vi "Beampointing_BELLA_PICObooster.vi"() -> ()   [LabVIEW 2013]
uses:
  shared programs/GUI_Template/GUI_master/tcp new data cluster.ctl
  <userlib>/_OpenG.lib/array/array.llb/Filter 1D Array with Scalar (String)__ogtk.vi
  <vilib>/Utility/file.llb/Write To Spreadsheet File (string).vi
  <vilib>/Utility/file.llb/Read From Spreadsheet File (string).vi
  <vilib>/Analysis/NI_AALBase.lvlib
  GUI_Beampointing_single_TRA/Ctrs/move.ctl
  Ctrs/beam detection.ctl
  <vilib>/vision/NI_Vision_Development_Module.lvlib
  shared programs/GUI_Template/GUI_master/tcp_new_data_event.ctl
panel:
  out "Array 3":sgl[](array[numeric])=[35.01637, 16.987305, 27.281555, 56.5656, 0.0, 12.310791, 0.0, 0.0, 0.0, 0.0, 0.0, 0.0]
  in  "save path":path=path "W:/BP_DATA"
  out "size(s) 6":i32=12
  out "config path":string="H:\\Software\\control-all-loasis\\Developers Version\\Interface\\builds\\GUIs\\GUI_Beampointing_PicoBooster\\20160427BELLA.cfg"
  out "motor refs 7":refnum<vi>[](array[refnum])
  out "Moving Y":string
  out "Moving X":string
  out "particles":T1(array[cluster])=[{"Area"=13625.0, "Number of Holes"=0.0, "Bounding Rect"={"Left"=100.0, "Top"=93.0, "Right"=241.0, "Bottom"=225.0}, "Center of Mass"={"X"=171.3850275229358, "Y"=158.37277064220183}, "Orientation"=31.450434142859965, "Dimensions"={"Width"=141.0, "Height"=132.0}}]
  out "motor refs 6":refnum<vi>[](array[refnum])
  out "millisecond timer value":u32=150056294
  out "motor refs 5":refnum<vi>[](array[refnum])
  out "appended path":path=path "C:/Users/loasis.BELLANET/Documents/000 Labview/Developers Version/Interface/GUI_Beampointing_multi/defaultDevices_PICObooster.txt"
  out "motor refs 4":refnum<vi>[](array[refnum])
  in  "active Axis ref 3":cluster{"Ref X":refnum<vi>, "Ref Y":refnum<vi>}
  out "motor refs 3":refnum<vi>[](array[refnum])
  in  "active man refs":cluster{"Ref X":refnum<vi>, "Ref Y":refnum<vi>}
  out "motor refs 2":refnum<vi>[](array[refnum])
  in  "Numeric":dbl=2.0
  out "Current State":string="Exit"
  in  "output cluster 2":T5 {"detection para"."smal para"."Measurement Parameter" items=["Center of Mass X", "Center of Mass Y", "First Pixel X", "First Pixel Y", "Bounding Rect Left", "Bounding Rect Top", "Bounding Rect Right", "Bounding Rect Bottom", "Max Feret Diameter Start X", "Max Feret Diameter Start Y", "Max Feret Diameter End X", "Max Feret Diameter End Y", "Max Horiz. Segment Length Left", "Max Horiz. Segment Length Right", "Max Horiz. Segment Length Row", "-", "Bounding Rect Width", "Bounding Rect Height", "Bounding Rect Diagonal", "Perimeter", "Convex Hull Perimeter", "Holes' Perimeter", "Max Feret Diameter", "Equivalent Ellipse Major Axis", "Equivalent Ellipse Minor Axis", "Equivalent Ellipse Minor Axis (Feret)", "Equivalent Rect Long Side", "Equivalent Rect Short Side", "Equivalent Rect Diagonal", "Equivalent Rect Short Side (Feret)", "Average Horiz. Segment Length", "Average Vert. Segment Length", "Hydraulic Radius", "Waddel Disk Diameter", "-", "Area", "Holes' Area", "Particle & Holes' Area", "Convex Hull Area", "Image Area", "-", "Number of Holes", "Number of Horiz. Segments", "Number of Vert. Segments", "-", "Orientation", "Max Feret Diameter Orientation", "-", "% Area/Image Area", "% Area/(Particle & Holes' Area)", "Ratio of Equivalent Ellipse Axes", "Ratio of Equivalent Rect Sides", "-", "Elongation Factor", "Compactness Factor", "Heywood Circularity Factor", "Type Factor", "-", "Sum X", "Sum Y", "Sum XX", "Sum XY", "Sum YY", "Sum XXX", "Sum XXY", "Sum XYY", "Sum YYY", "-", "Moment of Inertia XX", "Moment of Inertia XY", "Moment of Inertia YY", "Moment of Inertia XXX", "Moment of Inertia XXY", "Moment of Inertia XYY", "Moment of Inertia YYY", "Norm. Moment of Inertia XX", "Norm. Moment of Inertia XY", "Norm. Moment of Inertia YY", "Norm. Moment of Inertia XXX", "Norm. Moment of Inertia XXY", "Norm. Moment of Inertia XYY", "Norm. Moment of Inertia YYY", "Hu Moment 1", "Hu Moment 2", "Hu Moment 3", "Hu Moment 4", "Hu Moment 5", "Hu Moment 6", "Hu Moment 7"]; "detection para"."smal para"."Range Lower Value" format="%.2f"; "detection para"."smal para"."Range Upper Value" format="%.2f"; "detection para"."detection method" items=["clustering", "entropy", "metric", "moments", "inter-class variance"]; "detection para"."Filter" items=["No Filter", "Median Filter", "Low Pass Filter"]}
  out "CCDs":string[](array[string])=["RegenCam", "BoosterCam", "PreampCam", "Amp1Cam", "Amp2Cam", "Amp3Cam", "", "", "", "", "", ""]
  in  "GUIdevice 12":string
  in  "GUIdevice 11":string
  in  "GUIdevice 10":string
  in  "GUIdevice 9":string
  out "error out 2":errorcluster
  in  "active cams":string[](array[string])
  in  "Motor Y":dbl[][](array[numeric])
  in  "Motor X":dbl[][](array[numeric])
  out "Names":string[](array[string])=["device12", "device45", "", ""]
  in  "Offset X stats":dbl[][](array[numeric])
  in  "Offset Y stats":dbl[][](array[numeric])
  out "Box":T6(array[cluster])=[{"Left"=100.0, "Top"=93.0, "Right"=241.0, "Bottom"=225.0}, {"Left"=87.0, "Top"=22.0, "Right"=220.0, "Bottom"=185.0}, {"Left"=80.0, "Top"=37.0, "Right"=220.0, "Bottom"=176.0}, {"Left"=78.0, "Top"=52.0, "Right"=221.0, "Bottom"=209.0}, {"Left"=0.0, "Top"=0.0, "Right"=0.0, "Bottom"=0.0}]
  in  "Tab Control 2":enum32{"Config ", "Main", "History"}(tab)=enum."Main"
  in  "associated motors":T7={"Motor CCD 1"=0, "Motor CCD 2"=0, "Motor CCD 3"=1, "Motor CCD 4"=0, "Motor CCD 5"=0, "Motor CCD 6"=0, "Motor CCD 7"=0, "Motor CCD 8"=0, "Motor CCD 9"=0, "Motor CCD 10"=0, "Motor CCD 11"=0, "Motor CCD 12"=0} {"Motor CCD 12" items=["device12", "device45", "", ""]; "Motor CCD 11" items=["device12", "device45", "", ""]; "Motor CCD 10" items=["device12", "device45", "", ""]; "Motor CCD 9" items=["device12", "device45", "", ""]; "Motor CCD 8" items=["device12", "device45", "", ""]; "Motor CCD 7" items=["device12", "device45", "", ""]; "Motor CCD 6" items=["device12", "device45", "", ""]; "Motor CCD 5" items=["device12", "device45", "", ""]; "Motor CCD 4" items=["device12", "device45", "", ""]; "Motor CCD 3" items=["device12", "device45", "", ""]; "Motor CCD 2" items=["device12", "device45", "", ""]; "Motor CCD 1" items=["device12", "device45", "", ""]}
  out "Cameras":T8={"[0]"="RegenCam", "[1]"="BoosterCam", "[2]"="PreampCam", "[3]"="Amp1Cam", "[4]"="Amp2Cam", "[5]"="Amp3Cam", "[6]"="", "[7]"="", "[8]"="", "[8] 2"="", "[8] 3"="", "[8] 4"=""}
  out "Status":cluster{i32, i32, "Centroid X":dbl[][]}(graph)={0, 1, "Centroid X"=[[171.87383691112902, 0.0, 0.0], [153.80799798158193, 0.0, 0.0], [147.97157969527117, 0.0, 0.0], [147.97285865350722, 0.0, 0.0], [0.0, 0.0, 0.0], [0.0, 0.0, 0.0], [0.0, 0.0, 0.0], [0.0, 0.0, 0.0], [0.0, 0.0, 0.0], [0.0, 0.0, 0.0], [0.0, 0.0, 0.0], [0.0, 0.0, 0.0]]}
  in  "Exposure:12":dbl=0.095 min=0.0001 max=1.0 format="%#_6f"
  in  "Triggerdelay::12":dbl=0.003 min=0.0 max=0.09 format="%#_6f"
  in  "Exposure::11":dbl=0.095 min=0.0001 max=1.0 format="%#_6f"
  in  "Triggerdelay::11":dbl=0.003 min=0.0 max=0.09 format="%#_6f"
  in  "Exposure::10":dbl=0.095 min=0.0001 max=1.0 format="%#_6f"
  in  "Triggerdelay::10":dbl=0.003 min=0.0 max=0.09 format="%#_6f"
  in  "Exposure::9":dbl=0.095 min=0.0001 max=1.0 format="%#_6f"
  in  "Triggerdelay::9":dbl=0.003 min=0.0 max=0.09 format="%#_6f"
  in  "Trigger::9":bool
  in  "Trigger::10":bool caption="Trigger:10"
  in  "Trigger::11":bool
  in  "Trigger::12":bool
  in  "Target.Y::9":dbl=45.0 caption="T9y" min=0.0 max=2000.0 format="%#_6f"
  in  "Target.X::9":dbl=47.0 caption="Tx9" min=0.0 max=2000.0 format="%#_6f"
  in  "Target.Y::10":dbl=45.0 caption="T10y" min=0.0 max=2000.0 format="%#_6f"
  in  "Target.X::10":dbl=47.0 caption="T10x" min=0.0 max=2000.0 format="%#_6f"
  in  "Target.Y::11":dbl=45.0 caption="T11y" min=0.0 max=2000.0 format="%#_6f"
  in  "Target.X::11":dbl=47.0 caption="T11x" min=0.0 max=2000.0 format="%#_6f"
  in  "Target.Y::12":dbl=45.0 caption="T12y" min=0.0 max=2000.0 format="%#_6f"
  in  "Target.X::12":dbl=47.0 caption="T12x" min=0.0 max=2000.0 format="%#_6f"
  in  "Exposure::8":dbl=0.095 min=0.0001 max=1.0 format="%#_6f"
  in  "Triggerdelay::8":dbl=0.003 min=0.0 max=0.09 format="%#_6f"
  in  "Trigger::8":bool
  in  "Target.Y::8":dbl=45.0 caption="T8y" min=0.0 max=2000.0 format="%#_6f"
  in  "Target.X::8":dbl=47.0 caption="T8x" min=0.0 max=2000.0 format="%#_6f"
  in  "Target.Y::7":dbl=45.0 caption="T7x" min=0.0 max=2000.0 format="%#_6f"
  in  "Target.X::7":dbl=47.0 caption="T7y" min=0.0 max=2000.0 format="%#_6f"
  in  "Target.Y::6":dbl=142.0 caption="T6y" min=0.0 max=5000.0 format="%#_6f"
  in  "Target.X::6":dbl=123.0 caption="T6x" min=0.0 max=5000.0 format="%#_6f"
  in  "Target.Y::5":dbl=108.0 caption="T5y" min=0.0 max=5000.0 format="%#_6f"
  in  "Target.X::5":dbl=172.0 caption="T5x" min=0.0 max=5000.0 format="%#_6f"
  in  "Target.Y::4":dbl=130.0 caption="T4y" min=0.0 max=5000.0 format="%#_6f"
  in  "Target.X::4":dbl=148.0 caption="T4x" min=0.0 max=5000.0 format="%#_6f"
  in  "Target.Y::3":dbl=110.0 caption="T3y" min=0.0 max=5000.0 format="%#_6f"
  in  "Target.X::3":dbl=154.0 caption="T3x" min=0.0 max=5000.0 format="%#_6f"
  in  "Target.Y::2":dbl=106.0 caption="T2y" min=0.0 max=5000.0 format="%#_6f"
  in  "Target.X::2":dbl=163.0 caption="T2x" min=0.0 max=5000.0 format="%#_6f"
  in  "Target.Y::1":dbl=162.0 caption="T1y" min=0.0 max=5000.0 format="%#_6f"
  in  "Target.X::1":dbl=171.0 caption="T1x" min=0.0 max=5000.0 format="%#_6f"
  in  "Exposure::7":dbl=0.095 min=3.8e-05 max=1.0 format="%#_6f"
  in  "Triggerdelay::7":dbl=0.003 min=0.0 max=0.09 format="%#_6f"
  in  "Trigger::7":bool
  in  "Exposure::6":dbl=0.095 min=3.8e-05 max=1.0 format="%#_6f"
  in  "Triggerdelay::6":dbl=0.003 min=0.0 max=0.09 format="%#_6f"
  in  "Trigger::6":bool
  in  "Exposure::5":dbl=0.095 min=0.0001 max=1.0 format="%#_6f"
  in  "Triggerdelay::5":dbl=0.003 min=0.0 max=0.09 format="%#_6f"
  in  "Trigger::5":bool
  in  "Exposure::4":dbl=0.095 min=0.0001 max=1.0 format="%#_6f"
  in  "Triggerdelay::4":dbl=0.003 min=0.0 max=0.09 format="%#_6f"
  in  "Trigger::4":bool
  in  "Exposure::3":dbl=0.095 min=3.8e-05 max=1.0 format="%#_6f"
  in  "Triggerdelay::3":dbl=0.003 min=0.0 max=0.09 format="%#_6f"
  in  "Trigger::3":bool
  in  "Exposure::2":dbl=0.095 min=3.8e-05 max=1.0 format="%#_6f"
  in  "Triggerdelay::2":dbl=0.003 min=0.0 max=0.09 format="%#_6f"
  in  "Trigger::2":bool
  out "image::1":T9(plugin-control) caption="RegenCam"
  out "image::2":T9(plugin-control) caption="BoosterCam"
  out "image::3":T9(plugin-control) caption="PreampCam"
  out "image::4":T9(plugin-control) caption="Amp1Cam"
  out "image::5":T9(plugin-control) caption="Amp2Cam"
  out "image::6":T9(plugin-control) caption="Amp3Cam"
  out "image::7":T9(plugin-control)
  out "image::8":T9(plugin-control)
  in  "Exposure::1":dbl=0.095 min=3.8e-05 max=1.0 format="%#_6f"
  in  "Triggerdelay::1":dbl=0.003 min=0.0 max=0.09 format="%#_6f"
  in  "Trigger::1":bool
  in  "UDP error message":string
  out "required Y":bool[](array[boolean])=[FALSE, TRUE, FALSE, FALSE, FALSE]
  out "required X":bool[](array[boolean])=[FALSE, TRUE, FALSE, FALSE, FALSE]
  out "detected":bool[](array[boolean])=[TRUE, TRUE, TRUE, TRUE, FALSE]
  out "name array":string[](array[string])=["RegenCam", "BoosterCam", "PreampCam", "Amp1Cam", "Amp3Cam"]
  out "image::9":T9(plugin-control)
  out "image::10":T9(plugin-control)
  out "image::11":T9(plugin-control)
  out "image::12":T9(plugin-control)
  out "speedmode X":bool[](array[boolean])=[TRUE, TRUE, TRUE, TRUE, FALSE]
  out "speedmode Y":bool[](array[boolean])=[TRUE, FALSE, TRUE, TRUE, FALSE]
  out "CCD 9":cluster{timestamp[], dbl[]}[](graph)=[{[timestamp(3549547983.3591223 s since 1904-01-01)], [0.0]}, {[timestamp(3549547983.3591223 s since 1904-01-01)], [0.0]}, {[timestamp(3549547983.3591223 s since 1904-01-01)], [20.0]}, {[timestamp(3549547983.3591223 s since 1904-01-01)], [-20.0, -20.0, -20.0, -20.0]}]
  out "CCD 10":cluster{timestamp[], dbl[]}[](graph)=[{[timestamp(3549547983.360123 s since 1904-01-01)], [0.0]}, {[timestamp(3549547983.360123 s since 1904-01-01)], [0.0]}, {[timestamp(3549547983.360123 s since 1904-01-01)], [20.0]}, {[timestamp(3549547983.360123 s since 1904-01-01)], [-20.0, -20.0, -20.0, -20.0]}]
  out "CCD 11":cluster{timestamp[], dbl[]}[](graph)=[{[timestamp(3549547983.360123 s since 1904-01-01)], [0.0]}, {[timestamp(3549547983.360123 s since 1904-01-01)], [0.0]}, {[timestamp(3549547983.360123 s since 1904-01-01)], [20.0]}, {[timestamp(3549547983.360123 s since 1904-01-01)], [-20.0, -20.0, -20.0, -20.0]}]
  out "CCD 12":cluster{timestamp[], dbl[]}[](graph)=[{[timestamp(3549547983.360123 s since 1904-01-01)], [0.0]}, {[timestamp(3549547983.360123 s since 1904-01-01)], [0.0]}, {[timestamp(3549547983.360123 s since 1904-01-01)], [20.0]}, {[timestamp(3549547983.360123 s since 1904-01-01)], [-20.0, -20.0, -20.0, -20.0]}]
  out "CCD 5":cluster{timestamp[], dbl[]}[](graph)=[{[timestamp(3549547983.358122 s since 1904-01-01)], [0.0]}, {[timestamp(3549547983.358122 s since 1904-01-01)], [0.0]}, {[timestamp(3549547983.358122 s since 1904-01-01)], [20.0]}, {[timestamp(3549547983.358122 s since 1904-01-01)], [-20.0, -20.0, -20.0, -20.0]}]
  out "CCD 6":cluster{timestamp[], dbl[]}[](graph)=[{[timestamp(3549547983.3591223 s since 1904-01-01)], [0.0]}, {[timestamp(3549547983.3591223 s since 1904-01-01)], [0.0]}, {[timestamp(3549547983.3591223 s since 1904-01-01)], [20.0]}, {[timestamp(3549547983.3591223 s since 1904-01-01)], [-20.0, -20.0, -20.0, -20.0]}]
  out "CCD 7":cluster{timestamp[], dbl[]}[](graph)=[{[timestamp(3549547983.3591223 s since 1904-01-01)], [0.0]}, {[timestamp(3549547983.3591223 s since 1904-01-01)], [0.0]}, {[timestamp(3549547983.3591223 s since 1904-01-01)], [20.0]}, {[timestamp(3549547983.3591223 s since 1904-01-01)], [-20.0, -20.0, -20.0, -20.0]}]
  out "CCD 8":cluster{timestamp[], dbl[]}[](graph)=[{[timestamp(3549547983.3591223 s since 1904-01-01)], [0.0]}, {[timestamp(3549547983.3591223 s since 1904-01-01)], [0.0]}, {[timestamp(3549547983.3591223 s since 1904-01-01)], [20.0]}, {[timestamp(3549547983.3591223 s since 1904-01-01)], [-20.0, -20.0, -20.0, -20.0]}]
  out "CCD 2":cluster{timestamp[], dbl[]}[](graph)=[{[timestamp(3549547983.358122 s since 1904-01-01)], [3.0783937413765585]}, {[timestamp(3549547983.358122 s since 1904-01-01)], [8.883046862591215]}, {[timestamp(3549547983.358122 s since 1904-01-01)], [20.0]}, {[timestamp(3549547983.358122 s since 1904-01-01)], [-20.0, -20.0, -20.0, -20.0]}]
  out "CCD 1":cluster{timestamp[], dbl[]}[](graph)=[{[timestamp(3549547983.357121 s since 1904-01-01)], [3.1654865062995725]}, {[timestamp(3549547983.357121 s since 1904-01-01)], [-0.42630614615123363]}, {[timestamp(3549547983.357121 s since 1904-01-01)], [20.0]}, {[timestamp(3549547983.357121 s since 1904-01-01)], [-20.0, -20.0, -20.0, -20.0]}]
  out "CCD 3":cluster{timestamp[], dbl[]}[](graph)=[{[timestamp(3549547983.358122 s since 1904-01-01)], [5.607599326451648]}, {[timestamp(3549547983.358122 s since 1904-01-01)], [4.73033759911138]}, {[timestamp(3549547983.358122 s since 1904-01-01)], [0.0]}, {[timestamp(3549547983.358122 s since 1904-01-01)], [0.0, 0.0, 0.0, 0.0]}]
  out "CCD 4":cluster{timestamp[], dbl[]}[](graph)=[{[timestamp(3549547983.358122 s since 1904-01-01)], [1.2734976836249814]}, {[timestamp(3549547983.358122 s since 1904-01-01)], [-0.6350086940318818]}, {[timestamp(3549547983.358122 s since 1904-01-01)], [20.0]}, {[timestamp(3549547983.358122 s since 1904-01-01)], [-20.0, -20.0, -20.0, -20.0]}]
  in  "History Size":i32=2000
  out "History Index":i32=1
  in  "Feedback Global":bool
  in  "detection para":T3[](array[typedef])=[{"Filter"=1, "Filter Para"={"X Size"=5, "Y Size"=5, "% Tolerance"=1}, "detection method"=4, "smal para"=[{"Measurement Parameter"=35, "Range Lower Value"=0.0, "Range Upper Value"=0.0, "Range"=TRUE, "Measurement Type"=FALSE}], "Remove small Objects"=TRUE, "Restrict to round Objects"=FALSE}, {"Filter"=1, "Filter Para"={"X Size"=5, "Y Size"=5, "% Tolerance"=1}, "detection method"=4, "smal para"=[{"Measurement Parameter"=35, "Range Lower Value"=0.0, "Range Upper Value"=500.0, "Range"=FALSE, "Measurement Type"=FALSE}], "Remove small Objects"=TRUE, "Restrict to round Objects"=FALSE}, {"Filter"=1, "Filter Para"={"X Size"=5, "Y Size"=5, "% Tolerance"=1}, "detection method"=4, "smal para"=[{"Measurement Parameter"=35, "Range Lower Value"=0.0, "Range Upper Value"=500.0, "Range"=TRUE, "Measurement Type"=FALSE}], "Remove small Objects"=TRUE, "Restrict to round Objects"=FALSE}, {"Filter"=1, "Filter Para"={"X Size"=5, "Y Size"=5, "% Tolerance"=1}, "detection method"=4, "smal para"=[{"Measurement Parameter"=35, "Range Lower Value"=0.0, "Range Upper Value"=500.0, "Range"=TRUE, "Measurement Type"=FALSE}], "Remove small Objects"=TRUE, "Restrict to round Objects"=FALSE}, {"Filter"=1, "Filter Para"={"X Size"=5, "Y Size"=5, "% Tolerance"=1}, "detection method"=4, "smal para"=[{"Measurement Parameter"=35, "Range Lower Value"=0.0, "Range Upper Value"=500.0, "Range"=TRUE, "Measurement Type"=FALSE}], "Remove small Objects"=TRUE, "Restrict to round Objects"=FALSE}, {"Filter"=1, "Filter Para"={"X Size"=5, "Y Size"=5, "% Tolerance"=1}, "detection method"=4, "smal para"=[{"Measurement Parameter"=35, "Range Lower Value"=0.0, "Range Upper Value"=500.0, "Range"=TRUE, "Measurement Type"=FALSE}], "Remove small Objects"=TRUE, "Restrict to round Objects"=FALSE}, {"Filter"=1, "Filter Para"={"X Size"=5, "Y Size"=5, "% Tolerance"=1}, "detection method"=4, "smal para"=[{"Measurement Parameter"=35, "Range Lower Value"=0.0, "Range Upper Value"=500.0, "Range"=TRUE, "Measurement Type"=FALSE}], "Remove small Objects"=TRUE, "Restrict to round Objects"=FALSE}, {"Filter"=1, "Filter Para"={"X Size"=5, "Y Size"=5, "% Tolerance"=1}, "detection method"=3, "smal para"=[{"Measurement Parameter"=35, "Range Lower Value"=0.0, "Range Upper Value"=0.0, "Range"=FALSE, "Measurement Type"=FALSE}], "Remove small Objects"=TRUE, "Restrict to round Objects"=FALSE}, {"Filter"=1, "Filter Para"={"X Size"=5, "Y Size"=5, "% Tolerance"=1}, "detection method"=4, "smal para"=[{"Measurement Parameter"=35, "Range Lower Value"=0.0, "Range Upper Value"=0.0, "Range"=FALSE, "Measurement Type"=FALSE}], "Remove small Objects"=TRUE, "Restrict to round Objects"=FALSE}, {"Filter"=1, "Filter Para"={"X Size"=5, "Y Size"=5, "% Tolerance"=1}, "detection method"=4, "smal para"=[{"Measurement Parameter"=35, "Range Lower Value"=0.0, "Range Upper Value"=500.0, "Range"=TRUE, "Measurement Type"=FALSE}], "Remove small Objects"=TRUE, "Restrict to round Objects"=FALSE}, {"Filter"=1, "Filter Para"={"X Size"=5, "Y Size"=5, "% Tolerance"=1}, "detection method"=4, "smal para"=[{"Measurement Parameter"=35, "Range Lower Value"=0.0, "Range Upper Value"=500.0, "Range"=TRUE, "Measurement Type"=FALSE}], "Remove small Objects"=TRUE, "Restrict to round Objects"=FALSE}, {"Filter"=1, "Filter Para"={"X Size"=5, "Y Size"=5, "% Tolerance"=1}, "detection method"=4, "smal para"=[{"Measurement Parameter"=35, "Range Lower Value"=0.0, "Range Upper Value"=500.0, "Range"=TRUE, "Measurement Type"=FALSE}], "Remove small Objects"=TRUE, "Restrict to round Objects"=FALSE}] {"smal para"."Measurement Parameter" items=["Center of Mass X", "Center of Mass Y", "First Pixel X", "First Pixel Y", "Bounding Rect Left", "Bounding Rect Top", "Bounding Rect Right", "Bounding Rect Bottom", "Max Feret Diameter Start X", "Max Feret Diameter Start Y", "Max Feret Diameter End X", "Max Feret Diameter End Y", "Max Horiz. Segment Length Left", "Max Horiz. Segment Length Right", "Max Horiz. Segment Length Row", "-", "Bounding Rect Width", "Bounding Rect Height", "Bounding Rect Diagonal", "Perimeter", "Convex Hull Perimeter", "Holes' Perimeter", "Max Feret Diameter", "Equivalent Ellipse Major Axis", "Equivalent Ellipse Minor Axis", "Equivalent Ellipse Minor Axis (Feret)", "Equivalent Rect Long Side", "Equivalent Rect Short Side", "Equivalent Rect Diagonal", "Equivalent Rect Short Side (Feret)", "Average Horiz. Segment Length", "Average Vert. Segment Length", "Hydraulic Radius", "Waddel Disk Diameter", "-", "Area", "Holes' Area", "Particle & Holes' Area", "Convex Hull Area", "Image Area", "-", "Number of Holes", "Number of Horiz. Segments", "Number of Vert. Segments", "-", "Orientation", "Max Feret Diameter Orientation", "-", "% Area/Image Area", "% Area/(Particle & Holes' Area)", "Ratio of Equivalent Ellipse Axes", "Ratio of Equivalent Rect Sides", "-", "Elongation Factor", "Compactness Factor", "Heywood Circularity Factor", "Type Factor", "-", "Sum X", "Sum Y", "Sum XX", "Sum XY", "Sum YY", "Sum XXX", "Sum XXY", "Sum XYY", "Sum YYY", "-", "Moment of Inertia XX", "Moment of Inertia XY", "Moment of Inertia YY", "Moment of Inertia XXX", "Moment of Inertia XXY", "Moment of Inertia XYY", "Moment of Inertia YYY", "Norm. Moment of Inertia XX", "Norm. Moment of Inertia XY", "Norm. Moment of Inertia YY", "Norm. Moment of Inertia XXX", "Norm. Moment of Inertia XXY", "Norm. Moment of Inertia XYY", "Norm. Moment of Inertia YYY", "Hu Moment 1", "Hu Moment 2", "Hu Moment 3", "Hu Moment 4", "Hu Moment 5", "Hu Moment 6", "Hu Moment 7"]; "smal para"."Range Lower Value" format="%.2f"; "smal para"."Range Upper Value" format="%.2f"; "detection method" items=["clustering", "entropy", "metric", "moments", "inter-class variance"]; "Filter" items=["No Filter", "Median Filter", "Low Pass Filter"]}
  in  "GUIdevice 8":string
  in  "Tab Control":T10(tab)
  in  "new tdms":bool
  in  "Save Stats":bool
  in  "Save Config":bool
  in  "Load Config":bool
  in  "update speed [ms]":i32=2000
  in  "img to avg":i32=6 min=3 max=200
  in  "Reset History":bool
  in  "autodetect":bool
  in  "Detection Rate":dbl=0.8 min=0.001 max=1.0
  in  "Center":bool
  in  "Align":bool
  in  "Speedmode @":dbl=3.0 min=1.0 max=20.0
  in  "device ini":bool
  in  "beam detection para":T3={"Filter"=1, "Filter Para"={"X Size"=5, "Y Size"=5, "% Tolerance"=1}, "detection method"=4, "smal para"=[{"Measurement Parameter"=35, "Range Lower Value"=0.0, "Range Upper Value"=500.0, "Range"=FALSE, "Measurement Type"=FALSE}], "Remove small Objects"=TRUE, "Restrict to round Objects"=FALSE} {"smal para"."Measurement Parameter" items=["Center of Mass X", "Center of Mass Y", "First Pixel X", "First Pixel Y", "Bounding Rect Left", "Bounding Rect Top", "Bounding Rect Right", "Bounding Rect Bottom", "Max Feret Diameter Start X", "Max Feret Diameter Start Y", "Max Feret Diameter End X", "Max Feret Diameter End Y", "Max Horiz. Segment Length Left", "Max Horiz. Segment Length Right", "Max Horiz. Segment Length Row", "-", "Bounding Rect Width", "Bounding Rect Height", "Bounding Rect Diagonal", "Perimeter", "Convex Hull Perimeter", "Holes' Perimeter", "Max Feret Diameter", "Equivalent Ellipse Major Axis", "Equivalent Ellipse Minor Axis", "Equivalent Ellipse Minor Axis (Feret)", "Equivalent Rect Long Side", "Equivalent Rect Short Side", "Equivalent Rect Diagonal", "Equivalent Rect Short Side (Feret)", "Average Horiz. Segment Length", "Average Vert. Segment Length", "Hydraulic Radius", "Waddel Disk Diameter", "-", "Area", "Holes' Area", "Particle & Holes' Area", "Convex Hull Area", "Image Area", "-", "Number of Holes", "Number of Horiz. Segments", "Number of Vert. Segments", "-", "Orientation", "Max Feret Diameter Orientation", "-", "% Area/Image Area", "% Area/(Particle & Holes' Area)", "Ratio of Equivalent Ellipse Axes", "Ratio of Equivalent Rect Sides", "-", "Elongation Factor", "Compactness Factor", "Heywood Circularity Factor", "Type Factor", "-", "Sum X", "Sum Y", "Sum XX", "Sum XY", "Sum YY", "Sum XXX", "Sum XXY", "Sum XYY", "Sum YYY", "-", "Moment of Inertia XX", "Moment of Inertia XY", "Moment of Inertia YY", "Moment of Inertia XXX", "Moment of Inertia XXY", "Moment of Inertia XYY", "Moment of Inertia YYY", "Norm. Moment of Inertia XX", "Norm. Moment of Inertia XY", "Norm. Moment of Inertia YY", "Norm. Moment of Inertia XXX", "Norm. Moment of Inertia XXY", "Norm. Moment of Inertia XYY", "Norm. Moment of Inertia YYY", "Hu Moment 1", "Hu Moment 2", "Hu Moment 3", "Hu Moment 4", "Hu Moment 5", "Hu Moment 6", "Hu Moment 7"]; "smal para"."Range Lower Value" format="%.2f"; "smal para"."Range Upper Value" format="%.2f"; "detection method" items=["clustering", "entropy", "metric", "moments", "inter-class variance"]; "Filter" items=["No Filter", "Median Filter", "Low Pass Filter"]}
  in  "move config":T2={"Tolerance [%]"=0.1, "Stepsize"=0.0001, "Invert Axis"=TRUE, "Invert Direction X"=FALSE, "Invert Direction Y"=TRUE, "enable feedback"=FALSE, "Set Centriod Target"=FALSE}
  in  "Position 2":dbl=-20.0 caption="Stepsize" min=0.0 max=999999.0 format="%_6f"
  in  "Position 1":dbl=20.0 caption="Stepsize" min=0.0 max=999999.0 format="%_6f"
  in  "Right":bool caption="RelativeMove.Axis 1.CCW::1"
  in  "Left":bool caption="RelativeMove.Axis 1.CW::1"
  in  "Down":bool caption="RelativeMove.Axis. 2.CCW::1"
  in  "Up":bool caption="RelativeMove.Axis 2.CW::1"
  in  "StepSize":i16=5 caption="Stepsize" min=0 max=500 step=1
  in  "active axis refs 2":T11(array[cluster])
  in  "active Axis ref":cluster{"Ref X":refnum<vi>, "Ref Y":refnum<vi>}
  in  "CCDs":u16(ring) items=["RegenCam", "BoosterCam", "PreampCam", "Amp1Cam", "Amp2Cam", "Amp3Cam", "", "", "", "", "", ""]
  out "motor refs":refnum<vi>[](array[refnum])
  in  "Position.device 4::99":dbl caption="Motor Axis 1" min=-1000.0 max=1000.0 format="%#_6f"
  in  "Position.device 5::99":dbl caption="Motor Axis 1" min=-1000.0 max=1000.0 format="%#_6f"
  in  "Position.device 2::99":dbl=-20.0 caption="Motor Axis 1" min=-10000.0 max=10000.0 format="%#_6f"
  in  "Position.device 1::99":dbl=20.0 caption="Motor Axis 1" min=-10000.0 max=10000.0 format="%#_6f"
  in  "GUIdevice 99":string="LB-Pico-Booster"
  in  "move properties":T2[](array[typedef])=[{"Tolerance [%]"=0.1, "Stepsize"=0.0001, "Invert Axis"=TRUE, "Invert Direction X"=FALSE, "Invert Direction Y"=TRUE, "enable feedback"=FALSE, "Set Centriod Target"=FALSE}, {"Tolerance [%]"=0.1, "Stepsize"=0.0001, "Invert Axis"=TRUE, "Invert Direction X"=FALSE, "Invert Direction Y"=TRUE, "enable feedback"=FALSE, "Set Centriod Target"=FALSE}, {"Tolerance [%]"=0.1, "Stepsize"=0.0001, "Invert Axis"=TRUE, "Invert Direction X"=FALSE, "Invert Direction Y"=TRUE, "enable feedback"=FALSE, "Set Centriod Target"=FALSE}, {"Tolerance [%]"=0.1, "Stepsize"=0.0001, "Invert Axis"=TRUE, "Invert Direction X"=FALSE, "Invert Direction Y"=TRUE, "enable feedback"=FALSE, "Set Centriod Target"=FALSE}, {"Tolerance [%]"=0.1, "Stepsize"=0.0001, "Invert Axis"=TRUE, "Invert Direction X"=FALSE, "Invert Direction Y"=TRUE, "enable feedback"=FALSE, "Set Centriod Target"=FALSE}, {"Tolerance [%]"=0.1, "Stepsize"=0.0001, "Invert Axis"=TRUE, "Invert Direction X"=FALSE, "Invert Direction Y"=TRUE, "enable feedback"=FALSE, "Set Centriod Target"=FALSE}, {"Tolerance [%]"=0.1, "Stepsize"=0.0001, "Invert Axis"=TRUE, "Invert Direction X"=FALSE, "Invert Direction Y"=TRUE, "enable feedback"=FALSE, "Set Centriod Target"=FALSE}, {"Tolerance [%]"=0.1, "Stepsize"=0.0001, "Invert Axis"=TRUE, "Invert Direction X"=FALSE, "Invert Direction Y"=TRUE, "enable feedback"=FALSE, "Set Centriod Target"=FALSE}, {"Tolerance [%]"=0.1, "Stepsize"=0.0001, "Invert Axis"=TRUE, "Invert Direction X"=FALSE, "Invert Direction Y"=TRUE, "enable feedback"=FALSE, "Set Centriod Target"=FALSE}, {"Tolerance [%]"=0.1, "Stepsize"=0.0001, "Invert Axis"=TRUE, "Invert Direction X"=FALSE, "Invert Direction Y"=TRUE, "enable feedback"=FALSE, "Set Centriod Target"=FALSE}, {"Tolerance [%]"=0.1, "Stepsize"=0.0001, "Invert Axis"=TRUE, "Invert Direction X"=FALSE, "Invert Direction Y"=TRUE, "enable feedback"=FALSE, "Set Centriod Target"=FALSE}, {"Tolerance [%]"=0.1, "Stepsize"=0.0001, "Invert Axis"=TRUE, "Invert Direction X"=FALSE, "Invert Direction Y"=TRUE, "enable feedback"=FALSE, "Set Centriod Target"=FALSE}, {"Tolerance [%]"=0.1, "Stepsize"=0.0001, "Invert Axis"=TRUE, "Invert Direction X"=FALSE, "Invert Direction Y"=TRUE, "enable feedback"=FALSE, "Set Centriod Target"=FALSE}]
  in  "Time":timestamp[][](array[timestamp])
  in  "Mean Size":dbl[][](array[numeric])
  in  "Size":dbl[][](array[numeric])
  in  "active CCDs":i32(listbox)=-1
  in  "Offset Y":dbl[][](array[numeric])
  in  "Offset X":dbl[][](array[numeric])
  in  "Mean Centroid X":dbl[][](array[numeric])
  in  "Mean Centroid Y":dbl[][](array[numeric])
  in  "Centroid Y":dbl[][](array[numeric])
  in  "Centroid X":dbl[][](array[numeric])
  in  "GUIdevice 7":string
  in  "GUIdevice 6":string="Amp3Cam"
  in  "GUIdevice 5":string="Amp2Cam"
  in  "GUIdevice 4":string="Amp1Cam"
  in  "GUIdevice 3":string="PreampCam"
  in  "GUIdevice 2":string="BoosterCam"
  in  "insert tag":bool=TRUE
  in  "stop":bool
  in  "GUIdevice 1":string="RegenCam"
  out "tcp data event":T12
  out "error IO 2":errorcluster
  # "x [Tolerance]"
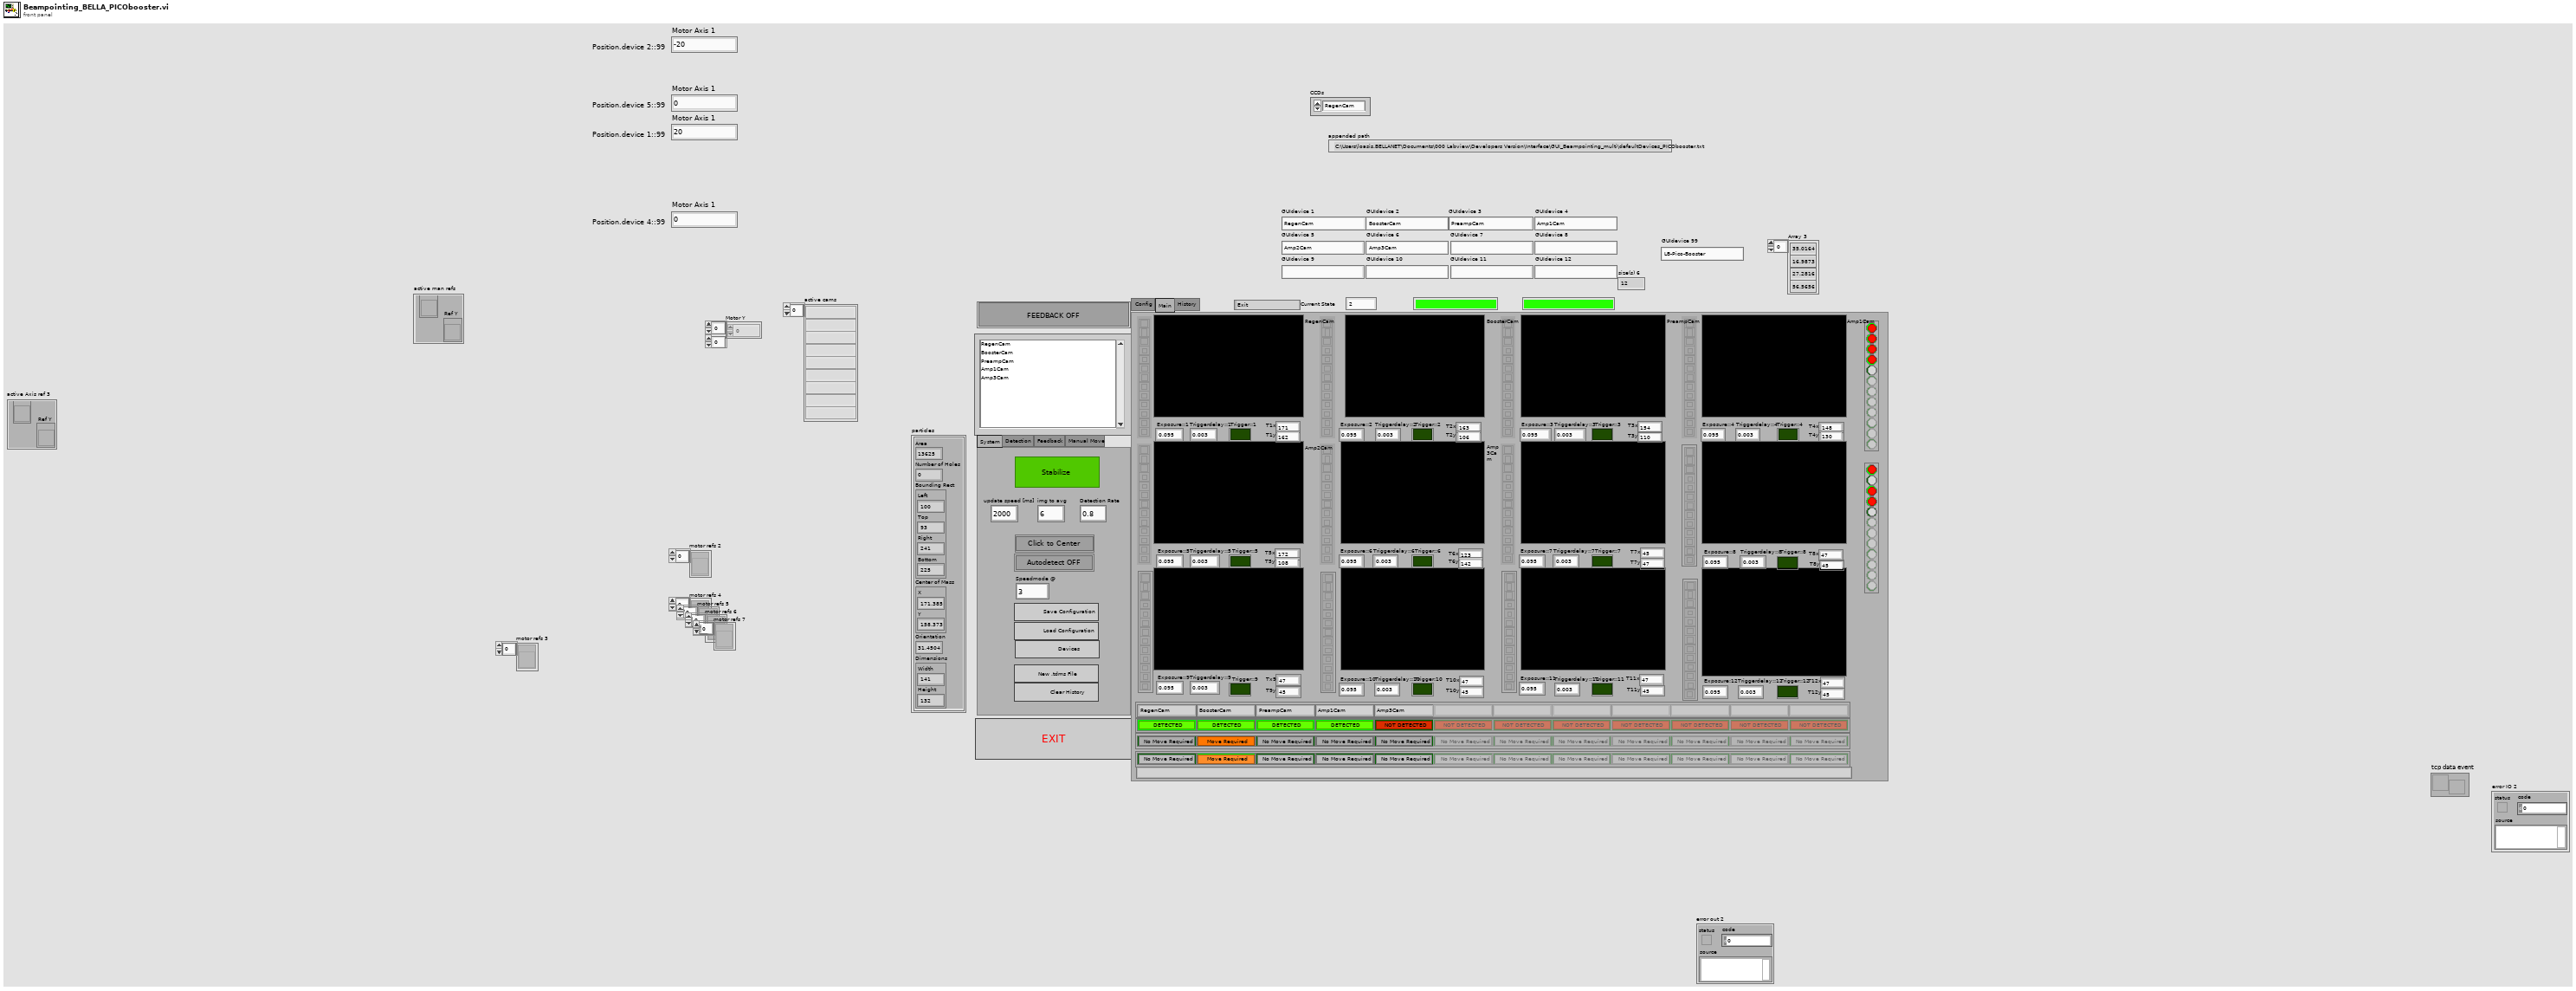
[diagram p1: front panel]
types:
  T1 = cluster{"Area":dbl, "Number of Holes":dbl, "Bounding Rect":cluster{"Left":dbl, "Top":dbl, "Right":dbl, "Bottom":dbl}, "Center of Mass":cluster{"X":dbl, "Y":dbl}, "Orientation":dbl, "Dimensions":cluster{"Width":dbl, "Height":dbl}}[]
  T2 = typedef "move.ctl" = cluster{"Tolerance [%]":dbl, "Stepsize":dbl, "Invert Axis":bool, "Invert Direction X":bool, "Invert Direction Y":bool, "enable feedback":bool, "Set Centriod Target":bool}
  T3 = typedef "beam detection.ctl" = cluster{"Filter":u16, "Filter Para":cluster{"X Size":i32, "Y Size":i32, "% Tolerance":i32}, "detection method":i32, "smal para":cluster{"Measurement Parameter":T4, "Range Lower Value":dbl, "Range Upper Value":dbl, "Range":bool, "Measurement Type":bool}[], "Remove small Objects":bool, "Restrict to round Objects":bool}
  T4 = typedef "Particle Parameters" = i32
  T5 = cluster{"CCDs":string[], "move properties":T2[], "detection para":T3[], "thresholds":cluster{"Lower value":sgl, "Upper value":sgl}[], "Value":cluster{"Motor CCD 1":u16, "Motor CCD 2":u16, "Motor CCD 3":u16, "Motor CCD 4":u16, "Motor CCD 5":u16, "Motor CCD 6":u16, "Motor CCD 7":u16, "Motor CCD 8":u16, "Motor CCD 9":u16, "Motor CCD 10":u16, "Motor CCD 11":u16, "Motor CCD 12":u16}}
  T6 = cluster{"Left":dbl, "Top":dbl, "Right":dbl, "Bottom":dbl}[]
  T7 = cluster{"Motor CCD 1":u16, "Motor CCD 2":u16, "Motor CCD 3":u16, "Motor CCD 4":u16, "Motor CCD 5":u16, "Motor CCD 6":u16, "Motor CCD 7":u16, "Motor CCD 8":u16, "Motor CCD 9":u16, "Motor CCD 10":u16, "Motor CCD 11":u16, "Motor CCD 12":u16}
  T8 = cluster{"[0]":string, "[1]":string, "[2]":string, "[3]":string, "[4]":string, "[5]":string, "[6]":string, "[7]":string, "[8]":string, "[8] 2":string, "[8] 3":string, "[8] 4":string}
  T9 = typedef "IMAQ Image.ctl" = refnum<image>
  T10 = enum32{"System", "Detection", "Feedback", "Manual Move"}
  T11 = cluster{"Ref X":refnum<vi>, "Ref Y":refnum<vi>}[]
  T12 = typedef "tcp_new_data_event.ctl" = refnum<user-event>
  T13 = typedef "tcp new data cluster.ctl" = cluster{"EventEnum":enum16{"new data", "connection status update"}, "Device name":string}
  T14 = cluster{"Left":i32, "Top":i32, "Right":i32, "Bottom":i32}
  T15 = enum32{"invalid app kind", "Development System", "Run Time System", "Student Edition", "Embedded LabVIEW", "Evaluation", "Custom"}
  T16 = enum16{"open", "open or create", "create or replace", "create", "open (read-only)"}
  T17 = enum32{"Invalid", "Standard", "Closed", "Hidden", "Minimized", "Maximized"}
  T18 = enum16{"open", "replace", "create", "open or create", "replace or create", "replace or create with confirmation"}
  T19 = enum8{"Enabled", "Disabled", "Disabled and Grayed Out"}
  T20 = typedef "Image Type" = u32
  T21 = cluster{"[0]":string, "[1]":string, "[2]":string, "[3]":string, "[4]":string, "[5]":string, "[6]":string, "[7]":string, "[8]":string, "[9]":string, "[10]":string, "[11]":string}
  T22 = cluster{"Target.X::1":refnum<vi>, "Target.Y::1":refnum<vi>}
  T23 = cluster{"Target.X::2":refnum<vi>, "Target.Y::2":refnum<vi>}
  T24 = cluster{"Target.X::3":refnum<vi>, "Target.Y::3":refnum<vi>}
  T25 = cluster{"Target.X::4":refnum<vi>, "Target.Y::4":refnum<vi>}
  T26 = cluster{"Target.X::5":refnum<vi>, "Target.Y::5":refnum<vi>}
  T27 = cluster{"Target.X::6":refnum<vi>, "Target.Y::6":refnum<vi>}
  T28 = cluster{"Target.X::7":refnum<vi>, "Target.Y::7":refnum<vi>}
  T29 = cluster{"Target.X::8":refnum<vi>, "Target.Y::8":refnum<vi>}
  T30 = cluster{"Target.X::12":refnum<vi>, "Target.Y::12":refnum<vi>}
  T31 = cluster{"Target.X::9":refnum<vi>, "Target.Y::9":refnum<vi>}
  T32 = cluster{"Target.X::10":refnum<vi>, "Target.Y::10":refnum<vi>}
  T33 = cluster{"Target.X::11":refnum<vi>, "Target.Y::11":refnum<vi>}
  T34 = cluster{"Target.X::12":refnum<vi>, "Target.Y::12":refnum<vi>}[]
  T35 = cluster{"Left":dbl, "Top":dbl, "Right":dbl, "Bottom":dbl}
  T36 = cluster{"Core":cluster{"Current VI Reference":refnum<vi>, "Close Panel on Exit?":bool}, "detection para":T3[], "thresholds":cluster{"Lower value":sgl, "Upper value":sgl}[], "Centroid X":dbl[][], "Centroid Y":dbl[][], "img to avg":i32, "Mean Centroid X":dbl[][], "Mean Centroid Y":dbl[][], "Offset X":dbl[][], "Offset Y":dbl[][], "Offset X stats ":dbl[][], "Offset Y stats ":dbl[][], "Size":dbl[][], "Mean Size":dbl[][], "Time":timestamp[][], "move properties":T2[], "active axis refs 2":cluster{"Ref X":refnum<vi>, "Ref Y":refnum<vi>}[], "active ccd":i32, "Feedback global":bool, "Motor X":dbl[][], "Motor Y":dbl[][], "active cams":string[], "Data Value Reference out":refnum<k34>, "active man refs":cluster{"Ref X":refnum<vi>, "Ref Y":refnum<vi>}, "detected":bool[], "speedmode X":bool[], "speedmode Y":bool[]}
  T37 = cluster{"Current VI Reference":refnum<vi>, "Close Panel on Exit?":bool}
  T38 = cluster{"appended array":timestamp[], "appended array":dbl[]}
  T39 = cluster{"appended array":timestamp[], "appended array":dbl[]}[]
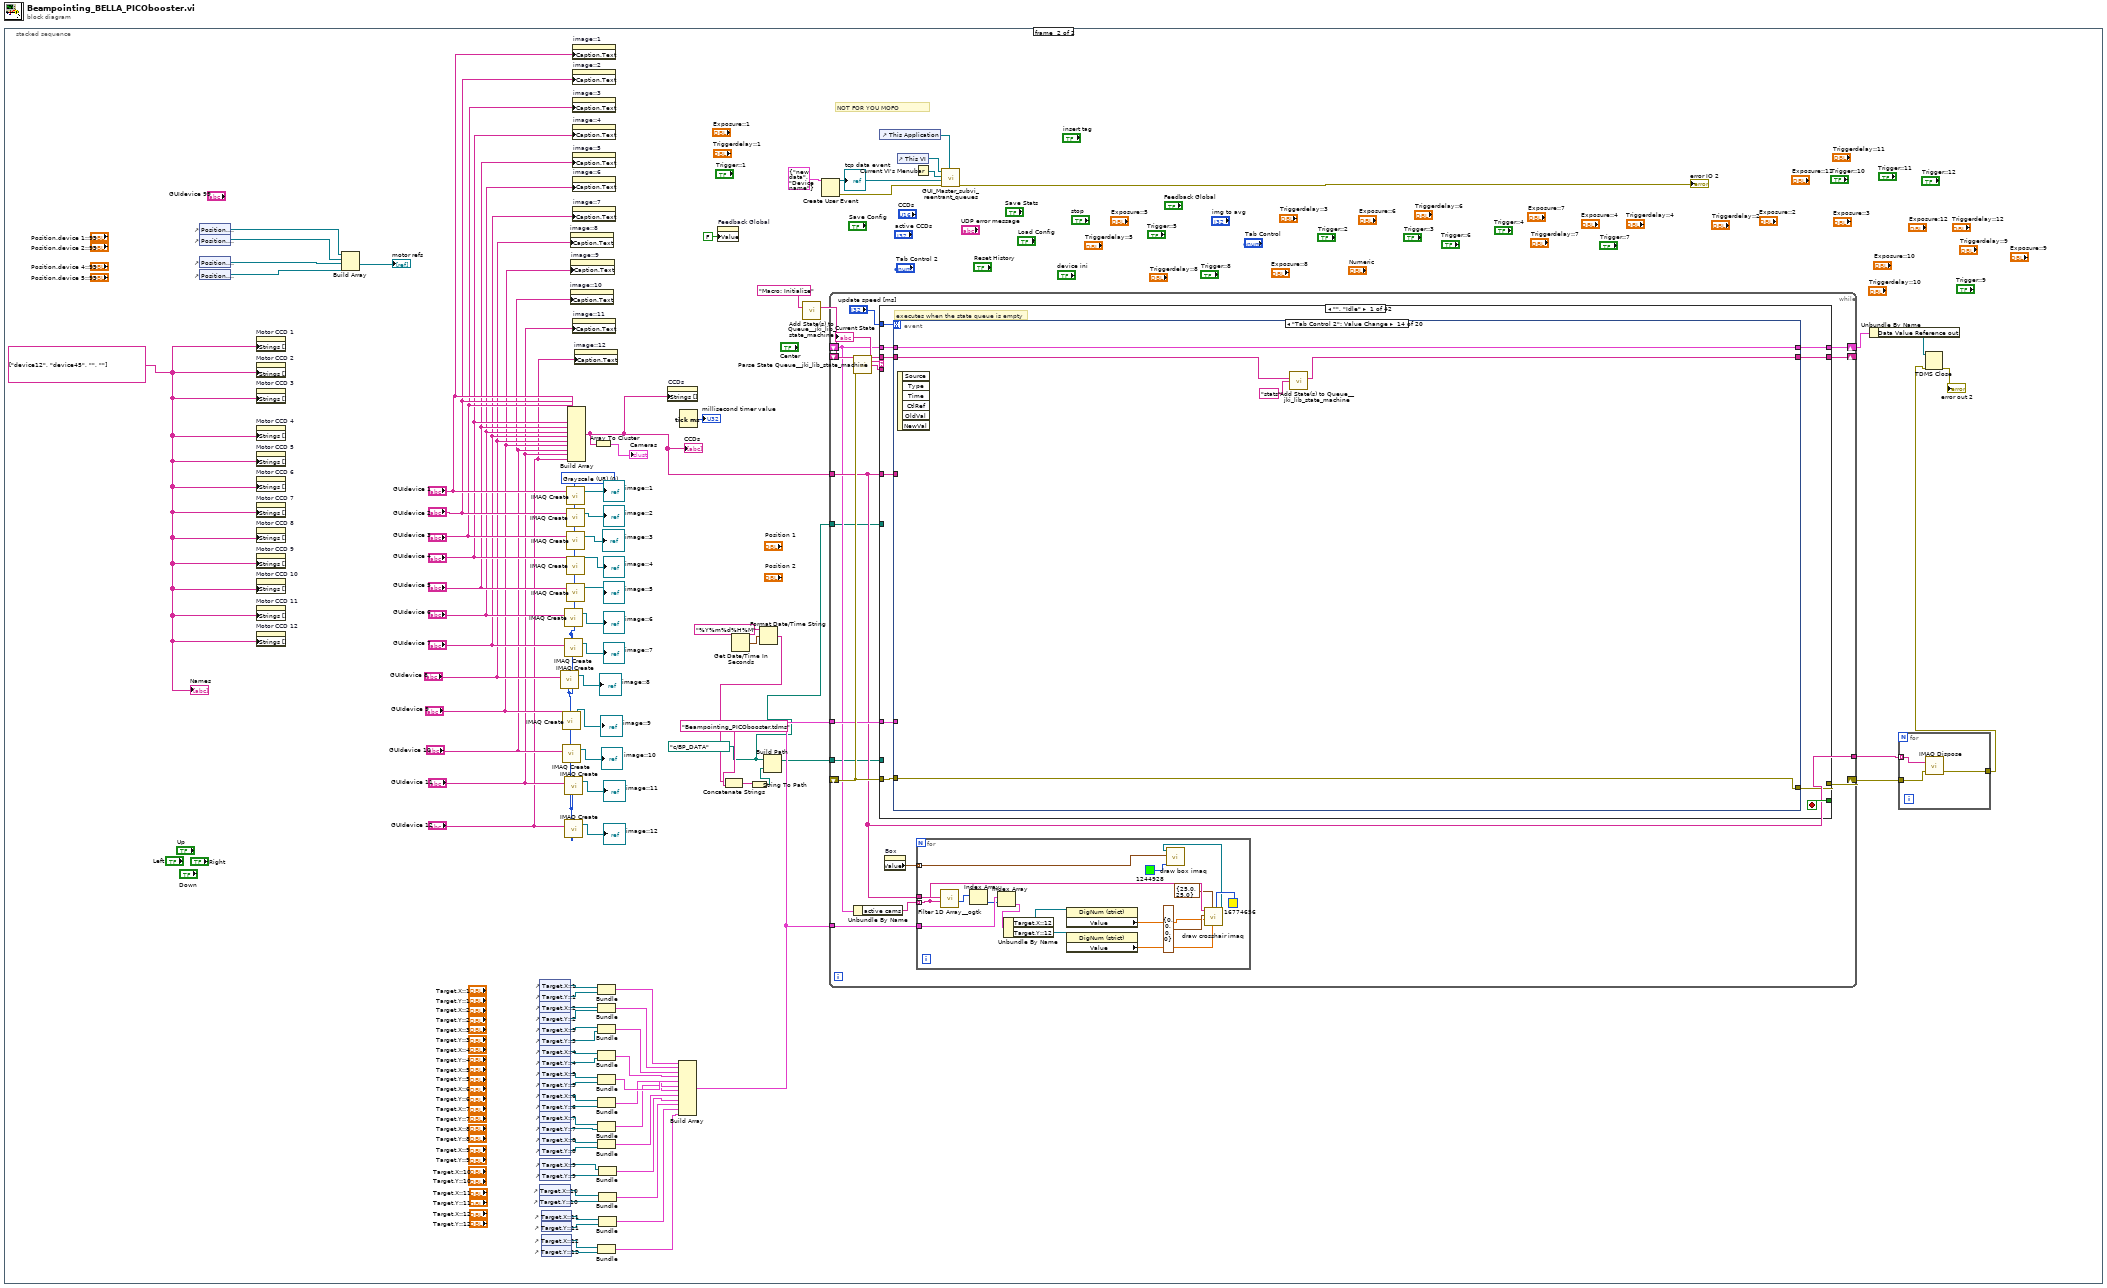
[diagram p0: block diagram]
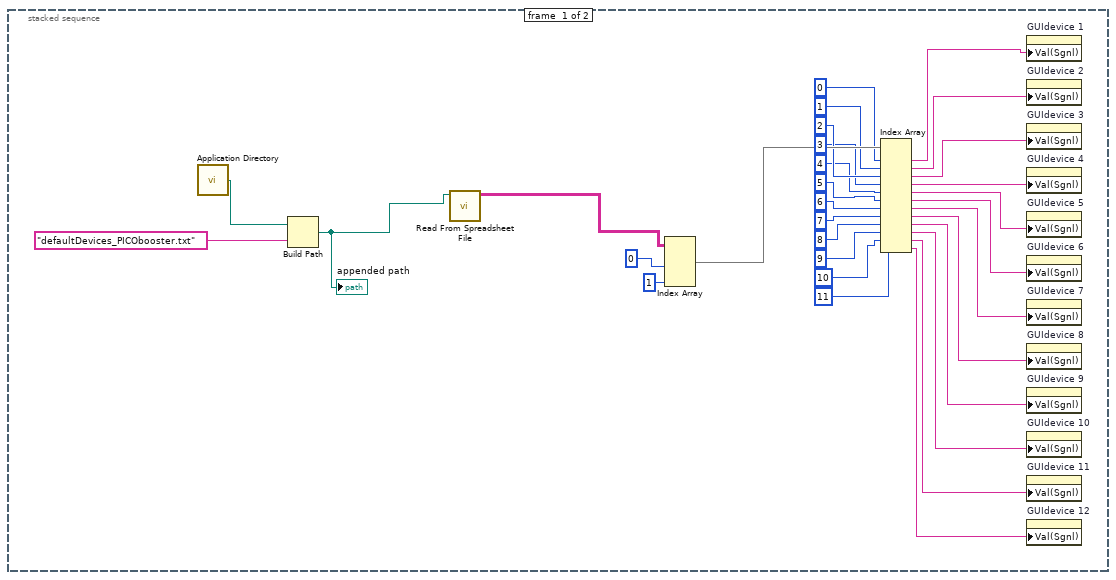
[diagram p2: hidden frame]
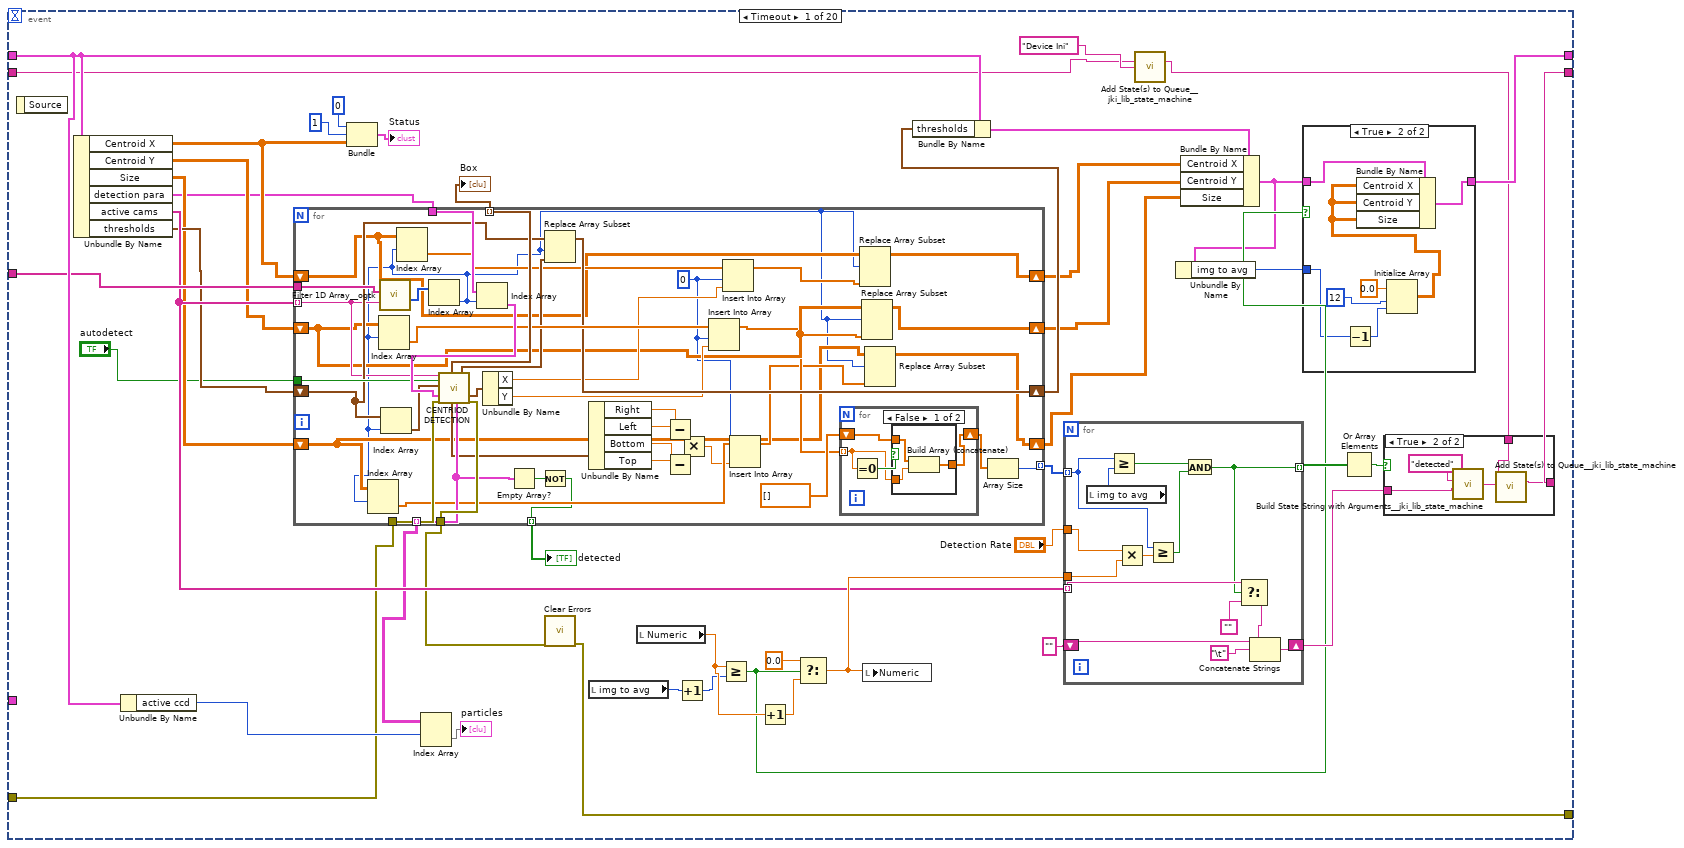
[diagram p3: hidden frame]
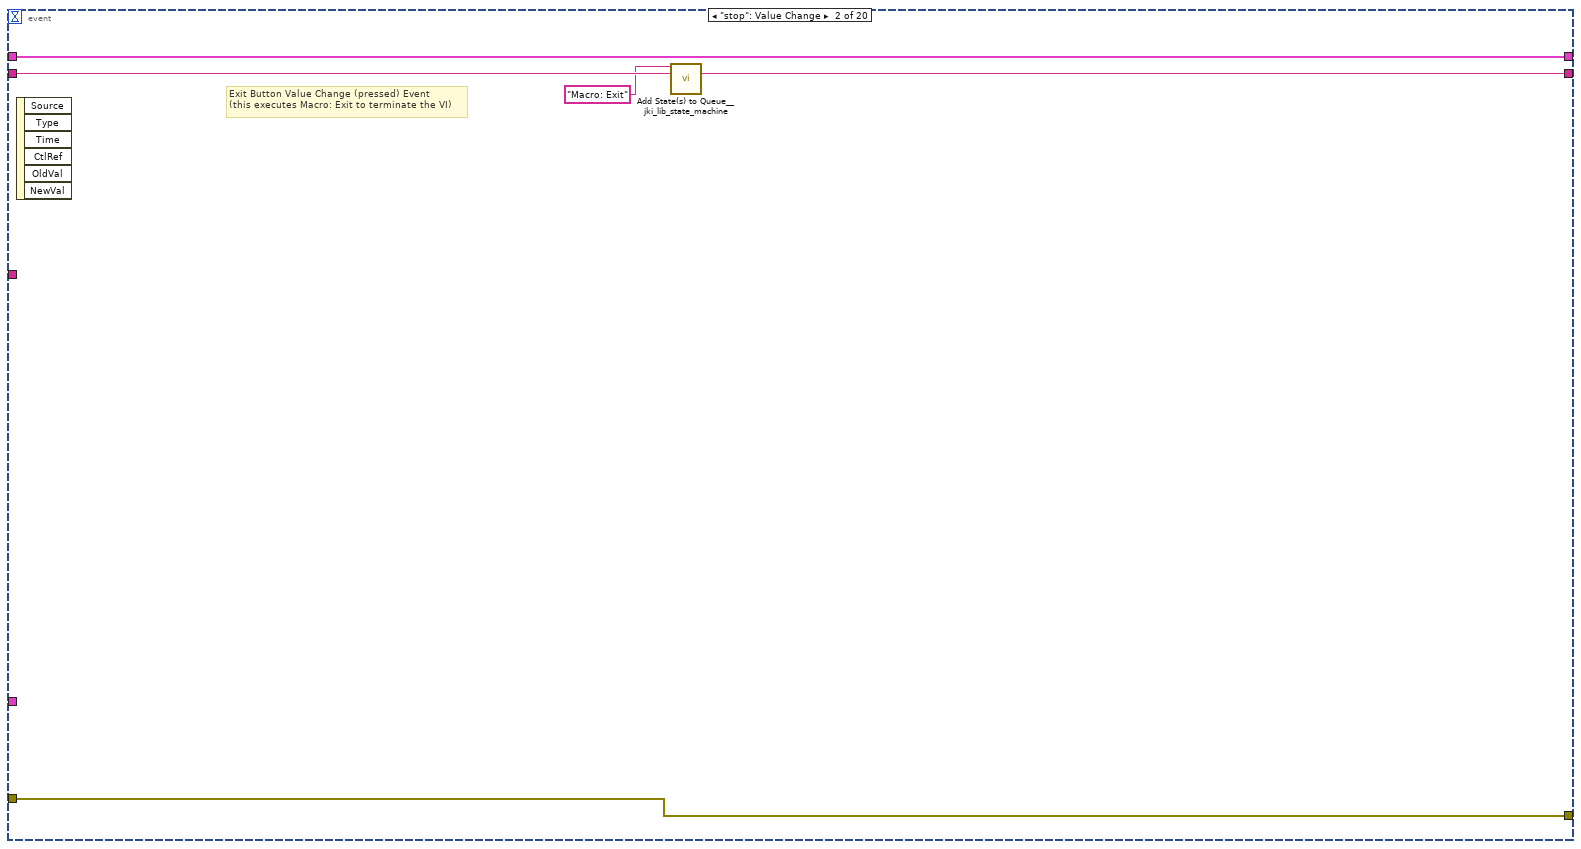
[diagram p7: hidden frame]
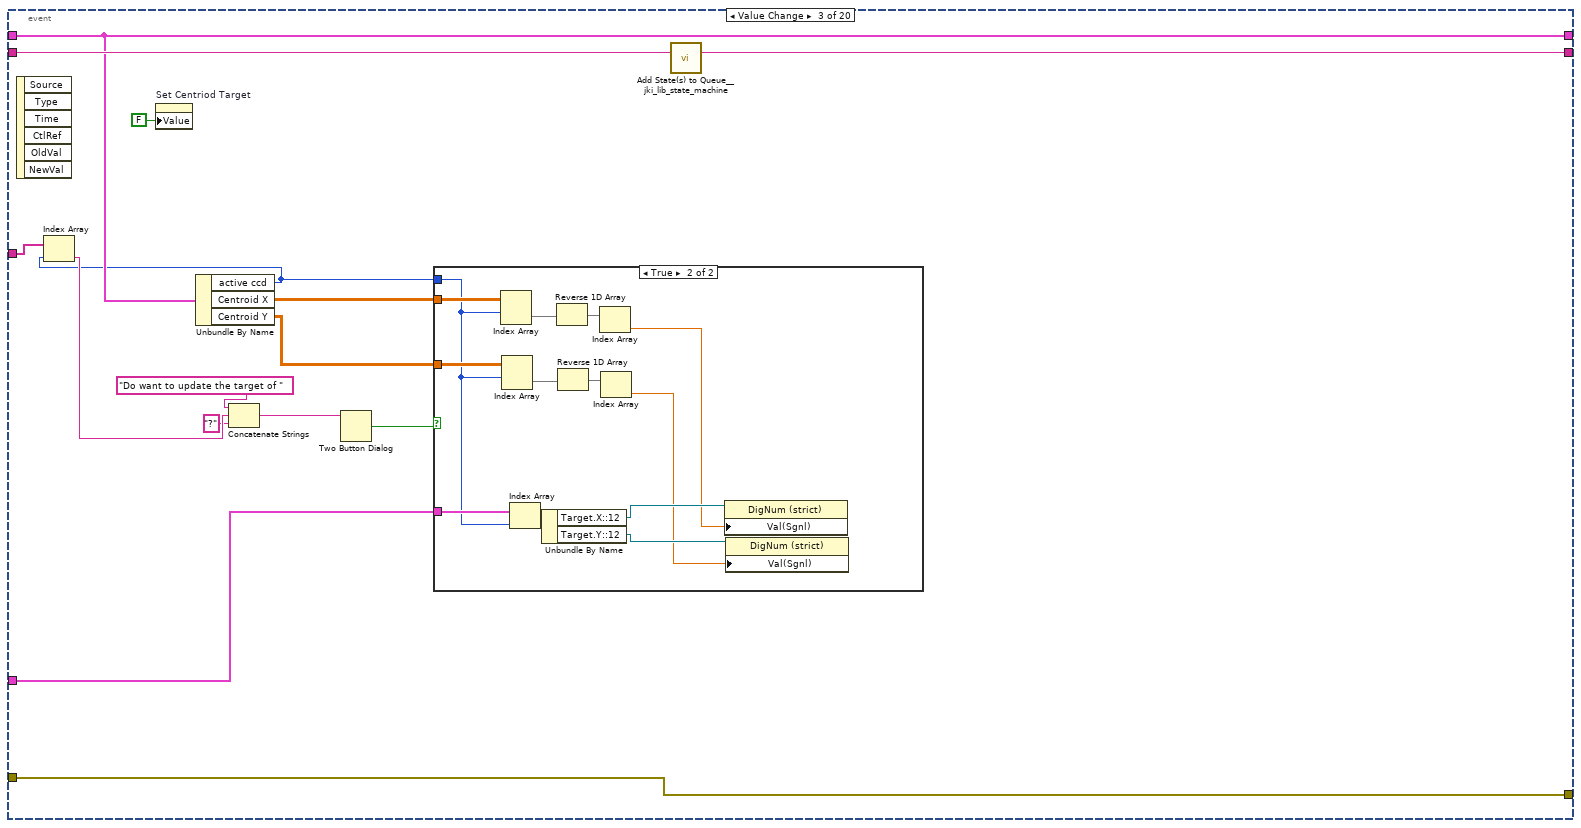
[diagram p8: hidden frame]
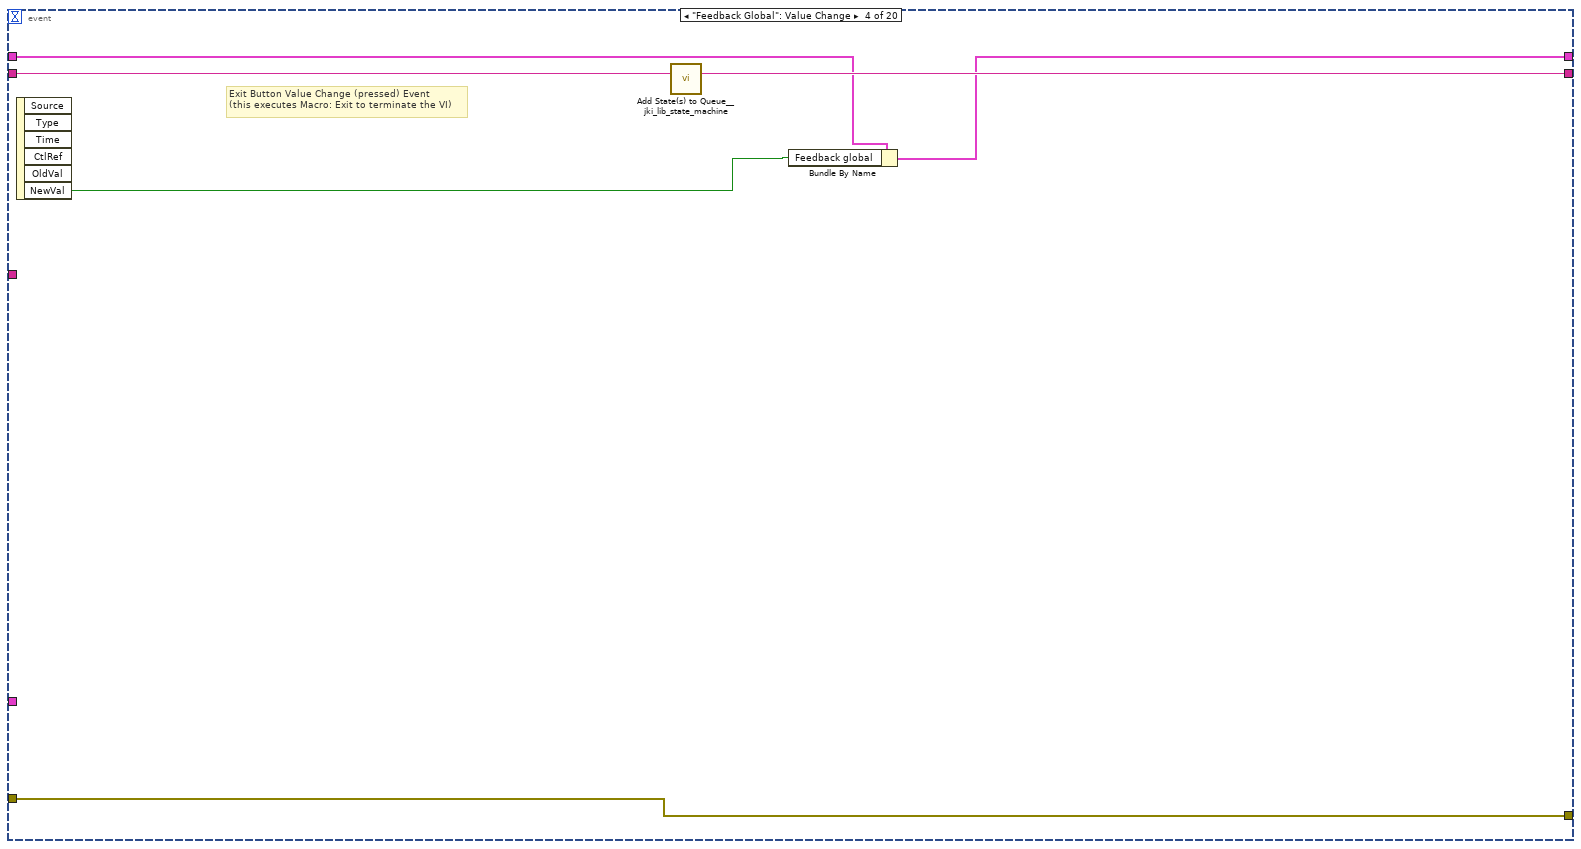
[diagram p10: hidden frame]
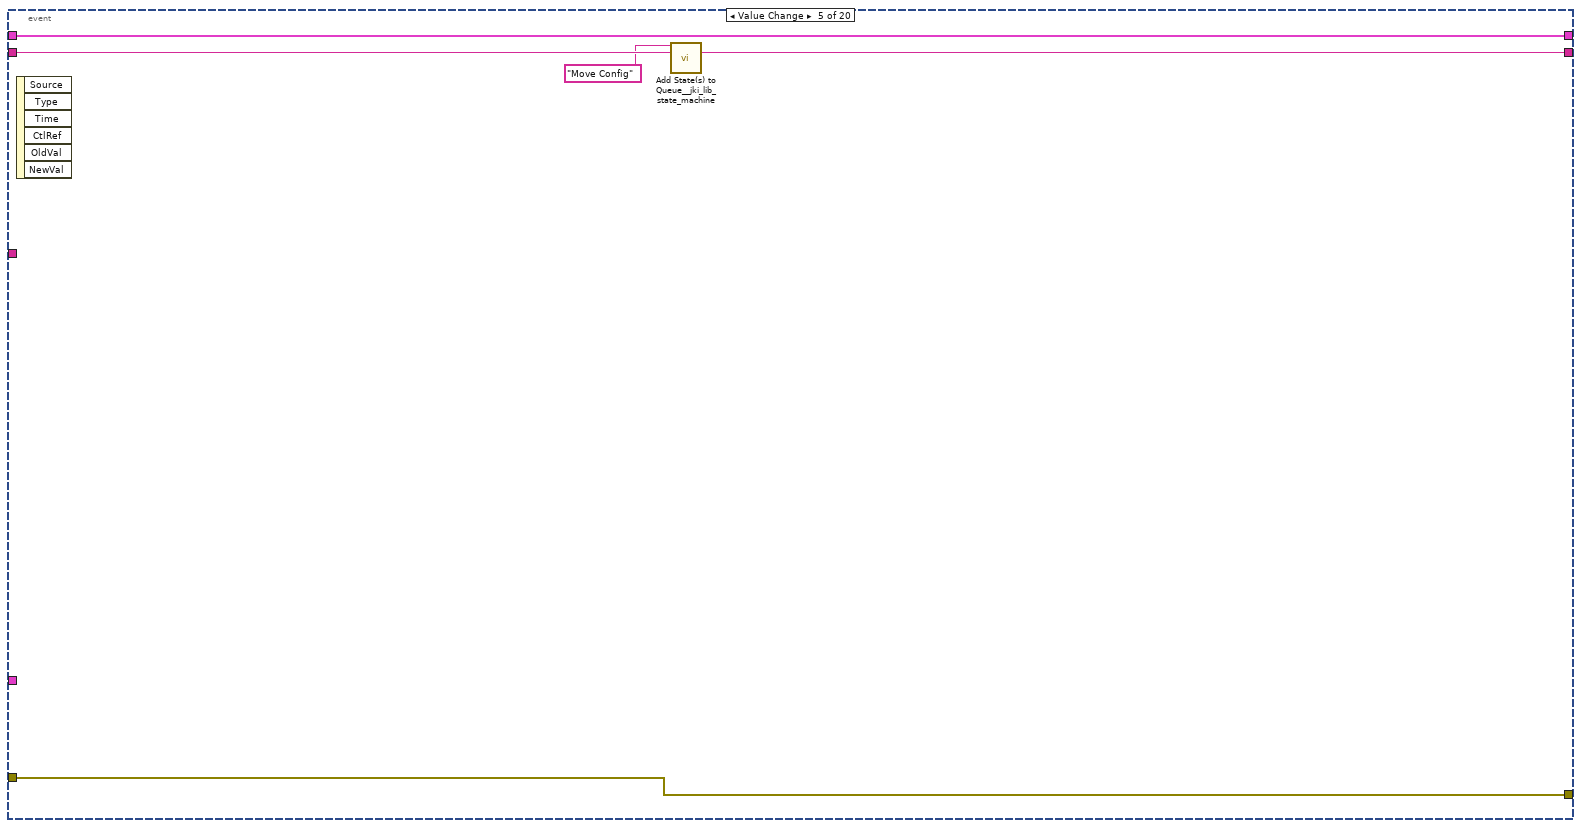
[diagram p11: hidden frame]
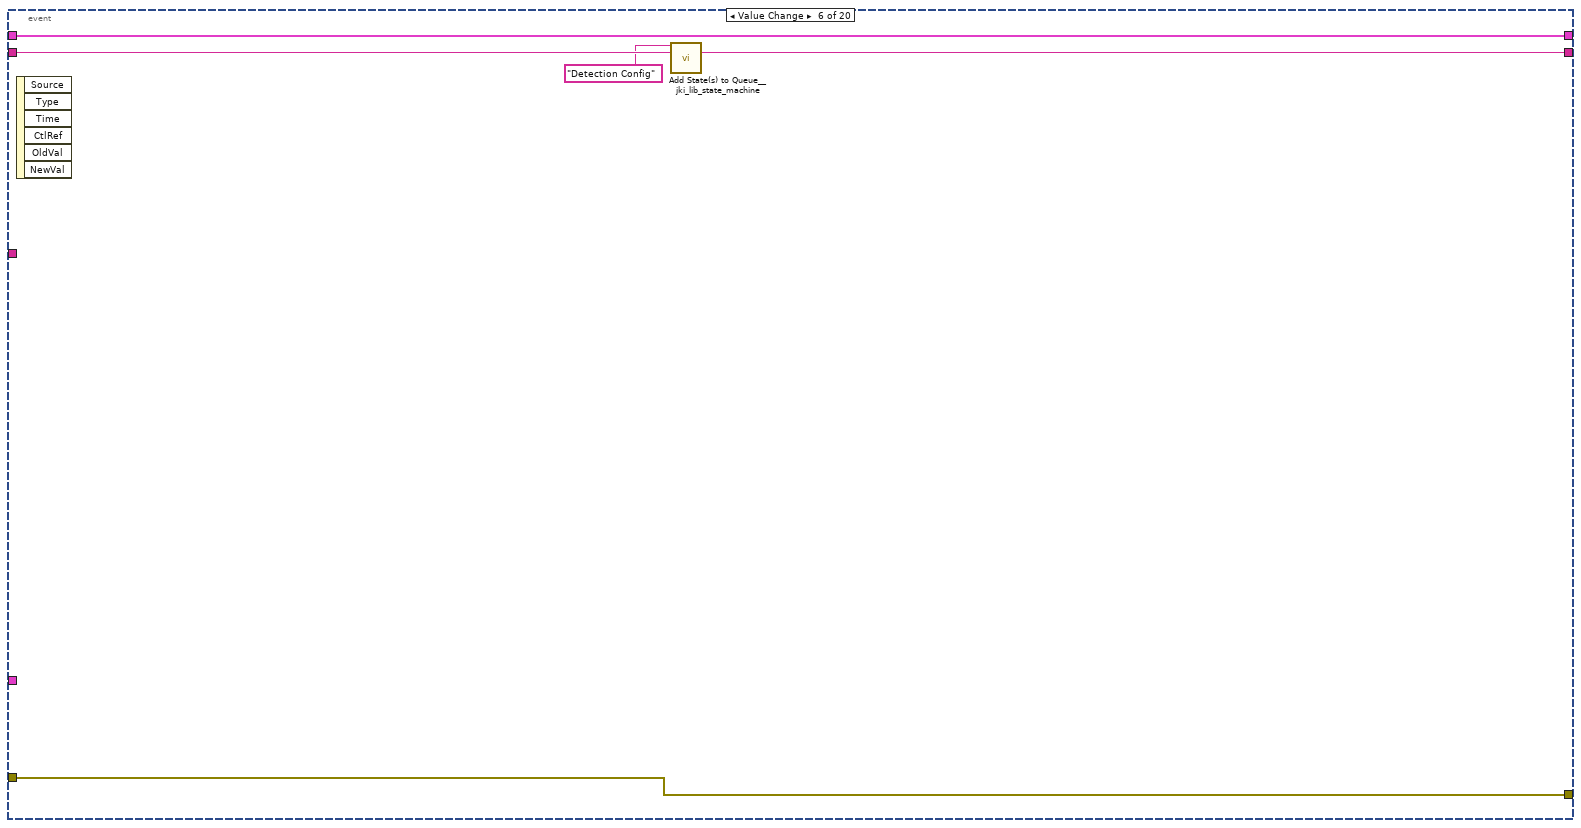
[diagram p12: hidden frame]
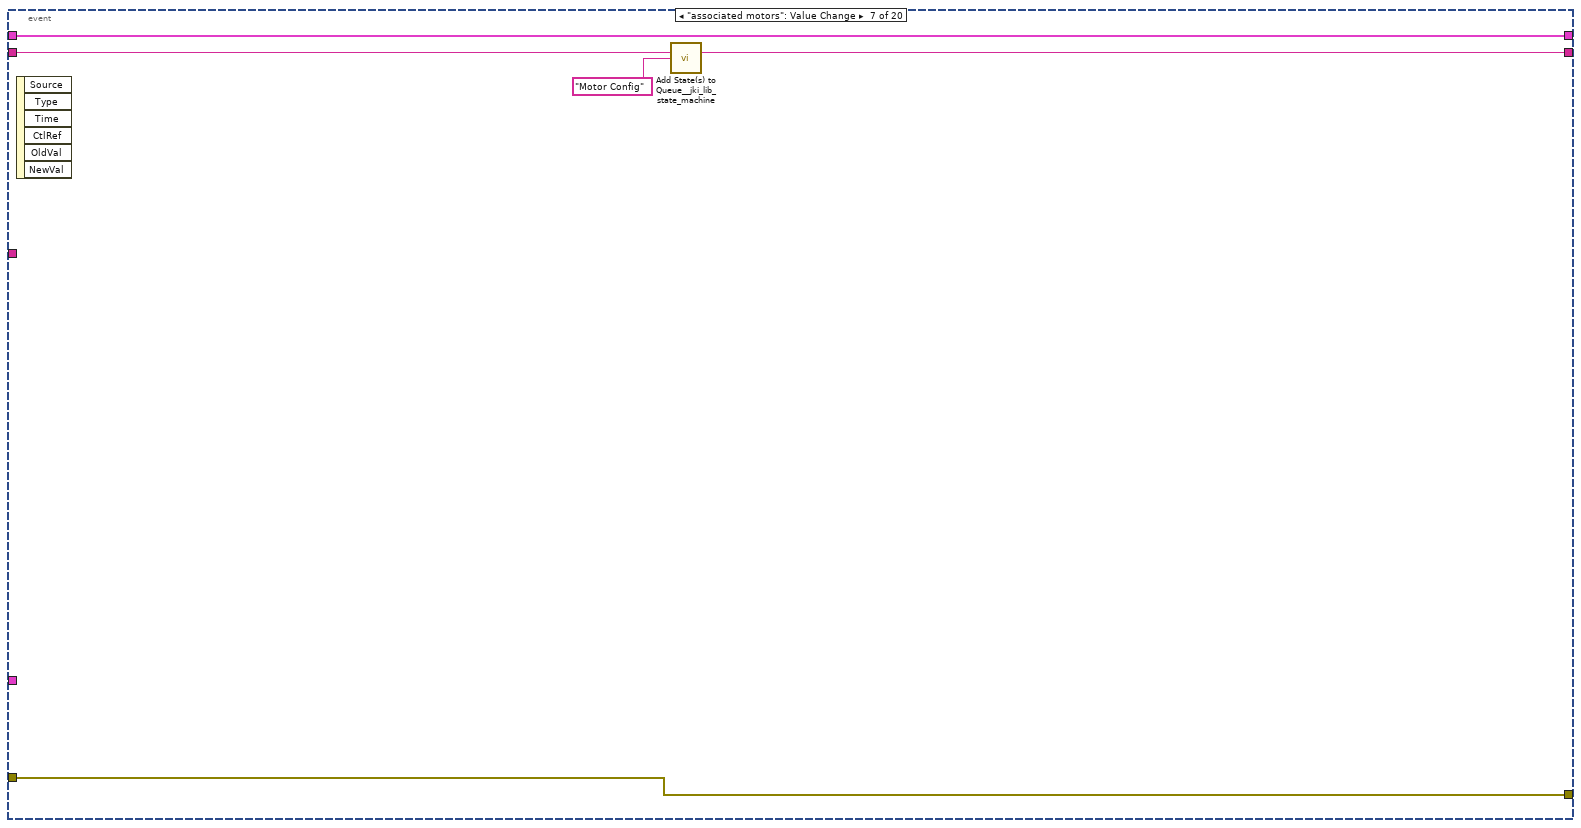
[diagram p13: hidden frame]
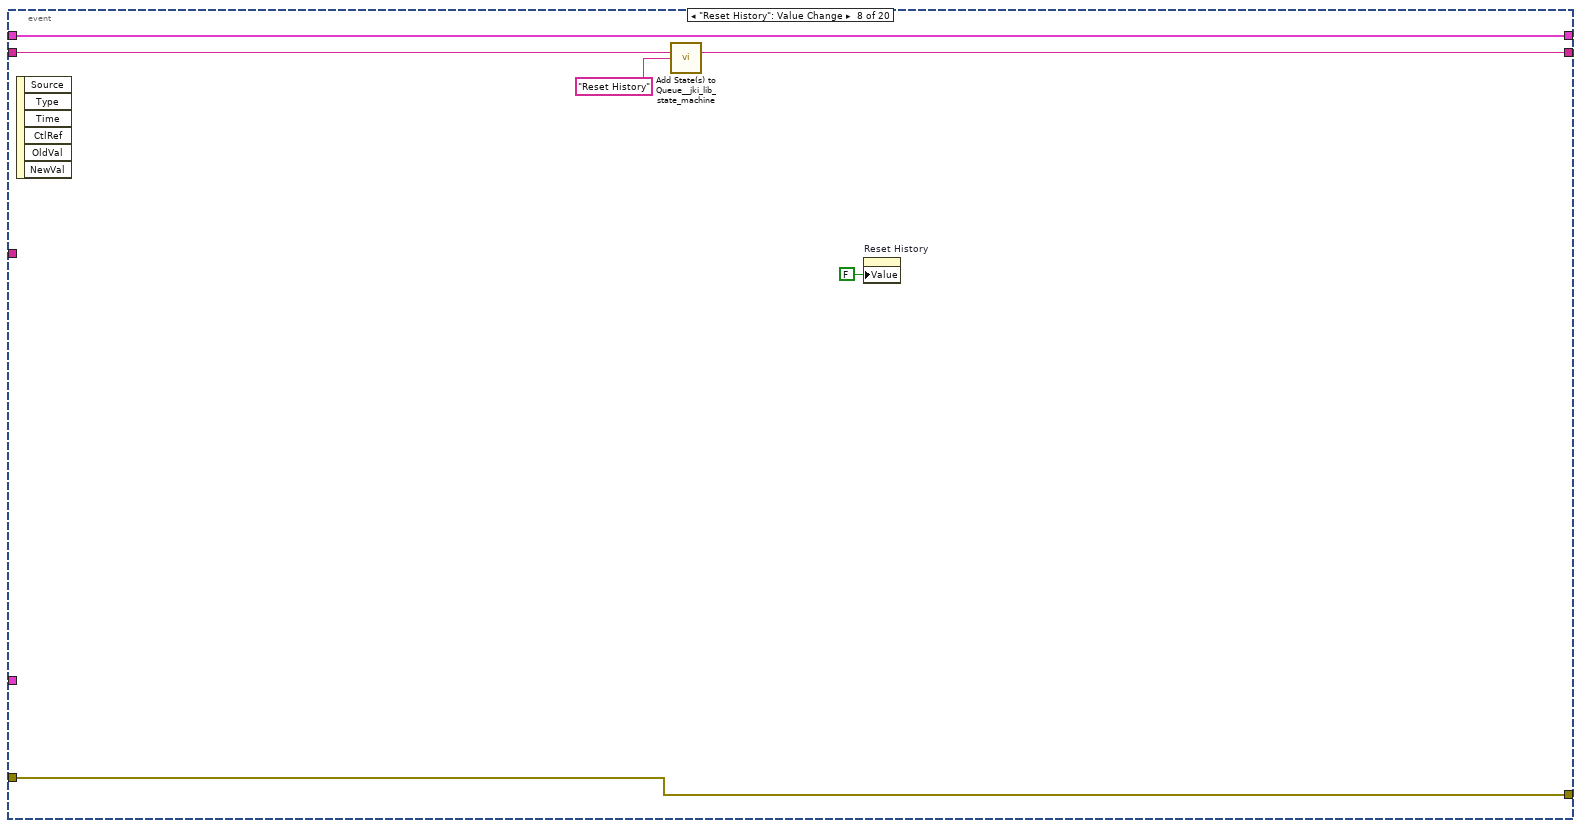
[diagram p14: hidden frame]
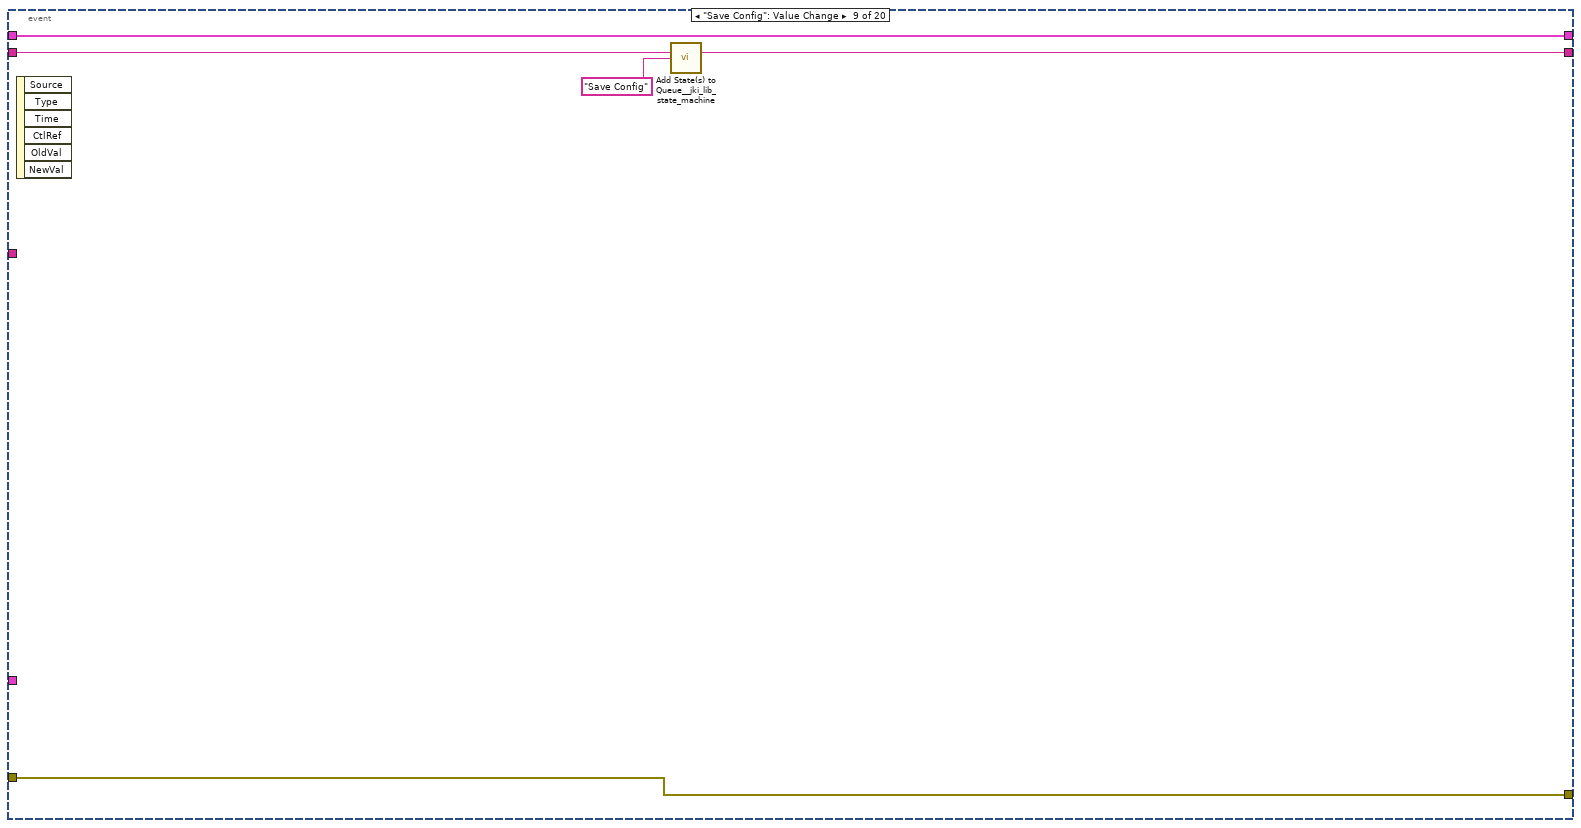
[diagram p15: hidden frame]
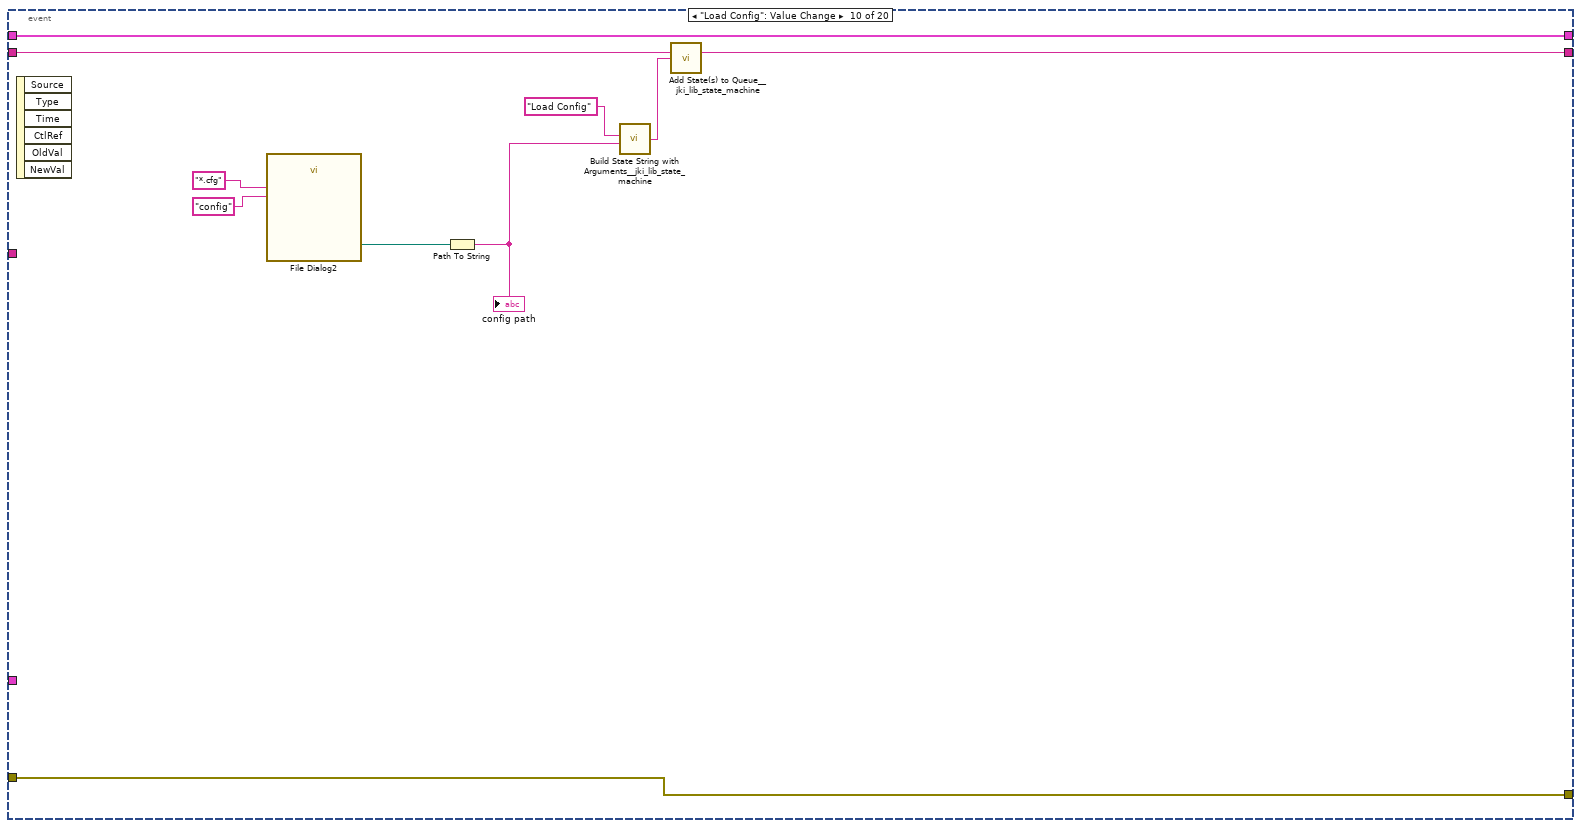
[diagram p16: hidden frame]
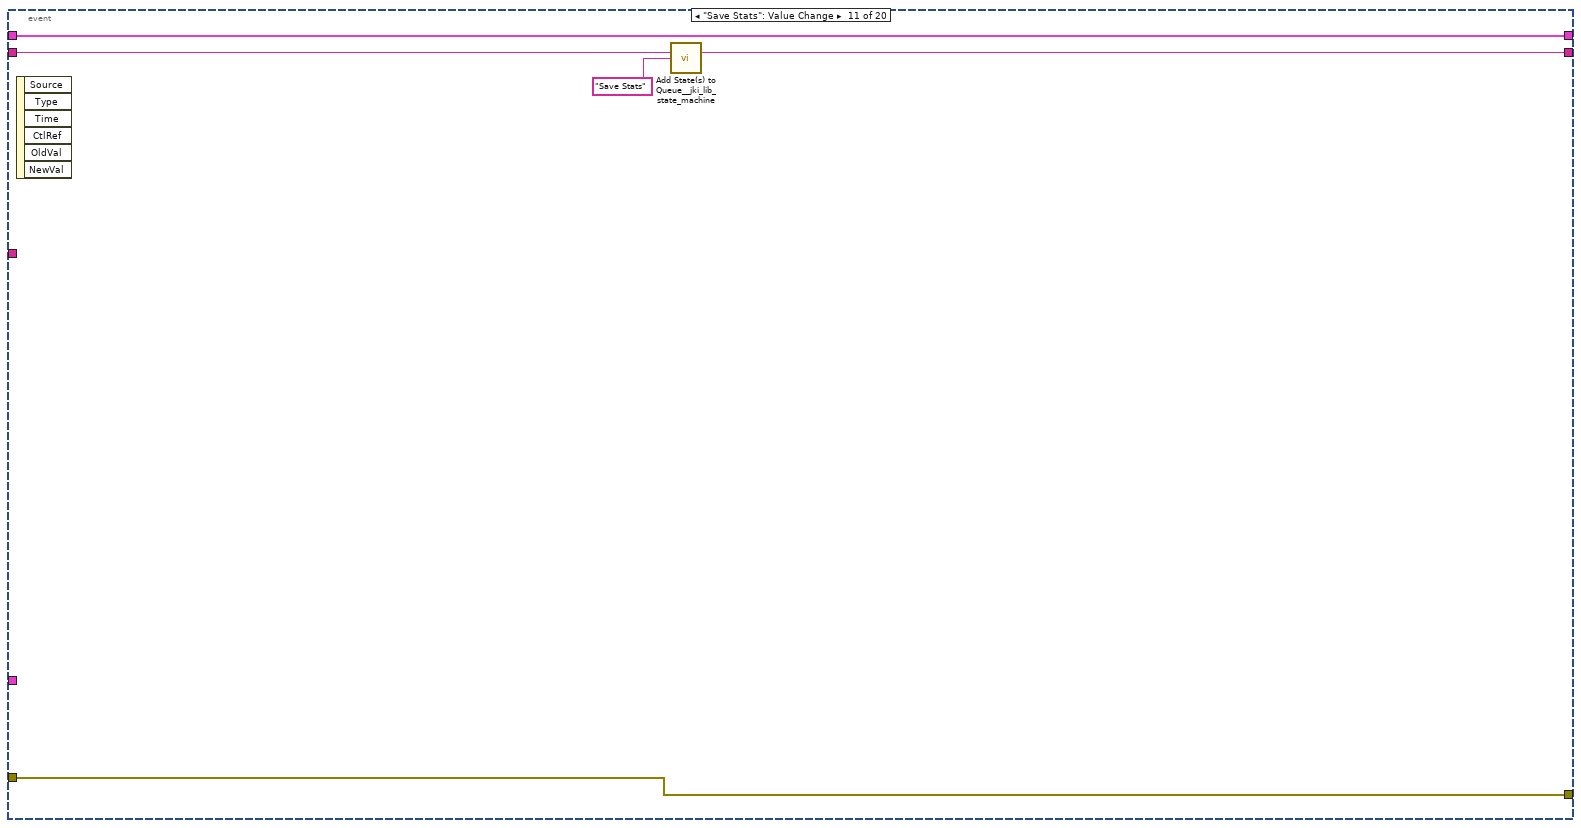
[diagram p17: hidden frame]
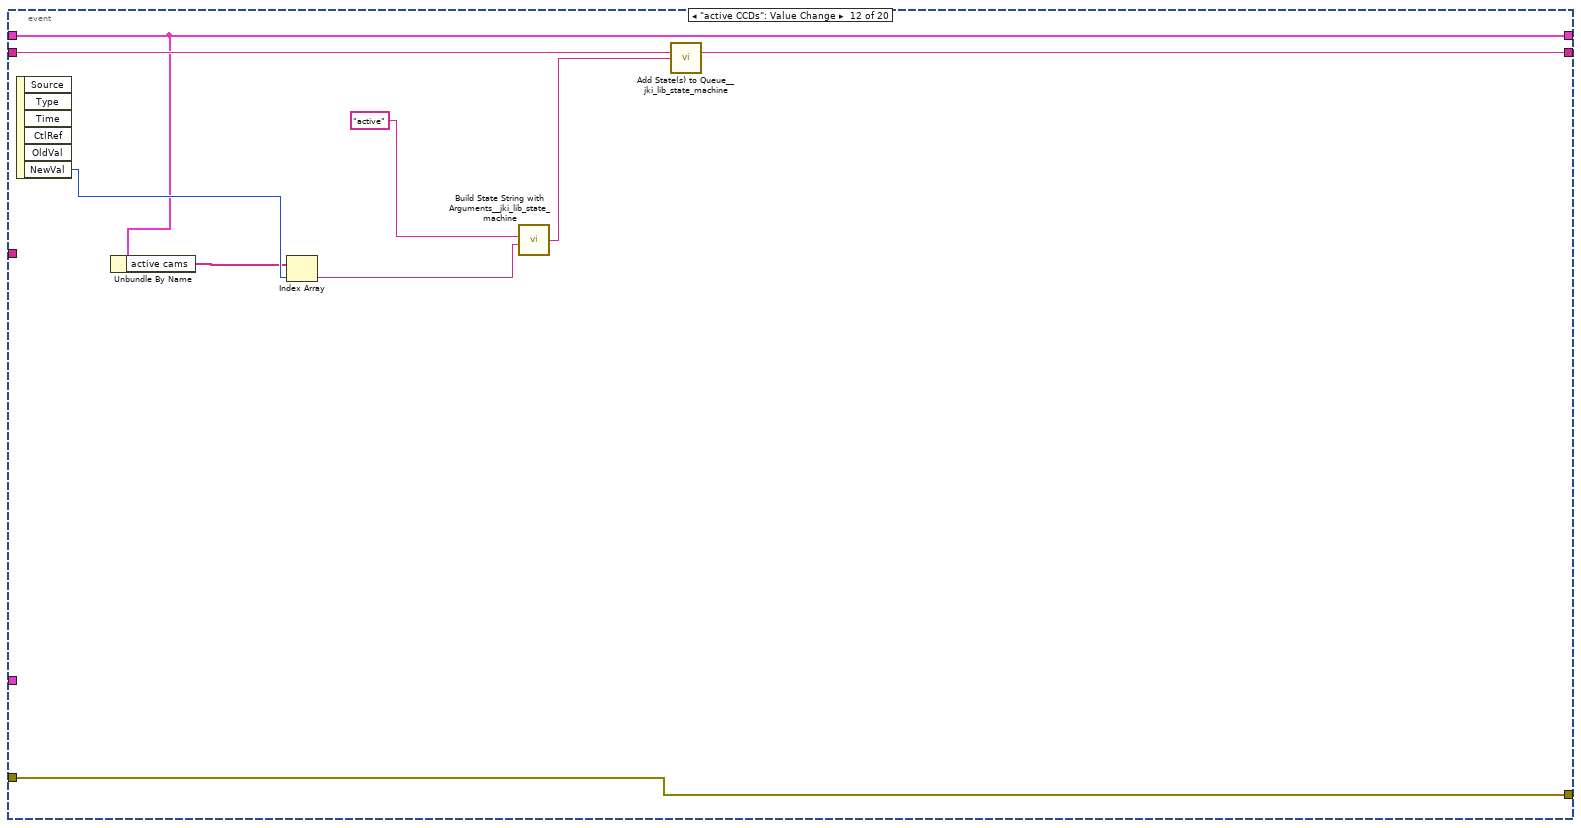
[diagram p18: hidden frame]
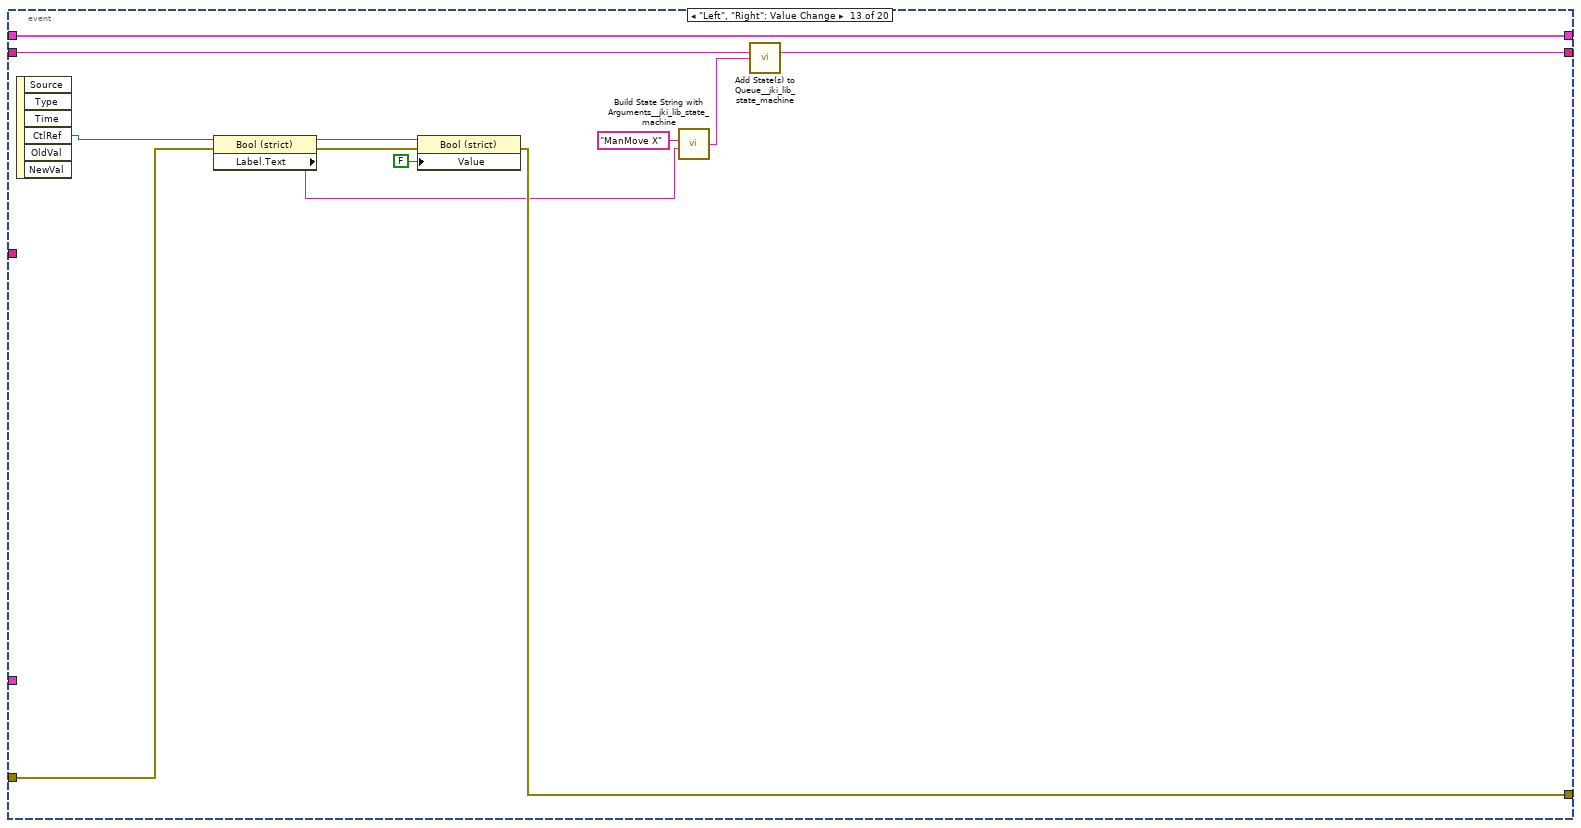
[diagram p19: hidden frame]
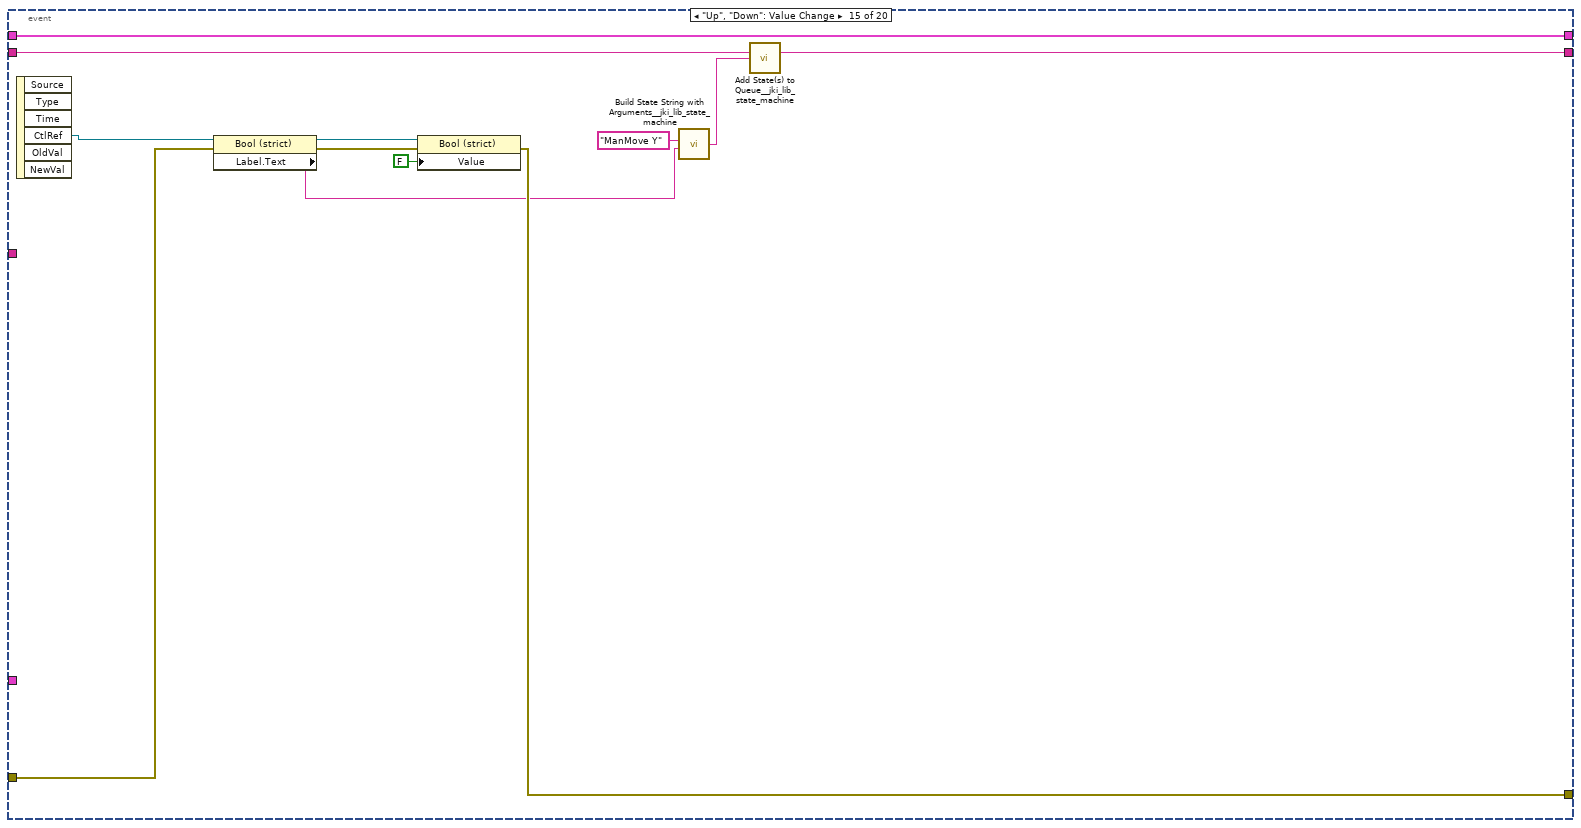
[diagram p20: hidden frame]
diagram:
  n1 = stacked-sequence {
    frame #0 {
      n2 = call <vilib>:"Application Directory.vi"() -> ("Application Directory"=w31:path)
      n3 = Build Path(base path=w31, name or relative path="defaultDevices_PICObooster.txt") -> (appended path=w29:path)
      "appended path" <- w29
      n4 = call-poly <vilib>:"Read From Spreadsheet File.vi"("file path (dialog if empty)"=w29) -> ("all rows"=w28:string[][])  [unwired: 6 in, 4 out]
      n5 = Index Array(array=w28, index (col) #1=0 ("disabled index (col)"), index (col) #2=1 ("index (col)")) -> (element #1=w25:string[])  [unwired: 2 in, 1 out]
      n6 = Index Array(array=w25, index #1=0 ("index"), index #2=1 ("index"), index #3=2 ("index"), index #4=3 ("index"), index #5=4 ("index"), index #6=5 ("index"), index #7=6 ("index"), index #8=7 ("index"), index #9=8 ("index"), index #10=9 ("index"), index #11=10 ("index"), index #12=11 ("index")) -> (element #1=w12:string, element #2=w11:string, element #3=w10:string, element #4=w9:string, element #5=w8:string, element #6=w7:string, element #7=w6:string, element #8=w5:string, element #9=w4:string, element #10=w3:string, element #11=w2:string, element #12=w1:string)
      n7 = property on="GUIdevice 1" class="Str"("Val(Sgnl)"=w12) -> ()  [unwired: 2 in, 2 out]
      n8 = property on="GUIdevice 2" class="Str"("Val(Sgnl)"=w11) -> ()  [unwired: 2 in, 2 out]
      n9 = property on="GUIdevice 3" class="Str"("Val(Sgnl)"=w10) -> ()  [unwired: 2 in, 2 out]
      n10 = property on="GUIdevice 4" class="Str"("Val(Sgnl)"=w9) -> ()  [unwired: 2 in, 2 out]
      n11 = property on="GUIdevice 5" class="Str"("Val(Sgnl)"=w8) -> ()  [unwired: 2 in, 2 out]
      n12 = property on="GUIdevice 6" class="Str"("Val(Sgnl)"=w7) -> ()  [unwired: 2 in, 2 out]
      n13 = property on="GUIdevice 7" class="Str"("Val(Sgnl)"=w6) -> ()  [unwired: 2 in, 2 out]
      n14 = property on="GUIdevice 8" class="Str"("Val(Sgnl)"=w5) -> ()  [unwired: 2 in, 2 out]
      n15 = property on="GUIdevice 9" class="Str"("Val(Sgnl)"=w4) -> ()  [unwired: 2 in, 2 out]
      n16 = property on="GUIdevice 10" class="Str"("Val(Sgnl)"=w3) -> ()  [unwired: 2 in, 2 out]
      n17 = property on="GUIdevice 11" class="Str"("Val(Sgnl)"=w2) -> ()  [unwired: 2 in, 2 out]
      n18 = property on="GUIdevice 12" class="Str"("Val(Sgnl)"=w1) -> ()  [unwired: 2 in, 2 out]
    }
    frame #1 {
      w32 = path "c:/BP_DATA" ("base path")
      w34 = string[] ["device12", "device45", "", ""] ("elements")
      w38 = T20 0 items=["Grayscale (U8)", "Grayscale (I16)", "Grayscale (SGL)", "Complex (CSG)", "RGB (U32)", "HSL (U32)", "RGB (U64)", "Grayscale (U16)"] ("Image Type")
      # "NOT FOR YOU MOFO"
      n19 = control-ref of="Position.device 1::99"() -> (w110:refnum<vi>)
      n20 = control-ref of="Position.device 2::99"() -> (w109:refnum<vi>)
      n21 = control-ref of="Position.device 4::99"() -> (w108:refnum<vi>)
      n22 = control-ref of="Position.device 5::99"() -> (w107:refnum<vi>)
      n23 = property on="Motor CCD 1" class="Ring (strict)"("Strings []"=w34) -> ()  [unwired: 2 in, 2 out]
      n24 = property on="Motor CCD 2" class="Ring (strict)"("Strings []"=w34) -> ()  [unwired: 2 in, 2 out]
      n25 = property on="Motor CCD 3" class="Ring (strict)"("Strings []"=w34) -> ()  [unwired: 2 in, 2 out]
      n26 = property on="Motor CCD 4" class="Ring (strict)"("Strings []"=w34) -> ()  [unwired: 2 in, 2 out]
      n27 = property on="Motor CCD 5" class="Ring (strict)"("Strings []"=w34) -> ()  [unwired: 2 in, 2 out]
      n28 = property on="Motor CCD 6" class="Ring (strict)"("Strings []"=w34) -> ()  [unwired: 2 in, 2 out]
      n29 = property on="Motor CCD 7" class="Ring (strict)"("Strings []"=w34) -> ()  [unwired: 2 in, 2 out]
      n30 = property on="Motor CCD 8" class="Ring (strict)"("Strings []"=w34) -> ()  [unwired: 2 in, 2 out]
      n31 = property on="Motor CCD 9" class="Ring (strict)"("Strings []"=w34) -> ()  [unwired: 2 in, 2 out]
      n32 = property on="Motor CCD 10" class="Ring (strict)"("Strings []"=w34) -> ()  [unwired: 2 in, 2 out]
      n33 = property on="Motor CCD 11" class="Ring (strict)"("Strings []"=w34) -> ()  [unwired: 2 in, 2 out]
      n34 = property on="Motor CCD 12" class="Ring (strict)"("Strings []"=w34) -> ()  [unwired: 2 in, 2 out]
      n35 = Build Array(w110, w109, w108, w107) -> (→"motor refs":refnum<vi>[])
      n36 = control-ref of="Target.X::1"() -> (w93:refnum<vi>)
      n37 = control-ref of="Target.Y::1"() -> (w92:refnum<vi>)
      n38 = control-ref of="Target.X::2"() -> (w91:refnum<vi>)
      n39 = control-ref of="Target.Y::2"() -> (w90:refnum<vi>)
      n40 = control-ref of="Target.X::3"() -> (w89:refnum<vi>)
      n41 = control-ref of="Target.Y::3"() -> (w88:refnum<vi>)
      n42 = control-ref of="Target.X::4"() -> (w87:refnum<vi>)
      n43 = control-ref of="Target.Y::4"() -> (w86:refnum<vi>)
      n44 = control-ref of="Target.X::5"() -> (w85:refnum<vi>)
      n45 = control-ref of="Target.Y::5"() -> (w84:refnum<vi>)
      n46 = control-ref of="Target.X::6"() -> (w83:refnum<vi>)
      n47 = control-ref of="Target.Y::6"() -> (w82:refnum<vi>)
      n48 = control-ref of="Target.X::7"() -> (w81:refnum<vi>)
      n49 = control-ref of="Target.Y::7"() -> (w80:refnum<vi>)
      n50 = control-ref of="Target.X::8"() -> (w79:refnum<vi>)
      n51 = control-ref of="Target.Y::8"() -> (w78:refnum<vi>)
      n52 = control-ref of="Target.X::9"() -> (w55:refnum<vi>)
      n53 = control-ref of="Target.Y::9"() -> (w54:refnum<vi>)
      n54 = control-ref of="Target.X::10"() -> (w53:refnum<vi>)
      n55 = control-ref of="Target.Y::10"() -> (w52:refnum<vi>)
      n56 = control-ref of="Target.X::11"() -> (w51:refnum<vi>)
      n57 = control-ref of="Target.Y::11"() -> (w50:refnum<vi>)
      n58 = control-ref of="Target.X::12"() -> (w49:refnum<vi>)
      n59 = control-ref of="Target.Y::12"() -> (w48:refnum<vi>)
      n60 = call "IMAQ Create"("Image Name"="GUIdevice 8", "Image Type"=w38) -> ("New Image"=→"image::8":T9)  [unwired: 3 in, 1 out]
      n61 = call "IMAQ Create"("Image Name"="GUIdevice 9", "Image Type"=w38) -> ("New Image"=→"image::9":T9)  [unwired: 3 in, 1 out]
      n62 = call "IMAQ Create"("Image Name"="GUIdevice 10", "Image Type"=w38) -> ("New Image"=→"image::10":T9)  [unwired: 3 in, 1 out]
      n63 = call "IMAQ Create"("Image Name"="GUIdevice 6", "Image Type"=w38) -> ("New Image"=→"image::6":T9)  [unwired: 3 in, 1 out]
      n64 = call "IMAQ Create"("Image Name"="GUIdevice 7", "Image Type"=w38) -> ("New Image"=→"image::7":T9)  [unwired: 3 in, 1 out]
      n65 = call "IMAQ Create"("Image Name"="GUIdevice 11", "Image Type"=w38) -> ("New Image"=→"image::11":T9)  [unwired: 3 in, 1 out]
      n66 = call "IMAQ Create"("Image Name"="GUIdevice 12", "Image Type"=w38) -> ("New Image"=→"image::12":T9)  [unwired: 3 in, 1 out]
      n67 = call "IMAQ Create"("Image Name"="GUIdevice 2") -> ("New Image"=→"image::2":T9)  [unwired: 4 in, 1 out]
      n68 = call "IMAQ Create"("Image Name"="GUIdevice 4", "Image Type"=w38) -> ("New Image"=→"image::4":T9)  [unwired: 3 in, 1 out]
      n69 = call "IMAQ Create"("Image Name"="GUIdevice 1", "Image Type"=w38) -> ("New Image"=→"image::1":T9)  [unwired: 3 in, 1 out]
      n70 = call "IMAQ Create"("Image Name"="GUIdevice 3", "Image Type"=w38) -> ("New Image"=→"image::3":T9)  [unwired: 3 in, 1 out]
      n71 = call "IMAQ Create"("Image Name"="GUIdevice 5", "Image Type"=w38) -> ("New Image"=→"image::5":T9)  [unwired: 3 in, 1 out]
      n72 = Build Array("GUIdevice 1", "GUIdevice 2", "GUIdevice 3", "GUIdevice 4", "GUIdevice 5", "GUIdevice 6", "GUIdevice 7", "GUIdevice 8", "GUIdevice 9", "GUIdevice 10", "GUIdevice 11", "GUIdevice 12") -> (w67:string[])
      "CCDs" <- w67
      n73 = property on="image::8" class="ImageControl"("Caption.Text"="GUIdevice 8") -> ()  [unwired: 2 in, 2 out]
      n74 = property on="image::10" class="ImageControl"("Caption.Text"="GUIdevice 10") -> ()  [unwired: 2 in, 2 out]
      n75 = property on="image::9" class="ImageControl"("Caption.Text"="GUIdevice 9") -> ()  [unwired: 2 in, 2 out]
      n76 = property on="image::1" class="ImageControl"("Caption.Text"="GUIdevice 1") -> ()  [unwired: 2 in, 2 out]
      n77 = property on="image::2" class="ImageControl"("Caption.Text"="GUIdevice 2") -> ()  [unwired: 2 in, 2 out]
      n78 = property on="image::3" class="ImageControl"("Caption.Text"="GUIdevice 3") -> ()  [unwired: 2 in, 2 out]
      n79 = property on="image::4" class="ImageControl"("Caption.Text"="GUIdevice 4") -> ()  [unwired: 2 in, 2 out]
      n80 = property on="image::5" class="ImageControl"("Caption.Text"="GUIdevice 5") -> ()  [unwired: 2 in, 2 out]
      n81 = property on="image::6" class="ImageControl"("Caption.Text"="GUIdevice 6") -> ()  [unwired: 2 in, 2 out]
      n82 = property on="image::7" class="ImageControl"("Caption.Text"="GUIdevice 7") -> ()  [unwired: 2 in, 2 out]
      n83 = property on="image::11" class="ImageControl"("Caption.Text"="GUIdevice 11") -> ()  [unwired: 2 in, 2 out]
      n84 = property on="image::12" class="ImageControl"("Caption.Text"="GUIdevice 12") -> ()  [unwired: 2 in, 2 out]
      n85 = Array To Cluster(array=w67) -> (cluster=→"Cameras":T21)
      n86 = Bundle("Target.X::1"=w93, "Target.Y::1"=w92) -> (w77:T22)  [unwired: 1 in]
      n87 = Bundle("Target.X::2"=w91, "Target.Y::2"=w90) -> (w76:T23)  [unwired: 1 in]
      n88 = Bundle("Target.X::3"=w89, "Target.Y::3"=w88) -> (w75:T24)  [unwired: 1 in]
      n89 = Bundle("Target.X::4"=w87, "Target.Y::4"=w86) -> (w68:T25)  [unwired: 1 in]
      n90 = Bundle("Target.X::5"=w85, "Target.Y::5"=w84) -> (w74:T26)  [unwired: 1 in]
      n91 = Bundle("Target.X::6"=w83, "Target.Y::6"=w82) -> (w73:T27)  [unwired: 1 in]
      n92 = Bundle("Target.X::7"=w81, "Target.Y::7"=w80) -> (w72:T28)  [unwired: 1 in]
      n93 = Bundle("Target.X::8"=w79, "Target.Y::8"=w78) -> (w71:T29)  [unwired: 1 in]
      n94 = Bundle("Target.X::12"=w49, "Target.Y::12"=w48) -> (w44:T30)  [unwired: 1 in]
      n95 = Bundle("Target.X::9"=w55, "Target.Y::9"=w54) -> (w47:T31)  [unwired: 1 in]
      n96 = Bundle("Target.X::10"=w53, "Target.Y::10"=w52) -> (w46:T32)  [unwired: 1 in]
      n97 = Bundle("Target.X::11"=w51, "Target.Y::11"=w50) -> (w45:T33)  [unwired: 1 in]
      n98 = property on="CCDs" class="Ring (strict)"("Strings []"=w67) -> ()  [unwired: 2 in, 2 out]
      n99 = Build Array(w77, w76, w75, w68, w74, w73, w72, w71, w47, w46, w45, w44) -> (w70:T34)
      n100 = Tick Count (ms)() -> (millisecond timer value=→"millisecond timer value":u32)
      n101 = property on="Feedback Global" class="Bool (strict)"("Value"=FALSE ("Feedback Global")) -> ()  [unwired: 2 in, 2 out]
      n102 = Get Date/Time In Seconds() -> (seconds since 1Jan1904=w57:timestamp)
      n103 = Format Date/Time String(time format string (%c)="%Y%m%d%H%M", seconds (now)=w57) -> (date/time string=w56:string)  [unwired: 1 in]
      n104 = Concatenate Strings(w56, "Beampointing_PICObooster.tdms" ("string")) -> (w60:string)
      n105 = String To Path(string=w60) -> (path=w59:path)
      n106 = Build Path(base path=w32, name or relative path=w59) -> (appended path=w62:path)
      n107 = call <vilib>:"Add State(s) to Queue__jki_lib_state_machine.vi"("State(s) in (\"\")"="Macro: Initialize") -> ("States Out"=w112:string)  [unwired: 14 in]
      n108 = Create User Event(user event datatype=T13 {"EventEnum"=enum."new data", "Device name"="Device name"} ("New Event")) -> (user event=w120:refnum<user-event>, error out=w122:errorcluster)  [unwired: 1 in]
      "tcp data event" <- w120
      n109 = while "JKI - String-Based Queued State Machine (Basic) v1.0" {
        shift-right: [w140] -> w66
        shift-left: _ -> [w133]
        shift-right: [w143] -> w94
        shift-left: _ -> [w139]
        shift-right: [w142] -> _
        shift-left: w112 -> [w144]
        tunnel: w70 -> [w137]
        tunnel: w67 -> [w135]
        tunnel: [w135] -> w95
        tunnel: w70 -> [w136]
        tunnel: w62 -> [w131]
        tunnel: w32 -> [w130]
        stop <- w141 stop-if-true
        n110 = Unbundle By Name(w133) -> ("active cams"=w132:string[])
        n111 = call <vilib>:"Parse State Queue__jki_lib_state_machine.vi"("State Queue"=w144, "Error In (no error)"=w139) -> ("Remaining States"=w146:string, "Current State"=w147:string, "Arguments"=w145:string)  [unwired: 11 in]
        "Current State" <- w147
        n112 = case shown="\"\", \"Idle\"" w147 {
          selector: w147 -> [_ _ w449 _ _ _ _ _ _ _ _ _ _ _ _ _ _ _ _ _ _ _ _ _ _ _ _ _ _ _ _ _ _ _ _ _ _ _ _ _ _ _]
          tunnel: w146 -> [w172 w448 w453 w471 w477 w482 w486 w525 w541 w545 w549 w555 w566 w590 w599 w609 w613 w637 w756 w808 w838 w847 w869 w890 w894 w910 w1053 w1192 w1272 w1336 w1407 w1483 w1507 w1522 w1596 w1648 w1658 w1698 w1787 w1813 w1824 w1847]
          tunnel: w145 -> [_ _ _ _ _ _ _ _ _ _ _ w550 w561 _ _ _ _ w632 w709 _ w823 _ _ _ _ w911 _ w1167 w1258 w1322 w1382 w1477 _ _ _ _ _ _ _ _ w1828 _]
          tunnel: w133 -> [w170 w445 w451 w461 w474 w480 w483 _ w536 w542 w547 w553 w560 w587 w596 w601 w610 w630 w746 w806 w819 w843 w861 w883 w891 w899 w1034 w1185 w1268 w1332 w1400 w1479 w1504 w1519 w1592 w1645 w1655 w1672 w1785 w1810 w1827 w1838]
          tunnel: [w169 w446 w455 w469 errorcluster {"status"=FALSE, "code"=0, "source"=""} ("error out") w479 w484 w492 w538 w543 w546 w551 w563 w588 w597 w607 w611 w633 w712 w797 w827 w845 w867 w888 w892 w942 w1066 w1190 w1270 w1334 w1405 w1472 w1505 w1520 w1593 w1646 w1656 w1660 w1749 w1811 w1822 w1845] -> w143
          tunnel: w139 -> [w168 w446 w454 w469 w473 w479 w484 w493 w539 w543 w546 w552 w564 w588 w597 w607 w611 w634 w710 w798 w826 w845 w867 w888 w892 w942 w1066 w1190 w1270 w1334 w1405 w1473 w1505 w1520 w1594 w1646 w1656 w1661 w1783 w1811 w1822 w1845]
          tunnel: [w171 w447 w452 w470 w476 w481 w485 w524 w540 w544 w548 w554 w565 w589 w598 w608 w612 w624 w755 w807 w837 w846 w868 w889 w893 w913 w1067 w1191 w1271 w1335 w1406 w1482 w1506 w1521 w1595 w1647 w1657 w1697 w1786 w1812 w1823 w1846] -> w142
          tunnel: [_ _ _ _ _ TRUE _ _ _ _ _ _ _ _ _ _ _ _ _ _ _ _ _ _ _ _ _ _ _ _ _ _ _ _ _ _ _ _ _ _ _ _] -> w141
          tunnel: [w165 w445 w451 w460 w474 w480 w483 w494 w536 w542 w547 w553 w560 w587 w596 w601 w610 w636 w745 w806 w832 w842 w860 w882 w891 w935 w1033 w1185 w1268 w1332 w1400 w1481 w1504 w1519 w1592 w1644 w1655 w1672 w1784 w1810 w1826 w1837] -> w140
          tunnel: "update speed [ms]" -> [w167 _ _ _ _ _ _ _ _ _ _ _ _ _ _ _ _ _ _ _ _ _ _ _ _ _ _ _ _ _ _ _ _ _ _ _ _ _ _ _ _ _]
          tunnel: w137 -> [w164 _ _ _ _ _ _ _ _ _ _ _ _ _ _ _ _ _ _ _ _ _ _ _ _ w933 _ _ _ _ _ _ _ _ _ _ _ _ _ w1795 _ _]
          tunnel: w135 -> [w166 _ _ _ _ _ _ w489 _ _ _ _ _ _ _ _ _ w616 w744 _ w833 _ _ _ _ w903 w1032 w1189 _ _ w1404 w1478 _ w1509 _ _ _ w1671 _ _ _ _]
          tunnel: w131 -> [_ _ _ _ _ _ _ w491 _ _ _ _ _ _ _ _ _ w635 _ _ _ _ _ _ _ _ _ _ _ _ _ _ _ _ _ _ _ _ _ _ _ _]
          tunnel: w130 -> [_ _ _ _ _ _ _ _ _ _ _ _ _ _ _ _ _ _ _ _ _ _ _ _ _ _ _ _ _ _ _ _ _ _ _ _ _ _ w1755 _ _ _]
          frame "", "Idle" {
            # "executes when the state queue is empty"
            n113 = event shown="[13] \"Tab Control 2\": Value Change" {
              selector: _ -> [_ _ _ _ _ _ _ _ _ _ _ _ _ _ _ _ _ _ _ _]
              dyn-events: _ -> [_ _ _ _ _ _ _ _ _ _ _ _ _ _ _ _ _ _ _ _]
              timeout: w167 -> [_ _ _ _ _ _ _ _ _ _ _ _ _ _ _ _ _ _ _ _]
              tunnel: w172 -> [w174 w301 w316 w335 w340 w345 w350 w356 w361 w371 w376 w385 w397 w399 w414 w419 w424 w430 w434 w444]
              tunnel: [w201 w300 w315 w334 w339 w344 w349 w355 w360 w370 w375 w384 w396 w398 w413 w418 w423 w429 w432 w443] -> w171
              tunnel: w170 -> [w197 w298 w312 w331 w337 w342 w347 w353 w358 w368 w373 w378 w395 w402 w412 w417 w422 w428 w435 w441]
              tunnel: [w213 w299 w314 w333 w338 w343 w348 w354 w359 w369 w374 w383 w390 w400 w407 w416 w421 w427 w431 w442] -> w169
              tunnel: w168 -> [w188 w299 w314 w333 w338 w343 w348 w354 w359 w369 w374 w383 w391 w400 w408 w416 w421 w427 w431 w442]
              tunnel: [w200 w298 w312 w330 w337 w342 w347 w353 w358 w368 w373 w378 w395 w402 w412 w417 w422 w428 w435 w441] -> w165
              tunnel: w166 -> [w193 _ w308 _ _ _ _ _ _ _ _ _ _ _ _ _ _ _ _ _]
              tunnel: w164 -> [_ _ w310 _ _ _ _ _ _ _ _ _ _ _ _ _ _ _ _ _]
              event Timeout {
                n114 = event-data() -> ()  [unwired: 1 in, 1 out]
                n115 = Unbundle By Name(w197) -> ("Centroid X"=w194:dbl[][], "Centroid Y"=w191:dbl[][], "Size"=w189:dbl[][], "detection para"=w184:T3[], "active cams"=w192:string[], "thresholds"=w190:cluster{"Lower value":sgl, "Upper value":sgl}[])
                n116 = Unbundle By Name(w197) -> ("active ccd"=w196:i32)
                n117 = for {
                  tunnel: w192 -> [w234] mode=indexing
                  tunnel: [w235] -> w179 mode=indexing
                  tunnel: w193 -> [w257]
                  tunnel: w184 -> [w255]
                  tunnel: [w218] -> w178 mode=indexing
                  tunnel: [w253] -> w187 mode=indexing
                  tunnel: [w251] -> w195 mode=indexing
                  tunnel: "autodetect" -> [w245]
                  tunnel: w188 -> [w258]
                  tunnel: [w259] -> w186
                  shift-right: [w242] -> w183
                  shift-left: w190 -> [w244]
                  shift-right: [w229] -> w182
                  shift-left: w194 -> [w231]
                  shift-right: [w225] -> w181
                  shift-left: w191 -> [w227]
                  shift-right: [w219] -> w180
                  shift-left: w189 -> [w221]
                  w223 = 0 ("index")
                  n118 = call-poly <userlib>:"Filter 1D Array__ogtk.vi"("items to filter"=w234, "array"=w257) -> ("filtered item indices"=w256:i32[])  [unwired: 4 in, 1 out]
                  n119 = Index Array(array=w256) -> (element=w220:i32)  [unwired: 1 in]
                  n120 = Index Array(array=w221, index (row)=w220) -> (element=w249:dbl[])  [unwired: 1 in]
                  n121 = Index Array(array=w227, index (row)=w220) -> (element=w250:dbl[])  [unwired: 1 in]
                  n122 = Index Array(array=w244, index=w220) -> (element=w248:cluster{"Lower value":sgl, "Upper value":sgl})
                  n123 = Index Array(array=w231, index (row)=w220) -> (element=w233:dbl[])  [unwired: 1 in]
                  n124 = Index Array(array=w255, index=w220) -> (element=w252:T3)
                  n125 = call "CENTRIOD DETECTION.vi"("Refnum in"=w234, "auto threshold"=w245, "Threshold Range In"=w248, "beam detection para"=w252, "error in (no error)"=w258) -> ("Bounding Rect"=w251:T35, "Particle Reports (Pixels)"=w253:T1, "Threshold Range Out"=w243:cluster{"Lower value":sgl, "Upper value":sgl}, "Centriod"=w260:cluster{"X":dbl, "Y":dbl}, "error out"=w259:errorcluster)  [unwired: 7 in, 3 out]
                  n126 = Unbundle By Name(w260) -> ("X"=w232:dbl, "Y"=w228:dbl)
                  n127 = Empty Array?(array=w253) -> (empty?=w254:bool)
                  n128 = Not(x=w254) -> (.not. x?=w218:bool)
                  n129 = Replace Array Subset(array=w244, new element=w243, index=w220) -> (w242:cluster{"Lower value":sgl, "Upper value":sgl}[])
                  n130 = Unbundle By Name(w251) -> ("Right"=w241:dbl, "Left"=w240:dbl, "Bottom"=w239:dbl, "Top"=w238:dbl)
                  n131 = Subtract(x=w241, y=w240) -> (x-y=w236:dbl)
                  n132 = Subtract(x=w239, y=w238) -> (x-y=w237:dbl)
                  n133 = Multiply(x=w236, y=w237) -> (x*y=w224:dbl)
                  n134 = Insert Into Array(array=w250, index=w223, new element=w228) -> (w226:dbl[])
                  n135 = Insert Into Array(array=w233, index=w223, new element=w232) -> (w230:dbl[])
                  n136 = Insert Into Array(array=w249, index=w223, new element=w224) -> (w222:dbl[])
                  n137 = for {
                    shift-right: [w261] -> w246
                    shift-left: dbl[] [] ("Array 4") -> [w264]
                    tunnel: w226 -> [w262] mode=indexing
                    n138 = Equal To 0?(x=w262) -> (x = 0?=w263:bool)
                    n139 = case shown="False" w263 {
                      tunnel: w264 -> [w267 w268]
                      tunnel: w262 -> [w266 _]
                      tunnel: [w265 w268] -> w261
                      frame False {
                        n140 = Build Array (concatenate)(w267, w266) -> (w265:dbl[])
                      }
                      frame True {
                      }
                    }
                  }
                  n141 = Replace Array Subset(array=w231, new element=w230, index (row)=w220) -> (w229:dbl[][])  [unwired: 1 in]
                  n142 = Replace Array Subset(array=w227, new element=w226, index (row)=w220) -> (w225:dbl[][])  [unwired: 1 in]
                  n143 = Replace Array Subset(array=w221, new element=w222, index (row)=w220) -> (w219:dbl[][])  [unwired: 1 in]
                  n144 = Array Size(array=w246) -> (size(s)=w235:i32)
                }
                "detected" <- w178
                "Box" <- w195
                n145 = Bundle(0, 1, "Centroid X"=w194) -> (→"Status":cluster{i32, i32, "Centroid X":dbl[][]})  [unwired: 1 in]
                n146 = Index Array(array=w187, index (row)=w196) -> (element=→"particles":T1)  [unwired: 1 in]
                n147 = call <vilib>:"Clear Errors.vi"("error in (no error)"=w186) -> ("error out"=w213:errorcluster)  [unwired: 6 in]
                n148 = local read "img to avg"() -> (w203:i32)
                n149 = local read "Numeric"() -> (w206:dbl)
                n150 = Increment(x=w203) -> (x+1=w202:i32)
                n151 = Greater Or Equal?(x=w206, y=w202) -> (x >= y?=w199:bool)
                n152 = Increment(x=w206) -> (x+1=w205:dbl)
                n153 = Select(t=0.0, s=w199, f=w205) -> (s? t:f=w204:dbl)
                n154 = local write "Numeric"(w204) -> ()
                n155 = Bundle By Name(cluster=w197, "thresholds"=w183) -> (w209:T36)
                n156 = for {
                  tunnel: w179 -> [w289] mode=indexing
                  tunnel: w192 -> [w296] mode=indexing
                  shift-right: [w291] -> w214
                  shift-left: "" ("GUIdevice 7") -> [w294]
                  tunnel: [w284] -> w216 mode=indexing
                  tunnel: "Detection Rate" -> [w288]
                  tunnel: w204 -> [w286]
                  n157 = local read "img to avg"() -> (w290:i32)
                  n158 = Greater Or Equal?(x=w289, y=w290) -> (x >= y?=w285:bool)
                  n159 = Multiply(x=w288, y=w286) -> (x*y=w287:dbl)
                  n160 = Greater Or Equal?(x=w289, y=w287) -> (x >= y?=w283:bool)
                  n161 = And(x=w285, y=w283) -> (x .and. y?=w284:bool)
                  n162 = Select(t=w296, s=w284, f="") -> (s? t:f=w292:string)
                  n163 = Concatenate Strings(w294, "\t", w292) -> (w291:string)
                }
                n164 = call <vilib>:"Add State(s) to Queue__jki_lib_state_machine.vi"("State(s) in (\"\")"=w174, "State(s) at Back (\"\")"="Device Ini" ("State(s) at Back (\"\")")) -> ("States Out"=w173:string)  [unwired: 13 in]
                n165 = Bundle By Name(cluster=w209, "Centroid X"=w182, "Centroid Y"=w181, "Size"=w180) -> (w177:T36)
                n166 = Unbundle By Name(w177) -> ("img to avg"=w176:i32)
                n167 = case shown="True" w199 {
                  tunnel: w177 -> [w269 w276]
                  tunnel: [w269 w275] -> w200
                  tunnel: w176 -> [_ w271]
                  frame False {
                  }
                  frame True {
                    n168 = Decrement(x=w271) -> (x-1=w274:i32)
                    n169 = Initialize Array(0.0 ("element"), 12 ("dimension size"), w274) -> (w270:dbl[][])
                    n170 = Bundle By Name(cluster=w276, "Centroid X"=w270, "Centroid Y"=w270, "Size"=w270) -> (w275:T36)
                  }
                }
                n171 = Or Array Elements(Boolean array=w216) -> (logical OR=w215:bool)
                n172 = case shown="True" w215 {
                  tunnel: w214 -> [_ w281]
                  tunnel: w173 -> [w277 w279]
                  tunnel: [w277 w278] -> w201
                  frame False {
                  }
                  frame True {
                    n173 = call <vilib>:"Build State String with Arguments__jki_lib_state_machine.vi"("Arguments (\"\")"=w281, "State"="detected") -> ("State with Arguments"=w280:string)  [unwired: 4 in]
                    n174 = call <vilib>:"Add State(s) to Queue__jki_lib_state_machine.vi"("State(s) in (\"\")"=w279, "State(s) at Back (\"\")"=w280) -> ("States Out"=w278:string)  [unwired: 13 in]
                  }
                }
              }
              event "stop": Value Change {
                # "Exit Button Value Change (pressed) Event\n(this executes Macro: Exit to terminate the VI)"
                n175 = event-data() -> ()  [unwired: 1 in, 6 out]
                n176 = call <vilib>:"Add State(s) to Queue__jki_lib_state_machine.vi"("State(s) in Front (\"\")"="Macro: Exit", "State(s) in (\"\")"=w301) -> ("States Out"=w300:string)  [unwired: 13 in]
              }
              event Value Change {
                n177 = event-data() -> ()  [unwired: 1 in, 6 out]
                n178 = property on="Set Centriod Target" class="Bool (strict)"("Value"=FALSE) -> ()  [unwired: 2 in, 2 out]
                n179 = Unbundle By Name(w312) -> ("active ccd"=w304:i32, "Centroid X"=w303:dbl[][], "Centroid Y"=w302:dbl[][])
                n180 = Index Array(array=w308, index=w304) -> (element=w307:string)
                n181 = Concatenate Strings("Do want to update the target of " ("message"), w307, "?" ("string")) -> (w305:string)
                n182 = Two Button Dialog(message=w305) -> (T button?=w311:bool)  [unwired: 2 in]
                n183 = case shown="True" w311 {
                  tunnel: w310 -> [_ w323]
                  tunnel: w304 -> [_ w322]
                  tunnel: w303 -> [_ w329]
                  tunnel: w302 -> [_ w324]
                  frame False {
                  }
                  frame True {
                    n184 = Index Array(array=w329, index (row)=w322) -> (element=w328:dbl[])  [unwired: 1 in]
                    n185 = Index Array(array=w324, index (row)=w322) -> (element=w325:dbl[])  [unwired: 1 in]
                    n186 = Index Array(array=w323, index=w322) -> (element=w321:T30)
                    n187 = Unbundle By Name(w321) -> ("Target.X::12"=w320:refnum<vi>, "Target.Y::12"=w318:refnum<vi>)
                    n188 = Reverse 1D Array(array=w328) -> (reversed array=w327:dbl[])
                    n189 = Reverse 1D Array(array=w325) -> (reversed array=w326:dbl[])
                    n190 = Index Array(array=w327) -> (element=w319:dbl)  [unwired: 1 in]
                    n191 = Index Array(array=w326) -> (element=w317:dbl)  [unwired: 1 in]
                    n192 = property class="DigNum (strict)"(reference=w320, "Val(Sgnl)"=w319) -> ()  [unwired: 1 in, 2 out]
                    n193 = property class="DigNum (strict)"(reference=w318, "Val(Sgnl)"=w317) -> ()  [unwired: 1 in, 2 out]
                  }
                }
                n194 = call <vilib>:"Add State(s) to Queue__jki_lib_state_machine.vi"("State(s) in (\"\")"=w316) -> ("States Out"=w315:string)  [unwired: 14 in]
              }
              event "Feedback Global": Value Change {
                # "Exit Button Value Change (pressed) Event\n(this executes Macro: Exit to terminate the VI)"
                n195 = event-data() -> ("NewVal"=w332:bool)  [unwired: 1 in, 5 out]
                n196 = call <vilib>:"Add State(s) to Queue__jki_lib_state_machine.vi"("State(s) in (\"\")"=w335) -> ("States Out"=w334:string)  [unwired: 14 in]
                n197 = Bundle By Name(cluster=w331, "Feedback global"=w332) -> (w330:T36)
              }
              event Value Change {
                n198 = event-data() -> ()  [unwired: 1 in, 6 out]
                n199 = call <vilib>:"Add State(s) to Queue__jki_lib_state_machine.vi"("State(s) in Front (\"\")"="Move Config", "State(s) in (\"\")"=w340) -> ("States Out"=w339:string)  [unwired: 13 in]
              }
              event Value Change {
                n200 = event-data() -> ()  [unwired: 1 in, 6 out]
                n201 = call <vilib>:"Add State(s) to Queue__jki_lib_state_machine.vi"("State(s) in Front (\"\")"="Detection Config", "State(s) in (\"\")"=w345) -> ("States Out"=w344:string)  [unwired: 13 in]
              }
              event "associated motors": Value Change {
                n202 = event-data() -> ()  [unwired: 1 in, 6 out]
                n203 = call <vilib>:"Add State(s) to Queue__jki_lib_state_machine.vi"("State(s) in (\"\")"=w350, "State(s) at Back (\"\")"="Motor Config" ("State(s) at Back (\"\")")) -> ("States Out"=w349:string)  [unwired: 13 in]
              }
              event "Reset History": Value Change {
                n204 = event-data() -> ()  [unwired: 1 in, 6 out]
                n205 = call <vilib>:"Add State(s) to Queue__jki_lib_state_machine.vi"("State(s) in (\"\")"=w356, "State(s) at Back (\"\")"="Reset History" ("State(s) at Back (\"\")")) -> ("States Out"=w355:string)  [unwired: 13 in]
                n206 = property on="Reset History" class="Bool (strict)"("Value"=FALSE ("Reset History")) -> ()  [unwired: 2 in, 2 out]
              }
              event "Save Config": Value Change {
                n207 = event-data() -> ()  [unwired: 1 in, 6 out]
                n208 = call <vilib>:"Add State(s) to Queue__jki_lib_state_machine.vi"("State(s) in (\"\")"=w361, "State(s) at Back (\"\")"="Save Config" ("State(s) at Back (\"\")")) -> ("States Out"=w360:string)  [unwired: 13 in]
              }
              event "Load Config": Value Change {
                n209 = event-data() -> ()  [unwired: 1 in, 6 out]
                n210 = call "File Dialog2"("pattern (all files)"="*.cfg", "pattern label"="config") -> ("selected path"=w365:path)  [unwired: 10 in, 3 out]
                n211 = Path To String(path=w365) -> (string=w363:string)
                "config path" <- w363
                n212 = call <vilib>:"Build State String with Arguments__jki_lib_state_machine.vi"("Arguments (\"\")"=w363, "State"="Load Config" ("State(s) at Back (\"\")")) -> ("State with Arguments"=w362:string)  [unwired: 4 in]
                n213 = call <vilib>:"Add State(s) to Queue__jki_lib_state_machine.vi"("State(s) in (\"\")"=w371, "State(s) at Back (\"\")"=w362) -> ("States Out"=w370:string)  [unwired: 13 in]
              }
              event "Save Stats": Value Change {
                n214 = event-data() -> ()  [unwired: 1 in, 6 out]
                n215 = call <vilib>:"Add State(s) to Queue__jki_lib_state_machine.vi"("State(s) in (\"\")"=w376, "State(s) at Back (\"\")"="Save Stats" ("State(s) at Back (\"\")")) -> ("States Out"=w375:string)  [unwired: 13 in]
              }
              event "active CCDs": Value Change {
                n216 = event-data() -> ("NewVal"=w382:i32)  [unwired: 1 in, 5 out]
                n217 = Unbundle By Name(w378) -> ("active cams"=w377:string[])
                n218 = Index Array(array=w377, index=w382) -> (element=w380:string)
                n219 = call <vilib>:"Build State String with Arguments__jki_lib_state_machine.vi"("Arguments (\"\")"=w380, "State"="active" ("State(s) at Back (\"\")")) -> ("State with Arguments"=w379:string)  [unwired: 4 in]
                n220 = call <vilib>:"Add State(s) to Queue__jki_lib_state_machine.vi"("State(s) in (\"\")"=w385, "State(s) at Back (\"\")"=w379) -> ("States Out"=w384:string)  [unwired: 13 in]
              }
              event "Left", "Right": Value Change {
                n221 = event-data() -> ("CtlRef"=w394:refnum<vi>)  [unwired: 1 in, 5 out]
                n222 = property class="Bool (strict)"(reference=w394, error in=w391) -> (reference out=w393:refnum<vi>, error out=w392:errorcluster, "Label.Text"=w388:string)
                n223 = property class="Bool (strict)"(reference=w393, error in=w392, "Value"=FALSE) -> (error out=w390:errorcluster)  [unwired: 1 out]
                n224 = call <vilib>:"Build State String with Arguments__jki_lib_state_machine.vi"("Arguments (\"\")"=w388, "State"="ManMove X") -> ("State with Arguments"=w387:string)  [unwired: 4 in]
                n225 = call <vilib>:"Add State(s) to Queue__jki_lib_state_machine.vi"("State(s) in (\"\")"=w397, "State(s) at Back (\"\")"=w387) -> ("States Out"=w396:string)  [unwired: 13 in]
              }
              event "Tab Control 2": Value Change {
                n226 = event-data() -> ()  [unwired: 1 in, 6 out]
                n227 = call <vilib>:"Add State(s) to Queue__jki_lib_state_machine.vi"("State(s) in (\"\")"=w399, "State(s) at Back (\"\")"="stats" ("State")) -> ("States Out"=w398:string)  [unwired: 13 in]
              }
              event "Up", "Down": Value Change {
                n228 = event-data() -> ("CtlRef"=w411:refnum<vi>)  [unwired: 1 in, 5 out]
                n229 = property class="Bool (strict)"(reference=w411, error in=w408) -> (reference out=w410:refnum<vi>, error out=w409:errorcluster, "Label.Text"=w405:string)
                n230 = property class="Bool (strict)"(reference=w410, error in=w409, "Value"=FALSE) -> (error out=w407:errorcluster)  [unwired: 1 out]
                n231 = call <vilib>:"Build State String with Arguments__jki_lib_state_machine.vi"("Arguments (\"\")"=w405, "State"="ManMove Y") -> ("State with Arguments"=w404:string)  [unwired: 4 in]
                n232 = call <vilib>:"Add State(s) to Queue__jki_lib_state_machine.vi"("State(s) in (\"\")"=w414, "State(s) at Back (\"\")"=w404) -> ("States Out"=w413:string)  [unwired: 13 in]
              }
              event "Center": Value Change {
                n233 = event-data() -> ()  [unwired: 1 in, 6 out]
                n234 = call <vilib>:"Add State(s) to Queue__jki_lib_state_machine.vi"("State(s) in (\"\")"=w419, "State(s) at Back (\"\")"="Center" ("State(s) at Back (\"\")")) -> ("States Out"=w418:string)  [unwired: 13 in]
              }
              event "new tdms": Value Change {
                n235 = event-data() -> ()  [unwired: 1 in, 6 out]
                n236 = call <vilib>:"Add State(s) to Queue__jki_lib_state_machine.vi"("State(s) in (\"\")"=w424, "State(s) at Back (\"\")"="newtdms" ("State(s) at Back (\"\")")) -> ("States Out"=w423:string)  [unwired: 13 in]
              }
              event "device ini": Value Change {
                n237 = event-data() -> ()  [unwired: 1 in, 6 out]
                n238 = property on="device ini" class="Bool (strict)"("Value"=FALSE ("test")) -> ()  [unwired: 2 in, 2 out]
                n239 = call <vilib>:"Add State(s) to Queue__jki_lib_state_machine.vi"("State(s) in (\"\")"=w430, "State(s) at Back (\"\")"="Device Ini" ("State(s) at Back (\"\")")) -> ("States Out"=w429:string)  [unwired: 13 in]
              }
              event "img to avg": Value Change {
                n240 = event-data() -> ("NewVal"=w436:i32)  [unwired: 1 in, 5 out]
                n241 = Number To Decimal String(number=w436) -> (decimal integer string=w438:string)  [unwired: 1 in]
                n242 = call <vilib>:"Build State String with Arguments__jki_lib_state_machine.vi"("Arguments (\"\")"=w438, "State"="ImgToAvg" ("State(s) at Back (\"\")")) -> ("State with Arguments"=w433:string)  [unwired: 4 in]
                n243 = call <vilib>:"Add State(s) to Queue__jki_lib_state_machine.vi"("State(s) in (\"\")"=w434, "State(s) at Back (\"\")"=w433) -> ("States Out"=w432:string)  [unwired: 13 in]
              }
              event Panel Close? {
                # "Discard the event because we'll close the front panel ourselves in Macro: Exit"
                # "Close Panel button (pressed) Event\n(this executes Macro: Exit to terminate the VI)"
                n244 = event-data() -> ()  [unwired: 1 in, 1 out]
                n245 = call <vilib>:"Add State(s) to Queue__jki_lib_state_machine.vi"("State(s) in Front (\"\")"="Macro: Exit", "State(s) in (\"\")"=w444) -> ("States Out"=w443:string)  [unwired: 13 in]
                n246 = event-data("Discard?"=TRUE) -> ()  [unwired: 1 in, 1 out]
              }
            }
          }
          frame "---------- Core ----------" {
            # "Do not put any code in this frame.\n(it is a separator no-op)"
            n247 = call <vilib>:"Add State(s) to Queue__jki_lib_state_machine.vi"("State(s) in (\"\")"=w448) -> ("States Out"=w447:string)  [unwired: 14 in]
          }
          frame Default {
            w458 = 42 items=["No error", "Argument error", "Memory is full", "Out of zone", "End of file", "File already open", "Generic file I/O error", "File not found", "File permission error", "Disk is full", "Duplicate path", "Too many files open", "System feature not enabled", "Resource file not found", "Cannot add resource", "Resource not found", "Image not found", "Image memory error", "Pen does not exist", "Config type invalid", "Config token not found", "Config parse error", "Config memory error", "Bad external code format", "Bad external code offset", "External code not present", "Null window", "Destroy window error", "Null menu", "Print aborted", "Bad print record", "Print driver error", "Windows error during printing", "Memory error during printing", "Print dialog error", "Generic print error", "Invalid device refnum", "Device not found", "Device parameter error", "Device unit error", "Cannot open device", "Device call aborted", "Generic error", "Cancelled by user", "Object ID too low", "Object ID too high", "Object not in heap", "Unknown heap", "Unknown object (invalid DefProc)", "Unknown object (DefProc not in table)", "Message out of range", "Invalid (null) method", "Unknown message", "Manager call not supported", "Bad address", "Network operation in progress", "Network operation timed out", "Connection is busy", "Network attribute not supported", "Network error", "Address in use", "System out of memory", "Connection aborted", "Connection refused", "Not connected", "Already connected", "Connection closed", "Initialization error (interapplication manager)", "Bad occurrence", "Wait on unbound occurrence handler", "Occurrence queue overflow", "Datalog type conflict", "Unused", "Unrecognized type (interapplication manager)", "Memory corrupt", "Failed to make temporary DLL", "Old CIN version", "Drag socket not found", "Failed to load drop-object", "Failed to register OLE object", "Failed to release OLE object", "Format specifier type mismatch", "Unknown format specifier", "Too few format specifiers", "Too many format specifiers", "Scan failed", "Newer CIN version", "Error converting to variant", "Runtime menu error", "Password tampered", "Variant attribute not found", "Incompatible variant data type", "Event data is not available", "Event Store is not present", "Occurrence is not found", "Event Queue is not created", "Event info is not available", "Refnum passed is NULL", "Error retrieving Class GUID", "Error retrieving CoClass GUID", "Error retrieving TypeLib GUID.", "Bad built application magic bytes.", "Specific driver is different from the specific driver associated with the Logical Name.", "There is no session opened to the class driver.", "Max Error", "MAX - Error with config objects", "MAX - Error loading configuration", "MAX - Group not supported"]
            # "Current State"
            # "Do not delete, rename, or modify this frame.\n(this is used to capture unhandled states and typos)"
            # "Handle mistyped state name (developer tool)"
            n248 = Format Into String(format string="Software Exception: Unhandled State \"%s\"." ("message"), error in=w454, w449) -> (resulting string=w457:string, error out=w456:errorcluster)  [unwired: 1 in]
            n249 = call <vilib>:"Error Cluster From Error Code.vi"("show call chain? (False)"=TRUE, "error in (no error)"=w456, "error message (\"\")"=w457, "error code (0)"=w458) -> ("error out"=w455:errorcluster)  [unwired: 5 in]
            n250 = call <vilib>:"Add State(s) to Queue__jki_lib_state_machine.vi"("State(s) in (\"\")"=w453) -> ("States Out"=w452:string)  [unwired: 14 in]
          }
          frame "Initialize Core Data" {
            # "Do not delete, rename, or modify this frame.\n(this is used to determine panel behavior on exit)"
            # "originally closed?"
            # "exe?"
            # "If panel starts closed or is an EXE, then close it when we exit"
            n251 = property class="VI"() -> ("Front Panel.Open"=w468:bool)  [unwired: 2 in, 2 out]
            n252 = property class="App"() -> ("App.Kind"=w467:T15)  [unwired: 2 in, 2 out]
            n253 = control-ref of="Current VI Reference"() -> (w462:refnum<vi>)
            n254 = Not(x=w468) -> (.not. x?=w465:bool)
            n255 = Equal?(x=w467, y=T15."Run Time System" ("Application:Kind")) -> (x = y?=w464:bool)
            n256 = Or(x=w465, y=w464) -> (x .or. y?=w463:bool)
            n257 = Bundle By Name(cluster=w461, "Core.Current VI Reference"=w462, "Core.Close Panel on Exit?"=w463) -> (w460:T36)
            n258 = call <vilib>:"Add State(s) to Queue__jki_lib_state_machine.vi"("State(s) in (\"\")"=w471) -> ("States Out"=w470:string)  [unwired: 14 in]
          }
          frame "Error Handler" {
            # "Unhandled Error -- Display it"
            # "Handle any errors here.\nYou can also output any states to clean-up after errors occur"
            # "Clear error"
            n259 = call <vilib>:"General Error Handler.vi"("error in (no error)"=w473) -> ()  [unwired: 10 in, 5 out]
            n260 = call <vilib>:"Add State(s) to Queue__jki_lib_state_machine.vi"("State(s) in Front (\"\")"="/* Post Error States", "State(s) in (\"\")"=w477) -> ("States Out"=w476:string)  [unwired: 13 in]
          }
          frame "Exit" {
            # "Do not put any code in this frame.\n(No errors that occur here will be handled.)"
            n261 = call <vilib>:"Add State(s) to Queue__jki_lib_state_machine.vi"("State(s) in (\"\")"=w482) -> ("States Out"=w481:string)  [unwired: 14 in]
          }
          frame "---------- Data ----------" {
            # "Do not put any code in this frame.\n(It is a separator no-op. You can make a copy of this frame to create a new Data frame)"
            n262 = call <vilib>:"Add State(s) to Queue__jki_lib_state_machine.vi"("State(s) in (\"\")"=w486) -> ("States Out"=w485:string)  [unwired: 14 in]
          }
          frame "Data: Initialize" {
            w490 = bool[] [FALSE, FALSE, FALSE, FALSE, TRUE, TRUE, TRUE, FALSE, FALSE, FALSE, FALSE, FALSE]  # detected
            w500 = bool[] [FALSE, FALSE, FALSE, FALSE, FALSE, FALSE, FALSE, FALSE, FALSE, FALSE, FALSE, TRUE]  # speedmode Y
            w501 = bool[] [FALSE, FALSE, FALSE, FALSE, FALSE, FALSE, FALSE, FALSE, FALSE, FALSE, FALSE, TRUE]  # speedmode X
            w503 = cluster{"Lower value":sgl, "Upper value":sgl}[] [{"Lower value"=93.0, "Upper value"=255.0}, {"Lower value"=105.0, "Upper value"=255.0}, {"Lower value"=0.0, "Upper value"=255.0}, {"Lower value"=127.0, "Upper value"=255.0}, {"Lower value"=0.0, "Upper value"=255.0}, {"Lower value"=0.0, "Upper value"=255.0}, {"Lower value"=0.0, "Upper value"=255.0}, {"Lower value"=0.0, "Upper value"=255.0}, {"Lower value"=0.0, "Upper value"=255.0}, {"Lower value"=0.0, "Upper value"=255.0}, {"Lower value"=0.0, "Upper value"=255.0}, {"Lower value"=0.0, "Upper value"=255.0}]  # thresholds
            w510 = FALSE  # Feedback global
            w512 = 0  # active ccd
            w496 = 2  # img to avg
            w523 = T37 {"Current VI Reference"=refnum, "Close Panel on Exit?"=FALSE}  # Core
            # "Initialize the shift-register data, here.\n(data names are defined by what you wire into the bundle function)"
            n263 = disable-structure shown="Disabled" {
              disable-tunnel: w493 -> [w535 _]
              disable-tunnel: [w534 _] -> w492
              disable-tunnel: w491 -> [w533 _]
              disable-tunnel: [w532 _] -> _
              disable-tunnel: w489 -> [w526 _]
              frame Disabled {
                n264 = TDMS Open(6:FALSE ("disable buffering (T)"), 7:enum16{"1.0", "2.0"}."2.0" ("file format version (2.0)"), 8:w535, 10:T16."create or replace" ("operation"), 11:w533) -> (0:w530:errorcluster, 3:w531:refnum<k34>)  [unwired: 2 in]
                n265 = call "TDMSbuffersize.vi"("error in (no error)"=w530, "group names"=w526, "Data Value Reference in"=w531) -> ("error out"=w534:errorcluster, "Data Value Reference out"=w532:refnum<k34>)  [unwired: 7 in]
              }
              frame Enabled {
              }
            }
            n266 = call <vilib>:"Add State(s) to Queue__jki_lib_state_machine.vi"("State(s) in Front (\"\")"="newtdms" ("State(s) in Front (\"\")"), "State(s) in (\"\")"=w525) -> ("States Out"=w524:string)  [unwired: 13 in]
            n267 = Bundle("Core"=w523, "detection para"="detection para", "thresholds"=w503, "Centroid X"="Centroid X", "Centroid Y"="Centroid Y", "img to avg"=w496, "Mean Centroid X"="Mean Centroid X", "Mean Centroid Y"="Mean Centroid Y", "Offset X"="Offset X", "Offset Y"="Offset Y", "Offset X stats"="Offset X stats", "Offset Y stats"="Offset Y stats", "Size"="Size", "Mean Size"="Mean Size", "Time"="Time", "move properties"="move properties", "active axis refs 2"="active axis refs 2", "active ccd"=w512, "Feedback global"=w510, "Motor X"="Motor X", "Motor Y"="Motor Y", "active cams"="active cams", "Data Value Reference out"=refnum<k34> refnum, "active man refs"="active man refs", "detected"=w490, "speedmode X"=w501, "speedmode Y"=w500) -> (w495:T36)  [unwired: 1 in]
            n268 = Initialize Array(0.0 ("element"), 12 ("dimension size"), w496) -> (w499:dbl[][])
            n269 = Bundle By Name(cluster=w495, "Centroid X"=w499, "Centroid Y"=w499, "Size"=w499) -> (w494:T36)
          }
          frame "Data: Cleanup" {
            # "Cleanup any data and references, here.\n(this is called automatically, by the Macro: Exit)"
            n270 = Unbundle By Name(w536) -> ("Core.Current VI Reference"=w537:refnum<vi>)
            n271 = Close Reference(reference=w537, error in (no error)=w539) -> (error out=w538:errorcluster)
            n272 = call <vilib>:"Add State(s) to Queue__jki_lib_state_machine.vi"("State(s) in (\"\")"=w541) -> ("States Out"=w540:string)  [unwired: 14 in]
          }
          frame "---------- UI ----------" {
            # "Do not put any code in this frame.\n(It is a separator no-op. You can make a copy of this frame to create a new UI frame)"
            n273 = call <vilib>:"Add State(s) to Queue__jki_lib_state_machine.vi"("State(s) in (\"\")"=w545) -> ("States Out"=w544:string)  [unwired: 14 in]
          }
          frame "UI: Initialize" {
            # "Initialize the User Interface, here.\n(this is called automatically, by the Macro: Init)"
            n274 = call <vilib>:"Add State(s) to Queue__jki_lib_state_machine.vi"("State(s) in (\"\")"=w549) -> ("States Out"=w548:string)  [unwired: 14 in]
          }
          frame "UI: Cursor Set" {
            # "Argument"
            # "Set and Unset Cursor Busy.\n(Usage: \"UI: Cursor Set >> Busy|Idle\")"
            n275 = case shown="\"Idle\", Default" w550 {
              tunnel: w552 -> [w557 w559]
              tunnel: [w556 w558] -> w551
              frame "Idle", Default {
                n276 = call <vilib>:"Unset Busy.vi"("error in (no error)"=w557) -> ("error out"=w556:errorcluster)  [unwired: 10 in]
              }
              frame "Busy" {
                n277 = call <vilib>:"Set Busy.vi"("error in (no error)"=w559) -> ("error out"=w558:errorcluster)  [unwired: 9 in, 1 out]
              }
            }
            n278 = call <vilib>:"Add State(s) to Queue__jki_lib_state_machine.vi"("State(s) in (\"\")"=w555) -> ("States Out"=w554:string)  [unwired: 14 in]
          }
          frame "UI: Front Panel State" {
            # "Argument"
            # "Set Front Panel Open or Closed\n(Usage: \"UI: Front Panel State >> Open|Close\")"
            n279 = Unbundle By Name(w560) -> ("Core.Current VI Reference"=w562:refnum<vi>)
            n280 = case shown="\"Open\", Default" w561 {
              tunnel: w564 -> [w570 w581]
              tunnel: [w571 w582] -> w563
              tunnel: w562 -> [_ _]
              frame "Open", Default {
                n281 = property class="VI"(error in=w570) -> (reference out=w568:refnum<vi>, error out=w569:errorcluster, "Front Panel.Open"=w567:bool)  [unwired: 1 in]
                n282 = case shown="False" w567 {
                  tunnel: [w574 w577] -> w571
                  tunnel: w569 -> [w573 w577]
                  tunnel: w568 -> [w572 _]
                  frame False {
                    n283 = invoke class="VI" method="FP.Open"(reference=w572, error in=w573, "Activate"=TRUE, "State"=T17."Standard") -> (error out=w574:errorcluster)  [unwired: 1 in, 4 out]
                  }
                  frame True {
                  }
                }
              }
              frame "Close" {
                n284 = property class="VI"(error in=w581) -> (reference out=w579:refnum<vi>, error out=w580:errorcluster, "Front Panel.Open"=w578:bool)  [unwired: 1 in]
                n285 = case shown="True" w578 {
                  tunnel: [w583 w586] -> w582
                  tunnel: w580 -> [w583 w585]
                  tunnel: w579 -> [_ w584]
                  frame False {
                  }
                  frame True {
                    n286 = invoke class="VI" method="FP.Close"(reference=w584, error in=w585) -> (error out=w586:errorcluster)  [unwired: 1 in, 2 out]
                  }
                }
              }
            }
            n287 = call <vilib>:"Add State(s) to Queue__jki_lib_state_machine.vi"("State(s) in (\"\")"=w566) -> ("States Out"=w565:string)  [unwired: 14 in]
          }
          frame "---------- Macro ----------" {
            # "Do not put any code in this frame.\n(It is a separator no-op. You can make a copy of this frame to create a new Macro frame)"
            n288 = call <vilib>:"Add State(s) to Queue__jki_lib_state_machine.vi"("State(s) in (\"\")"=w590) -> ("States Out"=w589:string)  [unwired: 14 in]
          }
          frame "Macro: Initialize" {
            # "Initialization Macro\n(This is called once, when the VI starts)"
            n289 = property on="img to avg" class="DigNum (strict)"() -> ("Value"=w592:i32)  [unwired: 2 in, 2 out]
            n290 = Number To Decimal String(number=w592) -> (decimal integer string=w594:string)  [unwired: 1 in]
            n291 = call <vilib>:"Build State String with Arguments__jki_lib_state_machine.vi"("Arguments (\"\")"=w594, "State"="ImgToAvg") -> ("State with Arguments"=w591:string)  [unwired: 4 in]
            n292 = call <vilib>:"Add State(s) to Queue__jki_lib_state_machine.vi"("State(s) in Front (\"\")"="Data: Initialize\nInitialize Core Data\nUI: Initialize\nUI: Front Panel State >> Open\nDevice Ini >> 3000", "State(s) in (\"\")"=w599, "State(s) at Back (\"\")"=w591) -> ("States Out"=w598:string)  [unwired: 12 in]
          }
          frame "Macro: Exit" {
            # "Exit Macro\n(This is called once, when the VI exits)"
            n293 = Unbundle By Name(w601) -> ("Core.Close Panel on Exit?"=w600:bool)
            n294 = Select(t="UI: Front Panel State >> Close", s=w600, f="") -> (s? t:f=w604:string)
            n295 = call <vilib>:"Add State(s) to Queue__jki_lib_state_machine.vi"("State(s) in (\"\")"=w604, "State(s) at Back (\"\")"="Data: Cleanup\nExit") -> ("States Out"=w602:string)  [unwired: 13 in]
            n296 = call <vilib>:"Add State(s) to Queue__jki_lib_state_machine.vi"("State(s) in Front (\"\")"=w602, "State(s) in (\"\")"=w609) -> ("States Out"=w608:string)  [unwired: 13 in]
          }
          frame "---------- Ini and Configure ----------" {
            # "Template Separator\n(You can make a copy of, or modify, this frame)"
            n297 = call <vilib>:"Add State(s) to Queue__jki_lib_state_machine.vi"("State(s) in (\"\")"=w613) -> ("States Out"=w612:string)  [unwired: 14 in]
          }
          frame "Device Ini" {
            # "Your code here.\n(You can make a copy of, or modify, this frame)"
            n298 = Empty String/Path?(string/path=w632) -> (empty?=w631:bool)
            n299 = flat-sequence {
              tunnel: w616 -> [w639]
              tunnel: [w639] -> w617
              tunnel: w615 -> [w638]
              tunnel: w617 -> [w644]
              tunnel: [w642] -> w614
              frame #0 {
                n300 = Wait (ms)(milliseconds to wait=w638) -> ()  [unwired: 1 out]
              }
              frame #1 {
                n301 = local read "Array 3"() -> (w640:sgl[])
                n302 = disable-structure shown="Disabled" {
                  disable-tunnel: w644 -> [w647 _]
                  disable-tunnel: [w645 _] -> _
                  frame Disabled {
                    n303 = for {
                      tunnel: w647 -> [w648] mode=indexing
                      shift-right: [w650] -> w645
                      shift-left: string[] [] -> [w651]
                      n304 = call "send command.vi"("Device Name"=w648) -> ("status"=w652:bool)  [unwired: 4 in]
                      n305 = Wait (ms)(milliseconds to wait=u32 1) -> ()  [unwired: 1 out]
                      n306 = case shown="True" w652 {
                        tunnel: w651 -> [w653 w656]
                        tunnel: [w653 w655] -> w650
                        tunnel: w648 -> [_ w654]
                        frame False {
                        }
                        frame True {
                          n307 = Build Array (concatenate)(w656, w654) -> (w655:string[])
                        }
                      }
                    }
                  }
                  frame Enabled {
                  }
                }
                n308 = for {
                  tunnel: w644 -> [w659] mode=indexing
                  shift-right: [w664] -> w642
                  shift-left: string[] [] -> [w665]
                  tunnel: [w658] -> w641 mode=indexing
                  shift-right: [w662] -> _
                  shift-left: w640 -> [w662]
                  i -> [w663]
                  n309 = call "IMAQ Histograph"("Image"=w659) -> ("error out"=w657:errorcluster, "Mean Value"=w658:sgl)  [unwired: 7 in, 2 out]
                  n310 = Index Array(array=w662, index=w663) -> (element=w661:sgl)
                  n311 = call <vilib>:"Clear Errors.vi"("error in (no error)"=w657) -> ()  [unwired: 6 in, 1 out]
                  n312 = Equal?(x=w658, y=w661) -> (x = y?=w660:bool)
                  n313 = case shown="False" w660 {
                    tunnel: w665 -> [w668 w669]
                    tunnel: [w667 w669] -> w664
                    tunnel: w659 -> [w666 _]
                    frame False {
                      n314 = Build Array (concatenate)(w668, w666) -> (w667:string[])
                    }
                    frame True {
                    }
                  }
                }
                "Array 3" <- w641
              }
            }
            n315 = case shown="False" w631 {
              tunnel: w632 -> [w703 _]
              tunnel: [w702 0] -> w615
              frame False {
                n316 = Decimal String To Number(string=w703) -> (number=w702:i32)  [unwired: 2 in, 1 out]
              }
              frame True {
              }
            }
            n317 = Unbundle By Name(w630) -> ("active cams"=w623:string[])
            n318 = call <vilib>:"Add State(s) to Queue__jki_lib_state_machine.vi"("State(s) in (\"\")"=w637) -> ("States Out"=w625:string)  [unwired: 14 in]
            n319 = Equal?(x=w623, y=w614) -> (x = y?=w629:bool[])
            n320 = Empty Array?(array=w623) -> (empty?=w628:bool)
            n321 = Not(x=w628) -> (.not. x?=w627:bool)
            n322 = Build Array (concatenate)(w629, w627) -> (w626:bool[])
            n323 = Array Size(array=w614) -> (size(s)=w622:i32)
            n324 = Array Size(array=w623) -> (size(s)=w621:i32)
            n325 = And Array Elements(Boolean array=w626) -> (logical AND=w619:bool)
            n326 = Equal?(x=w622, y=w621) -> (x = y?=w620:bool)
            n327 = And(x=w620, y=w619) -> (x .and. y?=w618:bool)
            n328 = case shown="False" w618 {
              tunnel: [w684 w701] -> w636
              tunnel: w635 -> [_ _]
              tunnel: w634 -> [w681 w700]
              tunnel: [w681 w700] -> w633
              tunnel: w630 -> [w677 w701]
              tunnel: w614 -> [w678 _]
              tunnel: w625 -> [w683 w699]
              tunnel: [w671 w699] -> w624
              frame False {
                n329 = property on="active CCDs" class="LstBox (strict)"("Item Names"=w678) -> ()  [unwired: 2 in, 2 out]
                n330 = Array Size(array=w678) -> (size(s)=w691:i32)
                n331 = Initialize Array(0.0 ("element"), w691, 0 ("dimension size")) -> (w686:dbl[][])
                n332 = Unbundle By Name(w677) -> ("img to avg"=w676:i32)
                n333 = Bundle By Name(cluster=w677, "active cams"=w678) -> (w685:T36)
                n334 = Initialize Array(0.0 ("element"), 12 ("dimension size"), w676) -> (w675:dbl[][])
                n335 = Bundle By Name(cluster=w685, "Offset X stats"=w686, "Offset Y stats"=w686, "Centroid X"=w675, "Centroid Y"=w675, "Mean Centroid X"=w686, "Mean Centroid Y"=w686, "Offset X"=w686, "Offset Y"=w686, "Size"=w675, "Mean Size"=w686, "Motor X"=w686, "Motor Y"=w686) -> (w684:T36)
                n336 = for {
                  N: 1 -> [_]
                  shift-right: [w693] -> w689
                  shift-left: timestamp[][] [] ("Time") -> [w695]
                  n337 = for {
                    N: 12 -> [_]
                    tunnel: w695 -> [w698] mode=indexing
                    tunnel: [w696] -> w693 mode=indexing
                    n338 = Get Date/Time In Seconds() -> (seconds since 1Jan1904=w697:timestamp)
                    n339 = Build Array (concatenate)(w698, w697) -> (w696:timestamp[])
                  }
                }
                n340 = property on="config path" class="Str"() -> ("Value"=w673:string)  [unwired: 2 in, 2 out]
                n341 = call <vilib>:"Add State(s) to Queue__jki_lib_state_machine.vi"("State(s) in Front (\"\")"="Move Config\nMotor Config\nDetection Config\nactive\nCenter" ("State(s) in Front (\"\")"), "State(s) in (\"\")"=w683) -> ("States Out"=w672:string)  [unwired: 13 in]
                n342 = call <vilib>:"Build State String with Arguments__jki_lib_state_machine.vi"("Arguments (\"\")"=w673, "State"="Load Config" ("State(s) in Front (\"\")")) -> ("State with Arguments"=w670:string)  [unwired: 4 in]
                n343 = call <vilib>:"Add State(s) to Queue__jki_lib_state_machine.vi"("State(s) in (\"\")"=w672, "State(s) at Back (\"\")"=w670) -> ("States Out"=w671:string)  [unwired: 13 in]
                n344 = property on="Time" class="Arr (strict)"("Value"=w689) -> ()  [unwired: 2 in, 2 out]
                "name array" <- w678
              }
              frame True {
              }
            }
          }
          frame "Load Config" {
            # "Your code here.\n(You can make a copy of, or modify, this frame)"
            n345 = Unbundle By Name(w746) -> ("detection para"=w752:T3[], "move properties"=w749:T2[], "thresholds"=w742:cluster{"Lower value":sgl, "Upper value":sgl}[])
            n346 = Empty String/Path?(string/path=w709) -> (empty?=w708:bool)
            n347 = case shown="False" w708 {
              tunnel: [w762 T5 {"CCDs"=[], "move properties"=[], "detection para"=[], "thresholds"=[], "Value"={"Motor CCD 1"=0, "Motor CCD 2"=0, "Motor CCD 3"=0, "Motor CCD 4"=0, "Motor CCD 5"=0, "Motor CCD 6"=0, "Motor CCD 7"=0, "Motor CCD 8"=0, "Motor CCD 9"=0, "Motor CCD 10"=0, "Motor CCD 11"=0, "Motor CCD 12"=0}} ("output cluster 2")] -> w754
              tunnel: [w760 w769] -> w713
              tunnel: w710 -> [w759 w769]
              tunnel: w709 -> [w758 _]
              frame False {
                n348 = String To Path(string=w758) -> (path=w757:path)
                n349 = Open/Create/Replace File(file path (use dialog)=w757, error in=w759, operation (0:open)=T18."open or create") -> (refnum out=w764:refnum<file>, error out=w765:errorcluster)  [unwired: 3 in, 1 out]
                n350 = Read from Binary File(5:"output cluster 2", 8:w765, 11:w764) -> (0:w766:errorcluster, 2:w762:T5, 3:w767:refnum<file>)  [unwired: 3 in, 1 out]
                n351 = Close File(refnum=w767, error in=w766) -> (error out=w760:errorcluster)  [unwired: 1 out]
              }
              frame True {
              }
            }
            n352 = property on="Load Config" class="Bool (strict)"("Value"=FALSE ("Load Config")) -> ()  [unwired: 2 in, 2 out]
            n353 = Unbundle By Name(w754) -> ("Value"=w740:T7, "CCDs"=w753:string[], "detection para"=w751:T3[], "move properties"=w750:T2[], "thresholds"=w743:cluster{"Lower value":sgl, "Upper value":sgl}[])
            n354 = Cluster To Array(cluster=w740) -> (array=w741:u16[])
            n355 = call <vilib>:"Add State(s) to Queue__jki_lib_state_machine.vi"("State(s) in (\"\")"=w756, "State(s) at Back (\"\")"="Motor Config" ("State(s) at Back (\"\")")) -> ("States Out"=w755:string)  [unwired: 13 in]
            n356 = for {
              tunnel: w753 -> [w785]
              tunnel: w751 -> [w787]
              tunnel: w750 -> [w786]
              shift-right: [w779] -> w748
              shift-left: w752 -> [w784]
              shift-right: [w777] -> w747
              shift-left: w749 -> [w783]
              tunnel: w744 -> [w782] mode=indexing
              tunnel: w743 -> [w778]
              shift-right: [w774] -> w706
              shift-left: w742 -> [w776]
              tunnel: w741 -> [w773]
              tunnel: [w770] -> w739 mode=indexing
              i -> [w771]
              n357 = call-poly <userlib>:"Filter 1D Array__ogtk.vi"("items to filter"=w782, "array"=w785) -> ("filtered item indices"=w788:i32[])  [unwired: 4 in, 1 out]
              n358 = Index Array(array=w788) -> (element=w772:i32)  [unwired: 1 in]
              n359 = Index Array(array=w773, index=w772) -> (element=w770:u16)
              n360 = Index Array(array=w787, index=w772) -> (element=w781:T3)
              n361 = Index Array(array=w786, index=w772) -> (element=w780:T2)
              n362 = Index Array(array=w778, index=w772) -> (element=w775:cluster{"Lower value":sgl, "Upper value":sgl})
              n363 = Replace Array Subset(array=w784, new element=w781, index=w771) -> (w779:T3[])
              n364 = Replace Array Subset(array=w783, new element=w780, index=w771) -> (w777:T2[])
              n365 = Replace Array Subset(array=w776, new element=w775, index=w771) -> (w774:cluster{"Lower value":sgl, "Upper value":sgl}[])
            }
            n366 = Array Size(array=w706) -> (size(s)=→"size(s) 6":i32)
            n367 = Index Array(array=w739, index #1=0 ("index (row)"), index #2=1 ("index (row)"), index #3=2 ("index (row)"), index #4=3 ("index (row)"), index #5=4 ("index (row)"), index #6=5 ("index (row)"), index #7=6 ("index (row)"), index #8=7 ("index (row)"), index #9=8 ("index (row)"), index #10=9 ("index (row)"), index #11=10 ("index (row)"), index #12=11 ("index (row)")) -> (element #1=w726:u16, element #2=w725:u16, element #3=w724:u16, element #4=w723:u16, element #5=w722:u16, element #6=w721:u16, element #7=w720:u16, element #8=w719:u16, element #9=w718:u16, element #10=w717:u16, element #11=w716:u16, element #12=w715:u16)
            n368 = Bundle By Name(cluster=w740, "Motor CCD 1"=w726, "Motor CCD 2"=w725, "Motor CCD 3"=w724, "Motor CCD 4"=w723, "Motor CCD 5"=w722, "Motor CCD 6"=w721, "Motor CCD 7"=w720, "Motor CCD 8"=w719, "Motor CCD 9"=w718, "Motor CCD 10"=w717, "Motor CCD 11"=w716, "Motor CCD 12"=w715) -> (w714:T7)
            n369 = Bundle By Name(cluster=w746, "detection para"=w748, "move properties"=w747, "thresholds"=w706) -> (w745:T36)
            n370 = property on="associated motors" class="Clust (strict)"(error in=w713, "Val(Sgnl)"=w714) -> (error out=w712:errorcluster)  [unwired: 1 in, 1 out]
          }
          frame "Save Config" {
            # "Your code here.\n(You can make a copy of, or modify, this frame)"
            n371 = Unbundle By Name(w806) -> ("move properties"=w792:T2[], "detection para"=w801:T3[], "thresholds"=w789:cluster{"Lower value":sgl, "Upper value":sgl}[])
            n372 = property on="associated motors" class="Clust (strict)"() -> ("Value"=w800:T7)  [unwired: 2 in, 2 out]
            n373 = property on="Save Config" class="Bool (strict)"("Value"=FALSE ("Save Config")) -> ()  [unwired: 2 in, 2 out]
            n374 = local read "CCDs"() -> (w790:string[])
            n375 = call "File Dialog"("pattern (all files)"="*.cfg", "pattern label"="config") -> ("selected path"=w794:path)  [unwired: 10 in, 3 out]
            n376 = Bundle("CCDs"=w790, "move properties"=w792, "detection para"=w801, "thresholds"=w789, "Value"=w800) -> (w793:T5)  [unwired: 1 in]
            n377 = Open/Create/Replace File(file path (use dialog)=w794, error in=w798, operation (0:open)=T18."replace or create with confirmation") -> (refnum out=w802:refnum<file>, error out=w803:errorcluster)  [unwired: 3 in, 1 out]
            n378 = Write to Binary File(file (use dialog)=w802, data=w793, error in=w803) -> (refnum out=w805:refnum<file>, error out=w804:errorcluster)  [unwired: 3 in, 1 out]
            n379 = Close File(refnum=w805, error in=w804) -> (error out=w797:errorcluster)  [unwired: 1 out]
            n380 = call <vilib>:"Add State(s) to Queue__jki_lib_state_machine.vi"("State(s) in (\"\")"=w808) -> ("States Out"=w807:string)  [unwired: 14 in]
          }
          frame "active" {
            # "Your code here.\n(You can make a copy of, or modify, this frame)"
            n381 = Empty String/Path?(string/path=w823) -> (empty?=w822:bool)
            n382 = Unbundle By Name(w819) -> ("move properties"=w835:T2[], "detection para"=w831:T3[])  [unwired: 1 out]
            n383 = Unbundle By Name(w819) -> ("active axis refs 2"=w818:T11)
            n384 = call-poly <userlib>:"Filter 1D Array__ogtk.vi"("items to filter"=w823, "array"=w833) -> ("filtered item indices"=w836:i32[])  [unwired: 4 in, 1 out]
            n385 = Index Array(array=w836) -> (element=w820:i32)  [unwired: 1 in]
            n386 = Select(t=0, s=w822, f=w820) -> (s? t:f=w816:i32)
            n387 = Index Array(array=w818, index=w816) -> (element=w817:cluster{"Ref X":refnum<vi>, "Ref Y":refnum<vi>})
            n388 = Unbundle By Name(w817) -> ("Ref X"=w815:refnum<vi>, "Ref Y"=w814:refnum<vi>)
            n389 = Index Array(array=w835, index=w816) -> (element=w834:T2)
            n390 = Index Array(array=w831, index=w816) -> (element=w830:T3)
            n391 = property on="move config" class="Clust (strict)"(error in=w826, "Value"=w834) -> (error out=w824:errorcluster)  [unwired: 1 in, 1 out]
            n392 = property on="beam detection para" class="Clust (strict)"(error in=w824, "Value"=w830) -> (error out=w825:errorcluster)  [unwired: 1 in, 1 out]
            n393 = call <vilib>:"Add State(s) to Queue__jki_lib_state_machine.vi"("State(s) in (\"\")"=w838) -> ("States Out"=w837:string)  [unwired: 14 in]
            n394 = property class="DigNum (strict)"(reference=w815, error in=w825) -> (error out=w811:errorcluster, "Value"=w813:dbl)  [unwired: 1 out]
            n395 = Bundle By Name(cluster="active Axis ref 3", "Ref X"=w815, "Ref Y"=w814) -> (w828:cluster{"Ref X":refnum<vi>, "Ref Y":refnum<vi>})
            n396 = Bundle By Name(cluster=w819, "active ccd"=w816, "active man refs"=w828) -> (w832:T36)
            n397 = property on="Position 1" class="DigNum (strict)"(error in=w811, "Value"=w813) -> (error out=w810:errorcluster)  [unwired: 1 in, 1 out]
            n398 = property class="DigNum (strict)"(reference=w814, error in=w810) -> (error out=w809:errorcluster, "Value"=w812:dbl)  [unwired: 1 out]
            n399 = property on="Position 2" class="DigNum (strict)"(error in=w809, "Value"=w812) -> (error out=w827:errorcluster)  [unwired: 1 in, 1 out]
          }
          frame "Detection Config" {
            # "Your code here.\n(You can make a copy of, or modify, this frame)"
            n400 = Unbundle By Name(w843) -> ("detection para"=w839:T3[], "active ccd"=w844:i32)
            n401 = Replace Array Subset(array=w839, new element="beam detection para", index=w844) -> (w840:T3[])
            n402 = Bundle By Name(cluster=w843, "detection para"=w840) -> (w842:T36)
            n403 = call <vilib>:"Add State(s) to Queue__jki_lib_state_machine.vi"("State(s) in (\"\")"=w847) -> ("States Out"=w846:string)  [unwired: 14 in]
          }
          frame "Motor Config" {
            # "Your code here.\n(You can make a copy of, or modify, this frame)"
            n404 = Unbundle By Name("associated motors") -> ("Motor CCD 1"=w864:u16, "Motor CCD 2"=w865:u16, "Motor CCD 3"=w866:u16, "Motor CCD 4"=w859:u16, "Motor CCD 5"=w858:u16, "Motor CCD 6"=w857:u16, "Motor CCD 7"=w856:u16, "Motor CCD 8"=w855:u16, "Motor CCD 9"=w854:u16, "Motor CCD 10"=w853:u16, "Motor CCD 11"=w852:u16, "Motor CCD 12"=w851:u16)
            n405 = Build Array(w864, w865, w866, w859, w858, w857, w856, w855, w854, w853, w852, w851) -> (w850:u16[])
            n406 = local read "motor refs"() -> (w862:refnum<vi>[])
            n407 = Increment(x=w850) -> (x+1=w849:u16[])
            n408 = for {
              tunnel: w849 -> [w881] mode=indexing
              tunnel: w862 -> [w876]
              tunnel: [w870] -> w848 mode=indexing
              n409 = Multiply(x=w881, y=u16 2) -> (x*y=w877:u16)
              n410 = Subtract(x=w877, y=u16 2) -> (x-y=w875:u16)
              n411 = Subtract(x=w877, y=u16 1) -> (x-y=w874:u16)
              n412 = Index Array(array=w876, index=w875) -> (element=w873:refnum<vi>)
              n413 = Index Array(array=w876, index=w874) -> (element=w872:refnum<vi>)
              n414 = Bundle By Name(cluster="active Axis ref", "Ref X"=w873, "Ref Y"=w872) -> (w870:cluster{"Ref X":refnum<vi>, "Ref Y":refnum<vi>})
            }
            n415 = call <vilib>:"Add State(s) to Queue__jki_lib_state_machine.vi"("State(s) in (\"\")"=w869) -> ("States Out"=w868:string)  [unwired: 14 in]
            n416 = Bundle By Name(cluster=w861, "active axis refs 2"=w848) -> (w860:T36)
          }
          frame "Move Config" {
            # "Your code here.\n(You can make a copy of, or modify, this frame)"
            n417 = Unbundle By Name(w883) -> ("move properties"=w887:T2[], "active ccd"=w886:i32)
            n418 = Replace Array Subset(array=w887, new element="move config", index=w886) -> (w884:T2[])
            n419 = Bundle By Name(cluster=w883, "move properties"=w884) -> (w882:T36)
            n420 = call <vilib>:"Add State(s) to Queue__jki_lib_state_machine.vi"("State(s) in (\"\")"=w890) -> ("States Out"=w889:string)  [unwired: 14 in]
          }
          frame "----------Centroid & Move----------" {
            # "Template Separator\n(You can make a copy of, or modify, this frame)"
            n421 = call <vilib>:"Add State(s) to Queue__jki_lib_state_machine.vi"("State(s) in (\"\")"=w894) -> ("States Out"=w893:string)  [unwired: 14 in]
          }
          frame "detected" {
            n422 = Unbundle By Name(w899) -> ("Offset X"=w932:dbl[][], "Offset Y"=w931:dbl[][], "Size"=w930:dbl[][], "Mean Size"=w929:dbl[][], "Time"=w926:timestamp[][], "Motor X"=w908:dbl[][], "active axis refs 2"=w907:T11, "Motor Y"=w906:dbl[][])
            n423 = Spreadsheet String To Array(format string="%s", spreadsheet string=w911, array type (2D Dbl)=string[] []) -> (array=w902:string[])  [unwired: 1 in]
            n424 = for {
              tunnel: w903 -> [w946] mode=indexing
              tunnel: w902 -> [w945]
              tunnel: [w944] -> w901 mode=indexing
              n425 = for {
                tunnel: w946 -> [w949]
                tunnel: [w948] -> w943 mode=indexing
                tunnel: w945 -> [w947] mode=indexing
                n426 = Equal?(x=w949, y=w947) -> (x = y?=w948:bool)
              }
              n427 = Or Array Elements(Boolean array=w943) -> (logical OR=w944:bool)
            }
            n428 = Unbundle By Name(w899) -> ("Mean Centroid X"=w937:dbl[][], "Mean Centroid Y"=w936:dbl[][], "Centroid X"=w939:dbl[][], "Centroid Y"=w938:dbl[][])
            n429 = call <vilib>:"Add State(s) to Queue__jki_lib_state_machine.vi"("State(s) in (\"\")"=w910) -> ("States Out"=w909:string)  [unwired: 14 in]
            n430 = for {
              tunnel: w939 -> [w999]
              tunnel: w938 -> [w998]
              tunnel: w937 -> [w997]
              tunnel: w936 -> [w996]
              tunnel: [w995] -> w923 mode=indexing
              tunnel: [w994] -> w934 mode=indexing
              tunnel: w933 -> [w993] mode=indexing
              tunnel: w932 -> [w992]
              tunnel: w931 -> [w991]
              tunnel: [w990] -> w900 mode=indexing
              tunnel: [w989] -> w924 mode=indexing
              tunnel: w930 -> [w988]
              tunnel: w929 -> [w987]
              tunnel: [w986] -> w928 mode=indexing
              tunnel: w926 -> [w985]
              tunnel: [w984] -> w925 mode=indexing
              tunnel: w908 -> [w976]
              tunnel: w907 -> [w975]
              tunnel: w906 -> [w974]
              tunnel: [w954] -> w905 mode=indexing
              tunnel: [w953] -> w904 mode=indexing
              tunnel: w901 -> [w952]
              i -> [w951]
              n431 = Unbundle By Name(w993) -> ("Target.X::12"=w958:refnum<vi>, "Target.Y::12"=w957:refnum<vi>)
              n432 = Index Array(array=w976, index (row)=w951) -> (element=w979:dbl[])  [unwired: 1 in]
              n433 = Index Array(array=w975, index=w951) -> (element=w978:cluster{"Ref X":refnum<vi>, "Ref Y":refnum<vi>})
              n434 = Index Array(array=w974, index (row)=w951) -> (element=w983:dbl[])  [unwired: 1 in]
              n435 = Index Array(array=w952, index=w951) -> (element=w950:bool)
              n436 = Index Array(array=w997, index (row)=w951) -> (element=w970:dbl[])  [unwired: 1 in]
              n437 = Index Array(array=w996, index (row)=w951) -> (element=w971:dbl[])  [unwired: 1 in]
              n438 = Index Array(array=w999, index (row)=w951) -> (element=w973:dbl[])  [unwired: 1 in]
              n439 = Index Array(array=w998, index (row)=w951) -> (element=w972:dbl[])  [unwired: 1 in]
              n440 = Index Array(array=w992, index (row)=w951) -> (element=w966:dbl[])  [unwired: 1 in]
              n441 = Index Array(array=w991, index (row)=w951) -> (element=w965:dbl[])  [unwired: 1 in]
              n442 = Index Array(array=w988, index (row)=w951) -> (element=w963:dbl[])  [unwired: 1 in]
              n443 = Index Array(array=w987, index (row)=w951) -> (element=w962:dbl[])  [unwired: 1 in]
              n444 = Index Array(array=w985, index (row)=w951) -> (element=w959:timestamp[])  [unwired: 1 in]
              n445 = Unbundle By Name(w978) -> ("Ref X"=w977:refnum<vi>, "Ref Y"=w981:refnum<vi>)
              n446 = property class="DigNum (strict)"(reference=w958) -> ("Value"=w956:dbl)  [unwired: 1 in, 2 out]
              n447 = property class="DigNum (strict)"(reference=w957) -> ("Value"=w955:dbl)  [unwired: 1 in, 2 out]
              n448 = call <vilib>:"Std Deviation and Variance.vi"("X"=w973) -> ("mean"=w969:dbl)  [unwired: 1 in, 2 out]
              n449 = call <vilib>:"Std Deviation and Variance.vi"("X"=w972) -> ("mean"=w968:dbl)  [unwired: 1 in, 2 out]
              n450 = call <vilib>:"Std Deviation and Variance.vi"("X"=w963) -> ("mean"=w961:dbl)  [unwired: 1 in, 2 out]
              n451 = Get Date/Time In Seconds() -> (seconds since 1Jan1904=w960:timestamp)
              n452 = property class="DigNum (strict)"(reference=w977) -> ("Value"=w980:dbl)  [unwired: 1 in, 2 out]
              n453 = property class="DigNum (strict)"(reference=w981) -> ("Value"=w982:dbl)  [unwired: 1 in, 2 out]
              n454 = Subtract(x=w956, y=w969) -> (x-y=w967:dbl)
              n455 = Subtract(x=w955, y=w968) -> (x-y=w964:dbl)
              n456 = case shown="True" w950 {
                tunnel: [w1012 w1031] -> w995
                tunnel: [w1000 w1030] -> w994
                tunnel: [w1001 w1029] -> w990
                tunnel: [w1002 w1028] -> w989
                tunnel: [w1003 w1027] -> w986
                tunnel: [w1004 w1026] -> w984
                tunnel: w971 -> [w1010 w1025]
                tunnel: w970 -> [w1011 w1024]
                tunnel: w969 -> [_ w1023]
                tunnel: w968 -> [_ w1022]
                tunnel: w967 -> [_ w1021]
                tunnel: w966 -> [w1009 w1020]
                tunnel: w965 -> [w1008 w1019]
                tunnel: w964 -> [_ w1018]
                tunnel: w962 -> [w1007 w1017]
                tunnel: w961 -> [_ w1016]
                tunnel: w960 -> [w1005 w1015]
                tunnel: w959 -> [w1006 w1014]
                frame False {
                  w1013 = 0.0
                  n457 = Build Array (concatenate)(w1011, w1013) -> (w1012:dbl[])
                  n458 = Build Array (concatenate)(w1010, w1013) -> (w1000:dbl[])
                  n459 = Build Array (concatenate)(w1009, w1013) -> (w1001:dbl[])
                  n460 = Build Array (concatenate)(w1008, w1013) -> (w1002:dbl[])
                  n461 = Build Array (concatenate)(w1007, w1013) -> (w1003:dbl[])
                  n462 = Build Array (concatenate)(w1006, w1005) -> (w1004:timestamp[])
                }
                frame True {
                  n463 = Build Array (concatenate)(w1024, w1023) -> (w1031:dbl[])
                  n464 = Build Array (concatenate)(w1025, w1022) -> (w1030:dbl[])
                  n465 = Build Array (concatenate)(w1020, w1021) -> (w1029:dbl[])
                  n466 = Build Array (concatenate)(w1019, w1018) -> (w1028:dbl[])
                  n467 = Build Array (concatenate)(w1017, w1016) -> (w1027:dbl[])
                  n468 = Build Array (concatenate)(w1014, w1015) -> (w1026:timestamp[])
                }
              }
              n469 = Build Array (concatenate)(w979, w980) -> (w954:dbl[])
              n470 = Build Array (concatenate)(w983, w982) -> (w953:dbl[])
            }
            n471 = local write "Numeric"(0.0 ("Numeric")) -> ()
            n472 = Array Size(array=w900) -> (size(s)=w922:i32[])
            n473 = Index Array(array=w922, index=1) -> (element=w920:i32)
            "History Index" <- w920
            n474 = call <vilib>:"Add State(s) to Queue__jki_lib_state_machine.vi"("State(s) in (\"\")"=w909, "State(s) at Back (\"\")"="Check Move\ntdms" ("State(s) at Back (\"\")")) -> ("States Out"=w914:string)  [unwired: 13 in]
            n475 = Unbundle By Name(w899) -> ("img to avg"=w896:i32)
            n476 = Initialize Array(0.0 ("element"), 12 ("dimension size"), w896) -> (w895:dbl[][])
            n477 = Greater?(x=w920, y="History Size") -> (0:w918:bool)
            n478 = Bundle By Name(cluster=w899, "Centroid X"=w895, "Centroid Y"=w895, "Mean Centroid X"=w923, "Mean Centroid Y"=w934, "Offset X"=w900, "Offset Y"=w924, "Mean Size"=w928, "Size"=w895, "Time"=w925, "Motor X"=w905, "Motor Y"=w904) -> (w935:T36)
            n479 = Select(t="history" ("State(s) at Back (\"\")"), s=w918, f="") -> (s? t:f=w915:string)
            n480 = call <vilib>:"Add State(s) to Queue__jki_lib_state_machine.vi"("State(s) in (\"\")"=w914, "State(s) at Back (\"\")"=w915) -> ("States Out"=w913:string)  [unwired: 13 in]
          }
          frame "Check Move" {
            (unwired) "Device Ini" ("State(s) in Front (\"\")")
            n481 = Unbundle By Name(w1034) -> ("move properties"=w1046:T2[], "Mean Size"=w1045:dbl[][], "move properties"=w1044:T2[], "Offset X"=w1043:dbl[][], "Offset Y"=w1042:dbl[][], "active cams"=w1041:string[])
            n482 = for {
              tunnel: w1044 -> [w1074]
              tunnel: w1043 -> [w1072]
              tunnel: w1042 -> [w1070]
              tunnel: w1045 -> [w1078]
              tunnel: [w1094] -> w1040 mode=indexing
              tunnel: [w1090] -> w1039 mode=indexing
              tunnel: w1041 -> [w1079] mode=indexing
              tunnel: [w1112] -> w1047 mode=indexing
              tunnel: [w1111] -> w1037 mode=indexing
              tunnel: w1046 -> [w1077]
              tunnel: [w1088] -> w1036 mode=indexing
              tunnel: [w1083] -> w1035 mode=indexing
              tunnel: "Speedmode @" -> [w1082]
              tunnel: w1032 -> [w1080]
              n483 = call-poly <userlib>:"Filter 1D Array__ogtk.vi"("items to filter"=w1079, "array"=w1080) -> ("filtered item indices"=w1081:i32[])  [unwired: 4 in, 1 out]
              n484 = Index Array(array=w1081) -> (element=w1068:i32)  [unwired: 1 in]
              n485 = Index Array(array=w1077, index=w1068) -> (element=w1076:T2)
              n486 = Index Array(array=w1078, index (row)=w1068) -> (element=w1075:dbl[])  [unwired: 1 in]
              n487 = Index Array(array=w1074, index=w1068) -> (element=w1073:T2)
              n488 = Index Array(array=w1072, index (row)=w1068) -> (element=w1071:dbl[])  [unwired: 1 in]
              n489 = Index Array(array=w1070, index (row)=w1068) -> (element=w1069:dbl[])  [unwired: 1 in]
              n490 = Unbundle By Name(w1073) -> ("Tolerance [%]"=w1105:dbl)
              n491 = Reverse 1D Array(array=w1071) -> (reversed array=w1110:dbl[])
              n492 = Reverse 1D Array(array=w1069) -> (reversed array=w1109:dbl[])
              n493 = Reverse 1D Array(array=w1075) -> (reversed array=w1104:dbl[])
              n494 = Unbundle By Name(w1076) -> ("enable feedback"=w1093:bool)
              n495 = Index Array(array=w1110) -> (element=w1108:dbl)  [unwired: 1 in]
              n496 = Index Array(array=w1109) -> (element=w1107:dbl)  [unwired: 1 in]
              n497 = Index Array(array=w1104) -> (element=w1103:dbl)  [unwired: 1 in]
              n498 = Absolute Value(x=w1108) -> (abs(x)=w1089:dbl)
              n499 = Absolute Value(x=w1107) -> (abs(x)=w1086:dbl)
              n500 = Square Root(x=w1103) -> (sqrt(x)=w1102:dbl)
              n501 = Divide(x=w1105, y=100.0) -> (x/y=w1101:dbl)
              n502 = Multiply(x=w1102, y=w1101) -> (x*y=w1085:dbl)
              n503 = Not Equal To 0?(x=w1086) -> (x != 0?=w1091:bool)
              n504 = Not Equal To 0?(x=w1089) -> (x != 0?=w1096:bool)
              n505 = Greater Or Equal?(x=w1089, y=w1085) -> (x >= y?=w1095:bool)
              n506 = Greater Or Equal?(x=w1086, y=w1085) -> (x >= y?=w1092:bool)
              n507 = Divide(x=w1089, y=w1085) -> (x/y=w1087:dbl)
              n508 = Divide(x=w1086, y=w1085) -> (x/y=w1084:dbl)
              n509 = Compound Arithmetic op=AND(w1093, w1096, w1095) -> (w1094:bool)
              n510 = Compound Arithmetic op=AND(w1093, w1092, w1091) -> (w1090:bool)
              n511 = Boolean To (0,1)(Boolean=w1090) -> (0, 1=w1097:i16)
              n512 = Greater?(x=w1087, y=w1082) -> (0:w1088:bool)
              n513 = Greater?(x=w1084, y=w1082) -> (0:w1083:bool)
              n514 = Multiply(x=w1097, y=w1086) -> (x*y=w1098:dbl)
              n515 = Boolean To (0,1)(Boolean=w1094) -> (0, 1=w1100:i16)
              n516 = Multiply(x=w1100, y=w1089) -> (x*y=w1099:dbl)
              n517 = Bundle(w1098, "GUIdevice 8"=w1079) -> (w1111:cluster{dbl, "GUIdevice 8":string})  [unwired: 1 in]
              n518 = Bundle(w1099, "GUIdevice 8"=w1079) -> (w1112:cluster{dbl, "GUIdevice 8":string})  [unwired: 1 in]
            }
            "required X" <- w1040
            "required Y" <- w1039
            "speedmode X" <- w1036
            "speedmode Y" <- w1035
            n519 = case shown="True" "Align" {
              tunnel: w1047 -> [w1118 w1123]
              tunnel: w1037 -> [w1117 w1120]
              tunnel: [w1116 w1122] -> w1050
              tunnel: [w1115 w1119] -> w1049
              frame False {
                n520 = Sort 1D Array(array=w1117) -> (sorted array=w1114:cluster{dbl, "GUIdevice 8":string}[])
                n521 = Sort 1D Array(array=w1118) -> (sorted array=w1113:cluster{dbl, "GUIdevice 8":string}[])
                n522 = Reverse 1D Array(array=w1114) -> (reversed array=w1115:cluster{dbl, "GUIdevice 8":string}[])
                n523 = Reverse 1D Array(array=w1113) -> (reversed array=w1116:cluster{dbl, "GUIdevice 8":string}[])
              }
              frame True {
                w1121 = cluster{dbl, "GUIdevice 8":string}[] [] ("Array")
                n524 = for {
                  shift-right: [w1133] -> w1122
                  shift-left: w1121 -> [w1135]
                  tunnel: w1123 -> [w1134] mode=indexing
                  n525 = Unbundle(w1134) -> (w1137:dbl)  [unwired: 1 out]
                  n526 = Not Equal To 0?(x=w1137) -> (x != 0?=w1136:bool)
                  n527 = case shown="True" w1136 {
                    tunnel: w1135 -> [w1138 w1141]
                    tunnel: w1134 -> [_ w1140]
                    tunnel: [w1138 w1139] -> w1133
                    frame False {
                    }
                    frame True {
                      n528 = Build Array (concatenate)(w1141, w1140) -> (w1139:cluster{dbl, "GUIdevice 8":string}[])
                    }
                  }
                }
                n529 = for {
                  shift-right: [w1124] -> w1119
                  shift-left: w1121 -> [w1126]
                  tunnel: w1120 -> [w1125] mode=indexing
                  n530 = Unbundle(w1125) -> (w1128:dbl)  [unwired: 1 out]
                  n531 = Not Equal To 0?(x=w1128) -> (x != 0?=w1127:bool)
                  n532 = case shown="True" w1127 {
                    tunnel: w1126 -> [w1129 w1132]
                    tunnel: w1125 -> [_ w1131]
                    tunnel: [w1129 w1130] -> w1124
                    frame False {
                    }
                    frame True {
                      n533 = Build Array (concatenate)(w1132, w1131) -> (w1130:cluster{dbl, "GUIdevice 8":string}[])
                    }
                  }
                }
              }
            }
            n534 = call <vilib>:"Add State(s) to Queue__jki_lib_state_machine.vi"("State(s) in (\"\")"=w1053) -> ("States Out"=w1052:string)  [unwired: 14 in]
            n535 = Bundle By Name(cluster=w1034, "speedmode X"=w1036, "speedmode Y"=w1035) -> (w1033:T36)
            n536 = Index Array(array=w1049) -> (element=w1054:cluster{dbl, "GUIdevice 8":string})  [unwired: 1 in]
            n537 = Index Array(array=w1050) -> (element=w1055:cluster{dbl, "GUIdevice 8":string})  [unwired: 1 in]
            n538 = Empty Array?(array=w1049) -> (empty?=w1057:bool)
            n539 = Unbundle(w1055) -> (w1063:dbl)  [unwired: 1 out]
            n540 = Unbundle(w1054) -> (w1059:dbl)  [unwired: 1 out]
            n541 = Unbundle By Name(w1033) -> ("Feedback global"=w1064:bool)
            n542 = Empty Array?(array=w1050) -> (empty?=w1061:bool)
            n543 = property on="autodetect" class="Bool (strict)"("Value"=FALSE ("autodetect")) -> ()  [unwired: 2 in, 2 out]
            n544 = Equal To 0?(x=w1063) -> (x = 0?=w1062:bool)
            n545 = Equal To 0?(x=w1059) -> (x = 0?=w1058:bool)
            n546 = Or(x=w1062, y=w1061) -> (x .or. y?=w1060:bool)
            n547 = Or(x=w1058, y=w1057) -> (x .or. y?=w1056:bool)
            n548 = case shown="True" w1064 {
              tunnel: w1060 -> [_ w1149]
              tunnel: w1050 -> [_ w1148]
              tunnel: w1056 -> [_ w1146]
              tunnel: w1049 -> [_ w1145]
              tunnel: w1052 -> [w1142 w1144]
              tunnel: [w1142 w1143] -> w1065
              frame False {
              }
              frame True {
                n549 = case shown="False" w1149 {
                  tunnel: w1148 -> [w1164 _]
                  tunnel: w1144 -> [w1160 w1165]
                  tunnel: [w1158 w1165] -> w1147
                  frame False {
                    n550 = Index Array(array=w1164) -> (element=w1163:cluster{dbl, "GUIdevice 8":string})  [unwired: 1 in]
                    n551 = Unbundle By Name(w1163) -> ("GUIdevice 8"=w1162:string)
                    n552 = call <vilib>:"Build State String with Arguments__jki_lib_state_machine.vi"("Arguments (\"\")"=w1162, "State"="Move X") -> ("State with Arguments"=w1159:string)  [unwired: 4 in]
                    n553 = call <vilib>:"Add State(s) to Queue__jki_lib_state_machine.vi"("State(s) in (\"\")"=w1160, "State(s) at Back (\"\")"=w1159) -> ("States Out"=w1158:string)  [unwired: 13 in]
                  }
                  frame True {
                  }
                }
                n554 = case shown="False" w1146 {
                  tunnel: w1145 -> [w1156 _]
                  tunnel: w1147 -> [w1152 w1157]
                  tunnel: [w1150 w1157] -> w1143
                  frame False {
                    n555 = Index Array(array=w1156) -> (element=w1155:cluster{dbl, "GUIdevice 8":string})  [unwired: 1 in]
                    n556 = Unbundle By Name(w1155) -> ("GUIdevice 8"=w1154:string)
                    n557 = call <vilib>:"Build State String with Arguments__jki_lib_state_machine.vi"("Arguments (\"\")"=w1154, "State"="Move Y") -> ("State with Arguments"=w1151:string)  [unwired: 4 in]
                    n558 = call <vilib>:"Add State(s) to Queue__jki_lib_state_machine.vi"("State(s) in (\"\")"=w1152, "State(s) at Back (\"\")"=w1151) -> ("States Out"=w1150:string)  [unwired: 13 in]
                  }
                  frame True {
                  }
                }
              }
            }
            n559 = call <vilib>:"Add State(s) to Queue__jki_lib_state_machine.vi"("State(s) in (\"\")"=w1052, "State(s) at Back (\"\")"=w1065) -> ("States Out"=w1067:string)  [unwired: 13 in]
          }
          frame "Move X" {
            # "Your code here.\n(You can make a copy of, or modify, this frame)"
            n560 = Unbundle By Name(w1185) -> ("Offset X"=w1184:dbl[][])
            n561 = call-poly <userlib>:"Filter 1D Array__ogtk.vi"("items to filter"=w1167, "array"=w1189) -> ("filtered item indices"=w1173:i32[])  [unwired: 4 in, 1 out]
            n562 = Unbundle By Name(w1185) -> ("active axis refs 2"=w1188:T11, "move properties"=w1172:T2[])
            n563 = for {
              tunnel: w1173 -> [w1194] mode=indexing
              tunnel: w1172 -> [w1198]
              shift-right: [w1193] -> w1170
              shift-left: i32[] [] ("filtered item indices") -> [w1196]
              n564 = Index Array(array=w1198, index=w1194) -> (element=w1197:T2)
              n565 = Unbundle By Name(w1197) -> ("enable feedback"=w1195:bool)
              n566 = case shown="True" w1195 {
                tunnel: w1196 -> [w1199 w1202]
                tunnel: w1194 -> [_ w1201]
                tunnel: [w1199 w1200] -> w1193
                frame False {
                }
                frame True {
                  n567 = Build Array (concatenate)(w1202, w1201) -> (w1200:i32[])
                }
              }
            }
            n568 = Index Array(array=w1170) -> (element=w1169:i32)  [unwired: 1 in]
            n569 = Index Array(array=w1184, index (row)=w1169) -> (element=w1183:dbl[])  [unwired: 1 in]
            n570 = Reverse 1D Array(array=w1183) -> (reversed array=w1182:dbl[])
            n571 = Index Array(array=w1188, index=w1169) -> (element=w1187:cluster{"Ref X":refnum<vi>, "Ref Y":refnum<vi>})
            n572 = Index Array(array=w1182) -> (element=w1180:dbl)  [unwired: 1 in]
            n573 = Index Array(array=w1172, index=w1169) -> (element=w1186:T2)
            n574 = Unbundle By Name(w1187) -> ("Ref X"=w1176:refnum<vi>, "Ref Y"=w1175:refnum<vi>)
            n575 = call <vilib>:"Build State String with Arguments__jki_lib_state_machine.vi"("Arguments (\"\")"=w1167, "State"="Wait" ("State(s) in Front (\"\")")) -> ("State with Arguments"=w1166:string)  [unwired: 4 in]
            n576 = Unbundle By Name(w1186) -> ("Invert Direction X"=w1177:bool, "Invert Axis"=w1181:bool, "Stepsize"=w1178:dbl, "enable feedback"=w1174:bool)
            n577 = Greater Or Equal To 0?(x=w1180) -> (x >= 0?=w1179:bool)
            n578 = call <vilib>:"Add State(s) to Queue__jki_lib_state_machine.vi"("State(s) in Front (\"\")"=w1166, "State(s) in (\"\")"=w1192) -> ("States Out"=w1191:string)  [unwired: 13 in]
            n579 = case shown="True" w1174 {
              tunnel: w1181 -> [_ w1208]
              tunnel: w1179 -> [_ w1207]
              tunnel: w1178 -> [_ w1206]
              tunnel: w1177 -> [_ w1205]
              tunnel: w1176 -> [_ w1204]
              tunnel: w1175 -> [_ w1203]
              frame False {
              }
              frame True {
                n580 = case shown="False" w1207 {
                  tunnel: w1205 -> [w1216 w1238]
                  tunnel: w1206 -> [w1214 w1236]
                  tunnel: w1208 -> [w1213 w1235]
                  tunnel: w1208 -> [w1212 w1234]
                  tunnel: w1204 -> [w1210 w1232]
                  tunnel: w1203 -> [w1209 w1231]
                  frame True {
                    n581 = case shown="False" w1213 {
                      tunnel: [w1227 w1229] -> w1215
                      tunnel: w1210 -> [w1228 _]
                      tunnel: w1209 -> [_ w1230]
                      frame False {
                        n582 = property class="DigNum (strict)"(reference=w1228) -> ("Value"=w1227:dbl)  [unwired: 1 in, 2 out]
                      }
                      frame True {
                        n583 = property class="DigNum (strict)"(reference=w1230) -> ("Value"=w1229:dbl)  [unwired: 1 in, 2 out]
                      }
                    }
                    n584 = case shown="False" w1216 {
                      tunnel: w1215 -> [w1223 w1226]
                      tunnel: w1214 -> [w1222 w1225]
                      tunnel: [w1221 w1224] -> w1211
                      frame False {
                        n585 = Add(x=w1223, y=w1222) -> (x+y=w1221:dbl)
                      }
                      frame True {
                        n586 = Subtract(x=w1226, y=w1225) -> (x-y=w1224:dbl)
                      }
                    }
                    n587 = case shown="False" w1212 {
                      tunnel: w1211 -> [w1217 w1219]
                      tunnel: w1210 -> [w1218 _]
                      tunnel: w1209 -> [_ w1220]
                      frame False {
                        n588 = property class="DigNum (strict)"(reference=w1218, "Val(Sgnl)"=w1217) -> ()  [unwired: 1 in, 2 out]
                      }
                      frame True {
                        n589 = property class="DigNum (strict)"(reference=w1220, "Val(Sgnl)"=w1219) -> ()  [unwired: 1 in, 2 out]
                      }
                    }
                  }
                  frame False {
                    n590 = case shown="False" w1235 {
                      tunnel: [w1249 w1251] -> w1237
                      tunnel: w1232 -> [w1250 _]
                      tunnel: w1231 -> [_ w1252]
                      frame False {
                        n591 = property class="DigNum (strict)"(reference=w1250) -> ("Value"=w1249:dbl)  [unwired: 1 in, 2 out]
                      }
                      frame True {
                        n592 = property class="DigNum (strict)"(reference=w1252) -> ("Value"=w1251:dbl)  [unwired: 1 in, 2 out]
                      }
                    }
                    n593 = case shown="False" w1238 {
                      tunnel: w1237 -> [w1245 w1248]
                      tunnel: w1236 -> [w1244 w1247]
                      tunnel: [w1243 w1246] -> w1233
                      frame False {
                        n594 = Subtract(x=w1245, y=w1244) -> (x-y=w1243:dbl)
                      }
                      frame True {
                        n595 = Add(x=w1248, y=w1247) -> (x+y=w1246:dbl)
                      }
                    }
                    n596 = case shown="False" w1234 {
                      tunnel: w1233 -> [w1239 w1241]
                      tunnel: w1232 -> [w1240 _]
                      tunnel: w1231 -> [_ w1242]
                      frame False {
                        n597 = property class="DigNum (strict)"(reference=w1240, "Val(Sgnl)"=w1239) -> ()  [unwired: 1 in, 2 out]
                      }
                      frame True {
                        n598 = property class="DigNum (strict)"(reference=w1242, "Val(Sgnl)"=w1241) -> ()  [unwired: 1 in, 2 out]
                      }
                    }
                  }
                }
              }
            }
            "Moving X" <- w1167
          }
          frame "ManMove X" {
            # "Your code here.\n(You can make a copy of, or modify, this frame)"
            n599 = Equal?(x=w1258, y="Right") -> (x = y?=w1259:bool)
            n600 = Unbundle By Name(w1268) -> ("move properties"=w1263:T2[], "active ccd"=w1256:i32, "active man refs"=w1261:cluster{"Ref X":refnum<vi>, "Ref Y":refnum<vi>}, "active cams"=w1257:string[])
            n601 = Index Array(array=w1257, index=w1256) -> (element=w1254:string)
            n602 = Index Array(array=w1263, index=w1256) -> (element=w1269:T2)
            n603 = Unbundle By Name(w1261) -> ("Ref X"=w1265:refnum<vi>, "Ref Y"=w1264:refnum<vi>)
            n604 = Unbundle By Name(w1269) -> ("Invert Direction X"=w1266:bool, "Invert Axis"=w1267:bool)
            n605 = call <vilib>:"Build State String with Arguments__jki_lib_state_machine.vi"("Arguments (\"\")"=w1254, "State"="Wait" ("State(s) in Front (\"\")")) -> ("State with Arguments"=w1253:string)  [unwired: 4 in]
            n606 = call <vilib>:"Add State(s) to Queue__jki_lib_state_machine.vi"("State(s) in Front (\"\")"=w1253, "State(s) in (\"\")"=w1272) -> ("States Out"=w1271:string)  [unwired: 13 in]
            n607 = case shown="False" w1259 {
              tunnel: w1266 -> [w1280 w1302]
              tunnel: "StepSize" -> [w1278 w1300]
              tunnel: w1267 -> [w1277 w1299]
              tunnel: w1267 -> [w1276 w1298]
              tunnel: w1265 -> [w1274 w1296]
              tunnel: w1264 -> [w1273 w1295]
              frame True {
                n608 = case shown="False" w1277 {
                  tunnel: [w1291 w1293] -> w1279
                  tunnel: w1274 -> [w1292 _]
                  tunnel: w1273 -> [_ w1294]
                  frame False {
                    n609 = property class="DigNum (strict)"(reference=w1292) -> ("Value"=w1291:dbl)  [unwired: 1 in, 2 out]
                  }
                  frame True {
                    n610 = property class="DigNum (strict)"(reference=w1294) -> ("Value"=w1293:dbl)  [unwired: 1 in, 2 out]
                  }
                }
                n611 = case shown="False" w1280 {
                  tunnel: w1279 -> [w1287 w1290]
                  tunnel: w1278 -> [w1286 w1289]
                  tunnel: [w1285 w1288] -> w1275
                  frame False {
                    n612 = Add(x=w1287, y=w1286) -> (x+y=w1285:dbl)
                  }
                  frame True {
                    n613 = Subtract(x=w1290, y=w1289) -> (x-y=w1288:dbl)
                  }
                }
                n614 = case shown="False" w1276 {
                  tunnel: w1275 -> [w1281 w1283]
                  tunnel: w1274 -> [w1282 _]
                  tunnel: w1273 -> [_ w1284]
                  frame False {
                    n615 = property class="DigNum (strict)"(reference=w1282, "Val(Sgnl)"=w1281) -> ()  [unwired: 1 in, 2 out]
                  }
                  frame True {
                    n616 = property class="DigNum (strict)"(reference=w1284, "Val(Sgnl)"=w1283) -> ()  [unwired: 1 in, 2 out]
                  }
                }
              }
              frame False {
                n617 = case shown="True" w1299 {
                  tunnel: [w1313 w1315] -> w1301
                  tunnel: w1296 -> [w1314 _]
                  tunnel: w1295 -> [_ w1316]
                  frame False {
                    n618 = property class="DigNum (strict)"(reference=w1314) -> ("Value"=w1313:dbl)  [unwired: 1 in, 2 out]
                  }
                  frame True {
                    n619 = property class="DigNum (strict)"(reference=w1316) -> ("Value"=w1315:dbl)  [unwired: 1 in, 2 out]
                  }
                }
                n620 = case shown="True" w1302 {
                  tunnel: w1301 -> [w1309 w1312]
                  tunnel: w1300 -> [w1308 w1311]
                  tunnel: [w1307 w1310] -> w1297
                  frame False {
                    n621 = Subtract(x=w1309, y=w1308) -> (x-y=w1307:dbl)
                  }
                  frame True {
                    n622 = Add(x=w1312, y=w1311) -> (x+y=w1310:dbl)
                  }
                }
                n623 = case shown="False" w1298 {
                  tunnel: w1297 -> [w1303 w1305]
                  tunnel: w1296 -> [w1304 _]
                  tunnel: w1295 -> [_ w1306]
                  frame False {
                    n624 = property class="DigNum (strict)"(reference=w1304, "Val(Sgnl)"=w1303) -> ()  [unwired: 1 in, 2 out]
                  }
                  frame True {
                    n625 = property class="DigNum (strict)"(reference=w1306, "Val(Sgnl)"=w1305) -> ()  [unwired: 1 in, 2 out]
                  }
                }
              }
            }
          }
          frame "ManMove Y" {
            # "Your code here.\n(You can make a copy of, or modify, this frame)"
            n626 = Equal?(x=w1322, y="Down") -> (x = y?=w1326:bool)
            n627 = Unbundle By Name(w1332) -> ("active cams"=w1321:string[], "move properties"=w1331:T2[], "active ccd"=w1320:i32, "active man refs"=w1330:cluster{"Ref X":refnum<vi>, "Ref Y":refnum<vi>})
            n628 = Index Array(array=w1321, index=w1320) -> (element=w1318:string)
            n629 = property on="StepSize" class="DigNum (strict)"() -> ("Value"=w1323:i16)  [unwired: 2 in, 2 out]
            n630 = Index Array(array=w1331, index=w1320) -> (element=w1333:T2)
            n631 = Unbundle By Name(w1330) -> ("Ref Y"=w1325:refnum<vi>, "Ref X"=w1324:refnum<vi>)
            n632 = Unbundle By Name(w1333) -> ("Invert Direction Y"=w1328:bool, "Invert Axis"=w1327:bool)
            n633 = call <vilib>:"Build State String with Arguments__jki_lib_state_machine.vi"("Arguments (\"\")"=w1318, "State"="Wait" ("State(s) in Front (\"\")")) -> ("State with Arguments"=w1317:string)  [unwired: 4 in]
            n634 = call <vilib>:"Add State(s) to Queue__jki_lib_state_machine.vi"("State(s) in Front (\"\")"=w1317, "State(s) in (\"\")"=w1336) -> ("States Out"=w1335:string)  [unwired: 13 in]
            n635 = case shown="True" w1326 {
              tunnel: w1328 -> [w1344 w1366]
              tunnel: w1323 -> [w1342 w1364]
              tunnel: w1327 -> [w1341 w1363]
              tunnel: w1327 -> [w1340 w1362]
              tunnel: w1325 -> [w1338 w1360]
              tunnel: w1324 -> [w1337 w1359]
              frame True {
                n636 = case shown="False" w1341 {
                  tunnel: [w1355 w1357] -> w1343
                  tunnel: w1338 -> [w1356 _]
                  tunnel: w1337 -> [_ w1358]
                  frame False {
                    n637 = property class="DigNum (strict)"(reference=w1356) -> ("Value"=w1355:dbl)  [unwired: 1 in, 2 out]
                  }
                  frame True {
                    n638 = property class="DigNum (strict)"(reference=w1358) -> ("Value"=w1357:dbl)  [unwired: 1 in, 2 out]
                  }
                }
                n639 = case shown="False" w1344 {
                  tunnel: w1343 -> [w1351 w1354]
                  tunnel: w1342 -> [w1350 w1353]
                  tunnel: [w1349 w1352] -> w1339
                  frame False {
                    n640 = Add(x=w1351, y=w1350) -> (x+y=w1349:dbl)
                  }
                  frame True {
                    n641 = Subtract(x=w1354, y=w1353) -> (x-y=w1352:dbl)
                  }
                }
                n642 = case shown="False" w1340 {
                  tunnel: w1339 -> [w1345 w1347]
                  tunnel: w1338 -> [w1346 _]
                  tunnel: w1337 -> [_ w1348]
                  frame False {
                    n643 = property class="DigNum (strict)"(reference=w1346, "Val(Sgnl)"=w1345) -> ()  [unwired: 1 in, 2 out]
                  }
                  frame True {
                    n644 = property class="DigNum (strict)"(reference=w1348, "Val(Sgnl)"=w1347) -> ()  [unwired: 1 in, 2 out]
                  }
                }
              }
              frame False {
                n645 = case shown="False" w1363 {
                  tunnel: [w1377 w1379] -> w1365
                  tunnel: w1360 -> [w1378 _]
                  tunnel: w1359 -> [_ w1380]
                  frame False {
                    n646 = property class="DigNum (strict)"(reference=w1378) -> ("Value"=w1377:dbl)  [unwired: 1 in, 2 out]
                  }
                  frame True {
                    n647 = property class="DigNum (strict)"(reference=w1380) -> ("Value"=w1379:dbl)  [unwired: 1 in, 2 out]
                  }
                }
                n648 = case shown="False" w1366 {
                  tunnel: w1365 -> [w1373 w1376]
                  tunnel: w1364 -> [w1372 w1375]
                  tunnel: [w1371 w1374] -> w1361
                  frame False {
                    n649 = Subtract(x=w1373, y=w1372) -> (x-y=w1371:dbl)
                  }
                  frame True {
                    n650 = Add(x=w1376, y=w1375) -> (x+y=w1374:dbl)
                  }
                }
                n651 = case shown="False" w1362 {
                  tunnel: w1361 -> [w1367 w1369]
                  tunnel: w1360 -> [w1368 _]
                  tunnel: w1359 -> [_ w1370]
                  frame False {
                    n652 = property class="DigNum (strict)"(reference=w1368, "Val(Sgnl)"=w1367) -> ()  [unwired: 1 in, 2 out]
                  }
                  frame True {
                    n653 = property class="DigNum (strict)"(reference=w1370, "Val(Sgnl)"=w1369) -> ()  [unwired: 1 in, 2 out]
                  }
                }
              }
            }
          }
          frame "Move Y" {
            # "Your code here.\n(You can make a copy of, or modify, this frame)"
            n654 = Unbundle By Name(w1400) -> ("Offset Y"=w1399:dbl[][])
            n655 = call-poly <userlib>:"Filter 1D Array__ogtk.vi"("items to filter"=w1382, "array"=w1404) -> ("filtered item indices"=w1388:i32[])  [unwired: 4 in, 1 out]
            n656 = Unbundle By Name(w1400) -> ("active axis refs 2"=w1403:T11, "move properties"=w1386:T2[])
            n657 = for {
              tunnel: w1388 -> [w1409] mode=indexing
              tunnel: w1386 -> [w1413]
              shift-right: [w1408] -> w1387
              shift-left: i32[] [] ("filtered item indices") -> [w1411]
              n658 = Index Array(array=w1413, index=w1409) -> (element=w1412:T2)
              n659 = Unbundle By Name(w1412) -> ("enable feedback"=w1410:bool)
              n660 = case shown="True" w1410 {
                tunnel: w1411 -> [w1414 w1417]
                tunnel: w1409 -> [_ w1416]
                tunnel: [w1414 w1415] -> w1408
                frame False {
                }
                frame True {
                  n661 = Build Array (concatenate)(w1417, w1416) -> (w1415:i32[])
                }
              }
            }
            n662 = Index Array(array=w1387) -> (element=w1384:i32)  [unwired: 1 in]
            n663 = Index Array(array=w1399, index (row)=w1384) -> (element=w1398:dbl[])  [unwired: 1 in]
            n664 = Reverse 1D Array(array=w1398) -> (reversed array=w1397:dbl[])
            n665 = Index Array(array=w1403, index=w1384) -> (element=w1402:cluster{"Ref X":refnum<vi>, "Ref Y":refnum<vi>})
            n666 = Index Array(array=w1397) -> (element=w1395:dbl)  [unwired: 1 in]
            n667 = Index Array(array=w1386, index=w1384) -> (element=w1401:T2)
            n668 = Unbundle By Name(w1402) -> ("Ref Y"=w1391:refnum<vi>, "Ref X"=w1390:refnum<vi>)
            n669 = Unbundle By Name(w1401) -> ("Invert Direction Y"=w1392:bool, "Invert Axis"=w1396:bool, "Stepsize"=w1393:dbl, "enable feedback"=w1389:bool)
            n670 = Greater Or Equal To 0?(x=w1395) -> (x >= 0?=w1394:bool)
            n671 = call <vilib>:"Build State String with Arguments__jki_lib_state_machine.vi"("Arguments (\"\")"=w1382, "State"="Wait" ("State(s) in Front (\"\")")) -> ("State with Arguments"=w1381:string)  [unwired: 4 in]
            n672 = call <vilib>:"Add State(s) to Queue__jki_lib_state_machine.vi"("State(s) in Front (\"\")"=w1381, "State(s) in (\"\")"=w1407) -> ("States Out"=w1406:string)  [unwired: 13 in]
            n673 = case shown="True" w1389 {
              tunnel: w1396 -> [_ w1423]
              tunnel: w1394 -> [_ w1422]
              tunnel: w1393 -> [_ w1421]
              tunnel: w1392 -> [_ w1420]
              tunnel: w1391 -> [_ w1419]
              tunnel: w1390 -> [_ w1418]
              frame False {
              }
              frame True {
                n674 = case shown="True" w1422 {
                  tunnel: w1420 -> [w1431 w1453]
                  tunnel: w1421 -> [w1429 w1451]
                  tunnel: w1423 -> [w1428 w1450]
                  tunnel: w1423 -> [w1427 w1449]
                  tunnel: w1419 -> [w1425 w1447]
                  tunnel: w1418 -> [w1424 w1446]
                  frame True {
                    n675 = case shown="False" w1428 {
                      tunnel: [w1442 w1444] -> w1430
                      tunnel: w1425 -> [w1443 _]
                      tunnel: w1424 -> [_ w1445]
                      frame False {
                        n676 = property class="DigNum (strict)"(reference=w1443) -> ("Value"=w1442:dbl)  [unwired: 1 in, 2 out]
                      }
                      frame True {
                        n677 = property class="DigNum (strict)"(reference=w1445) -> ("Value"=w1444:dbl)  [unwired: 1 in, 2 out]
                      }
                    }
                    n678 = case shown="False" w1431 {
                      tunnel: w1430 -> [w1438 w1441]
                      tunnel: w1429 -> [w1437 w1440]
                      tunnel: [w1436 w1439] -> w1426
                      frame False {
                        n679 = Add(x=w1438, y=w1437) -> (x+y=w1436:dbl)
                      }
                      frame True {
                        n680 = Subtract(x=w1441, y=w1440) -> (x-y=w1439:dbl)
                      }
                    }
                    n681 = case shown="False" w1427 {
                      tunnel: w1426 -> [w1432 w1434]
                      tunnel: w1425 -> [w1433 _]
                      tunnel: w1424 -> [_ w1435]
                      frame False {
                        n682 = property class="DigNum (strict)"(reference=w1433, "Val(Sgnl)"=w1432) -> ()  [unwired: 1 in, 2 out]
                      }
                      frame True {
                        n683 = property class="DigNum (strict)"(reference=w1435, "Val(Sgnl)"=w1434) -> ()  [unwired: 1 in, 2 out]
                      }
                    }
                  }
                  frame False {
                    n684 = case shown="False" w1450 {
                      tunnel: [w1464 w1466] -> w1452
                      tunnel: w1447 -> [w1465 _]
                      tunnel: w1446 -> [_ w1467]
                      frame False {
                        n685 = property class="DigNum (strict)"(reference=w1465) -> ("Value"=w1464:dbl)  [unwired: 1 in, 2 out]
                      }
                      frame True {
                        n686 = property class="DigNum (strict)"(reference=w1467) -> ("Value"=w1466:dbl)  [unwired: 1 in, 2 out]
                      }
                    }
                    n687 = case shown="False" w1453 {
                      tunnel: w1452 -> [w1460 w1463]
                      tunnel: w1451 -> [w1459 w1462]
                      tunnel: [w1458 w1461] -> w1448
                      frame False {
                        n688 = Subtract(x=w1460, y=w1459) -> (x-y=w1458:dbl)
                      }
                      frame True {
                        n689 = Add(x=w1463, y=w1462) -> (x+y=w1461:dbl)
                      }
                    }
                    n690 = case shown="False" w1449 {
                      tunnel: w1448 -> [w1454 w1456]
                      tunnel: w1447 -> [w1455 _]
                      tunnel: w1446 -> [_ w1457]
                      frame False {
                        n691 = property class="DigNum (strict)"(reference=w1455, "Val(Sgnl)"=w1454) -> ()  [unwired: 1 in, 2 out]
                      }
                      frame True {
                        n692 = property class="DigNum (strict)"(reference=w1457, "Val(Sgnl)"=w1456) -> ()  [unwired: 1 in, 2 out]
                      }
                    }
                  }
                }
              }
            }
            "Moving Y" <- w1382
          }
          frame "Wait" {
            # "Your code here.\n(You can make a copy of, or modify, this frame)"
            n693 = flat-sequence {
              tunnel: T19."Disabled and Grayed Out" ("Disabled") -> [w1484]
              tunnel: w1474 -> [w1493]
              tunnel: w1473 -> [w1492]
              tunnel: [w1491] -> w1472
              tunnel: w1471 -> [w1490]
              tunnel: w1470 -> [w1489]
              tunnel: T19."Enabled" ("Disabled") -> [w1503]
              frame #0 {
                n694 = property on="Right" class="Bool (strict)"("DisabledEnum"=w1484) -> ()  [unwired: 2 in, 2 out]
                n695 = property on="Up" class="Bool (strict)"("DisabledEnum"=w1484) -> ()  [unwired: 2 in, 2 out]
                n696 = property on="Left" class="Bool (strict)"("DisabledEnum"=w1484) -> ()  [unwired: 2 in, 2 out]
                n697 = property on="Down" class="Bool (strict)"("DisabledEnum"=w1484) -> ()  [unwired: 2 in, 2 out]
                n698 = property on="StepSize" class="DigNum (strict)"("DisabledEnum"=w1484) -> ()  [unwired: 2 in, 2 out]
              }
              frame #1 {
                n699 = Wait (ms)(milliseconds to wait=u32 800) -> ()  [unwired: 1 out]
              }
              frame #2 {
                n700 = property on="Moving Y" class="Str"("Value"="") -> ()  [unwired: 2 in, 2 out]
                n701 = property on="Moving X" class="Str"("Value"="") -> ()  [unwired: 2 in, 2 out]
              }
              frame #3 {
                n702 = Equal?(x=w1489, y=w1490) -> (x = y?=w1488:bool)
                n703 = case shown="True" w1488 {
                  tunnel: w1493 -> [_ w1500]
                  tunnel: w1492 -> [w1494 w1497]
                  tunnel: [w1494 w1495] -> w1491
                  frame False {
                  }
                  frame True {
                    n704 = Unbundle By Name(w1500) -> ("Ref X"=w1499:refnum<vi>, "Ref Y"=w1498:refnum<vi>)
                    n705 = property class="DigNum (strict)"(reference=w1499, error in=w1497) -> (error out=w1496:errorcluster, "Value"=w1502:dbl)  [unwired: 1 out]
                    n706 = property class="DigNum (strict)"(reference=w1498, error in=w1496) -> (error out=w1495:errorcluster, "Value"=w1501:dbl)  [unwired: 1 out]
                    n707 = property on="Position 1" class="DigNum (strict)"("Value"=w1502) -> ()  [unwired: 2 in, 2 out]
                    n708 = property on="Position 2" class="DigNum (strict)"("Value"=w1501) -> ()  [unwired: 2 in, 2 out]
                  }
                }
              }
              frame #4 {
                n709 = property on="Right" class="Bool (strict)"("DisabledEnum"=w1503) -> ()  [unwired: 2 in, 2 out]
                n710 = property on="Up" class="Bool (strict)"("DisabledEnum"=w1503) -> ()  [unwired: 2 in, 2 out]
                n711 = property on="Left" class="Bool (strict)"("DisabledEnum"=w1503) -> ()  [unwired: 2 in, 2 out]
                n712 = property on="Down" class="Bool (strict)"("DisabledEnum"=w1503) -> ()  [unwired: 2 in, 2 out]
                n713 = property on="StepSize" class="DigNum (strict)"("DisabledEnum"=w1503) -> ()  [unwired: 2 in, 2 out]
              }
            }
            n714 = call-poly <userlib>:"Filter 1D Array__ogtk.vi"("items to filter"=w1477, "array"=w1478) -> ("filtered item indices"=w1476:i32[])  [unwired: 4 in, 1 out]
            n715 = Index Array(array=w1476) -> (element=w1471:i32)  [unwired: 1 in]
            n716 = Unbundle By Name(w1479) -> ("active axis refs 2"=w1475:T11, "active ccd"=w1470:i32)
            n717 = Index Array(array=w1475, index=w1471) -> (element=w1474:cluster{"Ref X":refnum<vi>, "Ref Y":refnum<vi>})
            n718 = call <vilib>:"Add State(s) to Queue__jki_lib_state_machine.vi"("State(s) in (\"\")"=w1483) -> ("States Out"=w1482:string)  [unwired: 14 in]
            n719 = local read "Mean Centroid X"() -> (w1480:dbl[][])
            n720 = Bundle By Name(cluster=w1479, "Mean Centroid X"=w1480, "Mean Centroid Y"=w1480) -> (w1481:T36)
          }
          frame "---------------Statistics--------------" {
            # "Template Separator\n(You can make a copy of, or modify, this frame)"
            n721 = call <vilib>:"Add State(s) to Queue__jki_lib_state_machine.vi"("State(s) in (\"\")"=w1507) -> ("States Out"=w1506:string)  [unwired: 14 in]
          }
          frame "Save Stats" {
            # "Your code here.\n(You can make a copy of, or modify, this frame)"
            n722 = property on="CCD 1" class="XYGraph (strict)"() -> ("Value"=w1518:cluster{timestamp[], dbl[]}[])  [unwired: 2 in, 2 out]
            n723 = property on="CCD 2" class="XYGraph (strict)"() -> ("Value"=w1517:cluster{timestamp[], dbl[]}[])  [unwired: 2 in, 2 out]
            n724 = property on="CCD 3" class="XYGraph (strict)"() -> ("Value"=w1516:cluster{timestamp[], dbl[]}[])  [unwired: 2 in, 2 out]
            n725 = property on="CCD 4" class="XYGraph (strict)"() -> ("Value"=w1515:cluster{timestamp[], dbl[]}[])  [unwired: 2 in, 2 out]
            n726 = property on="CCD 5" class="XYGraph (strict)"() -> ("Value"=w1514:cluster{timestamp[], dbl[]}[])  [unwired: 2 in, 2 out]
            n727 = property on="CCD 6" class="XYGraph (strict)"() -> ("Value"=w1513:cluster{timestamp[], dbl[]}[])  [unwired: 2 in, 2 out]
            n728 = property on="CCD 7" class="XYGraph (strict)"() -> ("Value"=w1512:cluster{timestamp[], dbl[]}[])  [unwired: 2 in, 2 out]
            n729 = property on="CCD 8" class="XYGraph (strict)"() -> ("Value"=w1511:cluster{timestamp[], dbl[]}[])  [unwired: 2 in, 2 out]
            n730 = Build Array(w1518, w1517, w1516, w1515, w1514, w1513, w1512, w1511) -> (w1510:cluster{timestamp[], dbl[]}[][])
            n731 = disable-structure shown="Disabled" {
              disable-tunnel: w1522 -> [w1526 _]
              disable-tunnel: [w1525 _] -> w1521
              disable-tunnel: w1510 -> [w1524 _]
              disable-tunnel: w1509 -> [w1523 _]
              frame Disabled {
                n732 = for {
                  tunnel: w1524 -> [w1529] mode=indexing
                  tunnel: w1523 -> [w1528] mode=indexing
                  n733 = Empty String/Path?(string/path=w1528) -> (empty?=w1527:bool)
                  n734 = case shown="False" w1527 {
                    tunnel: w1529 -> [w1535 _]
                    tunnel: w1528 -> [w1533 _]
                    frame False {
                      n735 = Index Array(array=w1535, index #1=0 ("index"), index #2=1 ("index"), index #3=2 ("index"), index #4=3 ("index")) -> (element #1=w1570:cluster{timestamp[], dbl[]}, element #2=w1564:cluster{timestamp[], dbl[]}, element #3=w1563:cluster{timestamp[], dbl[]}, element #4=w1562:cluster{timestamp[], dbl[]})  [unwired: 1 in, 1 out]
                      n736 = Concatenate Strings(w1533, ".dat" ("string")) -> (w1531:string)
                      n737 = Unbundle(w1570) -> (w1569:timestamp[], w1547:dbl[])
                      n738 = Unbundle(w1564) -> (w1538:dbl[])  [unwired: 1 out]
                      n739 = Unbundle(w1563) -> (w1537:dbl[])  [unwired: 1 out]
                      n740 = Unbundle(w1562) -> (w1536:dbl[])  [unwired: 1 out]
                      n741 = Build Path(base path="save path", name or relative path=w1531) -> (appended path=w1530:path)
                      n742 = for {
                        tunnel: w1569 -> [w1572] mode=indexing
                        tunnel: [w1571] -> w1545 mode=indexing
                        n743 = Format Date/Time String(time format string (%c)="%Y%m%d%H%M%S", seconds (now)=w1572) -> (date/time string=w1571:string)  [unwired: 1 in]
                      }
                      n744 = Array Size(array=w1547) -> (size(s)=w1548:i32)
                      n745 = Number To Fractional String(number=w1547) -> (F-format string=w1544:string[])  [unwired: 3 in]
                      n746 = Number To Fractional String(number=w1538) -> (F-format string=w1541:string[])  [unwired: 3 in]
                      n747 = Number To Fractional String(number=w1537) -> (F-format string=w1540:string[])  [unwired: 3 in]
                      n748 = Number To Fractional String(number=w1536) -> (F-format string=w1539:string[])  [unwired: 3 in]
                      n749 = Initialize Array("", w1548, 5 ("dimension size")) -> (w1546:string[][])
                      n750 = Insert Into Array(array=w1546, index (col)=0 ("disabled index (col)"), new element=w1545) -> (w1556:string[][])  [unwired: 1 in]
                      n751 = Insert Into Array(array=w1556, index (col)=1 ("disabled index (col)"), new element=w1544) -> (w1555:string[][])  [unwired: 1 in]
                      n752 = Insert Into Array(array=w1555, index (col)=2 ("disabled index (col)"), new element=w1541) -> (w1559:string[][])  [unwired: 1 in]
                      n753 = Insert Into Array(array=w1559, index (col)=3 ("disabled index (col)"), new element=w1540) -> (w1560:string[][])  [unwired: 1 in]
                      n754 = Insert Into Array(array=w1560, index (col)=4 ("disabled index (col)"), new element=w1539) -> (w1561:string[][])  [unwired: 1 in]
                      n755 = Insert Into Array(array=w1561, index (row)=0, new element=string[] ["time", "Centroid X", "Centroid Y", "Motor Axis 1", "Motor Axis 2"] ("new element/subarray 2")) -> (w1543:string[][])  [unwired: 1 in]
                      n756 = call-poly <vilib>:"Write To Spreadsheet File.vi"("2D data"=w1543, "file path (dialog if empty)"=w1530) -> ()  [unwired: 6 in, 1 out]
                    }
                    frame True {
                    }
                  }
                }
                n757 = call <vilib>:"Add State(s) to Queue__jki_lib_state_machine.vi"("State(s) in (\"\")"=w1526) -> ("States Out"=w1525:string)  [unwired: 14 in]
              }
              frame Enabled {
              }
            }
            n758 = property on="Save Stats" class="Bool (strict)"("Value"=FALSE ("Save Stats")) -> ()  [unwired: 2 in, 2 out]
          }
          frame "tdms" {
            w1583 = 21600.0 ("new tdms")
            # "Your code here.\n(You can make a copy of, or modify, this frame)"
            n759 = Unbundle By Name(w1592) -> ("active cams"=w1576:string[], "Data Value Reference out"=w1591:refnum<k34>, "Offset X"=w1590:dbl[][], "Offset Y"=w1589:dbl[][], "active axis refs 2"=w1588:T11)
            n760 = for {
              tunnel: w1590 -> [w1639]
              tunnel: w1589 -> [w1638]
              tunnel: w1576 -> [w1602] mode=indexing
              tunnel: w1591 -> [w1603]
              tunnel: w1588 -> [w1624]
              tunnel: w1594 -> [w1608]
              tunnel: [w1606] -> w1593
              i -> [w1625]
              n761 = Index Array(array=w1639, index (row)=w1625) -> (element=w1637:dbl[])  [unwired: 1 in]
              n762 = Index Array(array=w1638, index (row)=w1625) -> (element=w1636:dbl[])  [unwired: 1 in]
              n763 = Index Array(array=w1624, index=w1625) -> (element=w1623:cluster{"Ref X":refnum<vi>, "Ref Y":refnum<vi>})
              n764 = Reverse 1D Array(array=w1636) -> (reversed array=w1634:dbl[])
              n765 = Reverse 1D Array(array=w1637) -> (reversed array=w1635:dbl[])
              n766 = Unbundle By Name(w1623) -> ("Ref X"=w1622:refnum<vi>, "Ref Y"=w1621:refnum<vi>)
              n767 = Index Array(array=w1635) -> (element=w1633:dbl)  [unwired: 1 in]
              n768 = Index Array(array=w1634) -> (element=w1632:dbl)  [unwired: 1 in]
              n769 = property class="DigNum (strict)"(reference=w1622, error in=w1608) -> (error out=w1607:errorcluster, "Value"=w1616:dbl)  [unwired: 1 out]
              n770 = Build Array(w1633) -> (w1605:dbl[])
              n771 = Build Array(w1632) -> (w1627:dbl[])
              n772 = Get Date/Time In Seconds() -> (seconds since 1Jan1904=w1604:timestamp)
              n773 = Build Array(w1604) -> (w1600:timestamp[])
              n774 = property class="DigNum (strict)"(reference=w1621, error in=w1607) -> (error out=w1598:errorcluster, "Value"=w1610:dbl)  [unwired: 1 out]
              n775 = Build Array(w1616) -> (w1615:dbl[])
              n776 = TDMS Write(0:w1603, 5:w1602, 7:"time", 9:w1600, 11:w1598) -> (4:w1599:refnum<k34>, 15:w1597:errorcluster)  [unwired: 1 in, 2 out]
              n777 = Build Array(w1610) -> (w1609:dbl[])
              n778 = TDMS Write(0:w1599, 5:w1602, 7:"centroid X", 9:w1605, 11:w1597) -> (4:w1630:refnum<k34>, 6:w1629:string, 15:w1628:errorcluster)  [unwired: 1 in, 1 out]
              n779 = TDMS Write(0:w1630, 5:w1629, 7:"centroid Y", 9:w1627, 11:w1628) -> (4:w1619:refnum<k34>, 6:w1618:string, 15:w1620:errorcluster)  [unwired: 1 in, 1 out]
              n780 = TDMS Write(0:w1619, 5:w1618, 7:"Motor Axis 1", 9:w1615, 11:w1620) -> (4:w1614:refnum<k34>, 6:w1613:string, 15:w1611:errorcluster)  [unwired: 1 in, 1 out]
              n781 = TDMS Write(0:w1614, 5:w1613, 7:"Motor Axis 2", 9:w1609, 11:w1611) -> (15:w1606:errorcluster)  [unwired: 1 in, 3 out]
            }
            n782 = property on="millisecond timer value" class="DigNum (strict)"() -> ("Value"=w1575:u32)  [unwired: 2 in, 2 out]
            n783 = Tick Count (ms)() -> (millisecond timer value=w1574:u32)
            n784 = Unbundle By Name(w1592) -> ()  [unwired: 1 out]
            n785 = Subtract(x=w1574, y=w1575) -> (x-y=w1578:u32)
            n786 = Divide(x=w1578, y=u32 1000) -> (x/y=w1580:dbl)
            n787 = Quotient & Remainder(x=w1580, y=w1583) -> (x-y*floor(x/y)=w1581:dbl)  [unwired: 1 out]
            n788 = Subtract(x=w1583, y=20.0) -> (x-y=w1585:dbl)
            n789 = Greater?(x=w1581, y=w1585) -> (0:w1582:bool)
            n790 = Select(t="newtdms", s=w1582, f="") -> (s? t:f=w1577:string)
            n791 = call <vilib>:"Add State(s) to Queue__jki_lib_state_machine.vi"("State(s) in (\"\")"=w1596, "State(s) at Back (\"\")"=w1577) -> ("States Out"=w1595:string)  [unwired: 13 in]
          }
          frame "Reset History" {
            # "Your code here.\n(You can make a copy of, or modify, this frame)"
            n792 = for {
              N: 1 -> [_]
              shift-right: [w1649] -> w1641
              shift-left: timestamp[][] [] ("Time") -> [w1651]
              n793 = for {
                N: 12 -> [_]
                tunnel: w1651 -> [w1654] mode=indexing
                tunnel: [w1652] -> w1649 mode=indexing
                n794 = Get Date/Time In Seconds() -> (seconds since 1Jan1904=w1653:timestamp)
                n795 = Build Array (concatenate)(w1654, w1653) -> (w1652:timestamp[])
              }
            }
            n796 = local read "Offset X"() -> (w1640:dbl[][])
            n797 = Bundle By Name(cluster=w1645, "Offset X"=w1640, "Offset Y"=w1640, "Time"=w1641, "Motor X"=w1640) -> (w1644:T36)
            n798 = call <vilib>:"Add State(s) to Queue__jki_lib_state_machine.vi"("State(s) in (\"\")"=w1648) -> ("States Out"=w1647:string)  [unwired: 14 in]
          }
          frame "New Category: 2" {
            # "Your code here.\n(You can make a copy of, or modify, this frame)"
            n799 = call <vilib>:"Add State(s) to Queue__jki_lib_state_machine.vi"("State(s) in (\"\")"=w1658) -> ("States Out"=w1657:string)  [unwired: 14 in]
          }
          frame "stats" {
            # "Your code here.\n(You can make a copy of, or modify, this frame)"
            n800 = Unbundle By Name(w1672) -> ("Offset X"=w1670:dbl[][], "Offset Y"=w1669:dbl[][], "Time"=w1668:timestamp[][], "Motor X"=w1667:dbl[][], "Motor Y"=w1666:dbl[][], "Data Value Reference out"=w1662:refnum<k34>)
            n801 = TDMS List Contents(4:w1661, 7:w1662) -> (0:w1665:errorcluster, 2:w1663:string[], 3:w1664:refnum<k34>)  [unwired: 1 in, 1 out]
            n802 = for {
              tunnel: w1665 -> [w1717]
              tunnel: [w1703] -> w1659 mode=indexing
              tunnel: [w1702] -> w1660
              tunnel: [w1701] -> _
              tunnel: w1664 -> [w1700]
              tunnel: w1663 -> [w1699] mode=indexing
              w1718 = dbl[] [] ("appended array")
              n803 = TDMS Read(0:w1700, 5:w1699, 7:"time", 11:w1717, 12:timestamp[] [] ("appended array")) -> (4:w1732:refnum<k34>, 6:w1728:string, 10:w1709:timestamp[], 15:w1716:errorcluster)  [unwired: 3 in, 2 out]
              n804 = TDMS Read(0:w1732, 5:w1728, 7:"centroid X", 11:w1716, 12:w1718) -> (4:w1731:refnum<k34>, 6:w1727:string, 10:w1712:dbl[], 15:w1715:errorcluster)  [unwired: 3 in, 2 out]
              n805 = TDMS Read(0:w1731, 5:w1727, 7:"centroid Y", 11:w1715, 12:w1718) -> (4:w1730:refnum<k34>, 6:w1726:string, 10:w1711:dbl[], 15:w1714:errorcluster)  [unwired: 3 in, 2 out]
              n806 = TDMS Read(0:w1730, 5:w1726, 7:"Motor Axis 1", 11:w1714, 12:w1718) -> (4:w1729:refnum<k34>, 6:w1725:string, 10:w1710:dbl[], 15:w1713:errorcluster)  [unwired: 3 in, 2 out]
              n807 = TDMS Read(0:w1729, 5:w1725, 7:"Motor Axis 2", 11:w1713, 12:w1718) -> (4:w1701:refnum<k34>, 10:w1708:dbl[], 15:w1702:errorcluster)  [unwired: 3 in, 3 out]
              n808 = Bundle("appended array"=w1709, "appended array"=w1712) -> (w1707:T38)  [unwired: 1 in]
              n809 = Bundle("appended array"=w1709, "appended array"=w1711) -> (w1706:T38)  [unwired: 1 in]
              n810 = Bundle("appended array"=w1709, "appended array"=w1710) -> (w1705:T38)  [unwired: 1 in]
              n811 = Bundle("appended array"=w1709, "appended array"=w1708) -> (w1704:T38)  [unwired: 1 in]
              n812 = Build Array(w1707, w1706, w1705, w1704) -> (w1703:T39)
            }
            n813 = for {
              tunnel: w1671 -> [_] mode=indexing
              tunnel: w1670 -> [w1742]
              tunnel: w1669 -> [w1741]
              tunnel: w1668 -> [w1740]
              tunnel: w1667 -> [w1736]
              tunnel: w1666 -> [w1735]
              tunnel: [w1744] -> _ mode=indexing
              i -> [w1743]
              n814 = Index Array(array=w1741, index (row)=w1743) -> (element=w1737:dbl[])  [unwired: 1 in]
              n815 = Index Array(array=w1736, index (row)=w1743) -> (element=w1734:dbl[])  [unwired: 1 in]
              n816 = Index Array(array=w1735, index (row)=w1743) -> (element=w1733:dbl[])  [unwired: 1 in]
              n817 = Index Array(array=w1742, index (row)=w1743) -> (element=w1738:dbl[])  [unwired: 1 in]
              n818 = Index Array(array=w1740, index (row)=w1743) -> (element=w1739:timestamp[])  [unwired: 1 in]
              n819 = Bundle("Time"=w1739, "Motor X"=w1734) -> (w1747:cluster{"Time":timestamp[], "Motor X":dbl[]})  [unwired: 1 in]
              n820 = Bundle("Time"=w1739, "Motor Y"=w1733) -> (w1748:cluster{"Time":timestamp[], "Motor Y":dbl[]})  [unwired: 1 in]
              n821 = Bundle("Time"=w1739, "Offset X"=w1738) -> (w1746:cluster{"Time":timestamp[], "Offset X":dbl[]})  [unwired: 1 in]
              n822 = Bundle("Time"=w1739, "Offset Y"=w1737) -> (w1745:cluster{"Time":timestamp[], "Offset Y":dbl[]})  [unwired: 1 in]
              n823 = Build Array(w1745, w1746, w1747, w1748) -> (w1744:cluster{"Time":timestamp[], "Motor Y":dbl[]}[])
            }
            n824 = call <vilib>:"Add State(s) to Queue__jki_lib_state_machine.vi"("State(s) in (\"\")"=w1698) -> ("States Out"=w1697:string)  [unwired: 14 in]
            n825 = Index Array(array=w1659, index (row) #1=0 ("index (row)"), index (row) #2=1 ("index (row)"), index (row) #3=2 ("index (row)"), index (row) #4=3 ("index (row)"), index (row) #5=4 ("index (row)"), index (row) #6=5 ("index (row)"), index (row) #7=6 ("index (row)"), index (row) #8=7 ("index (row)"), index (row) #9=8 ("index (row)"), index (row) #10=9 ("index (row)"), index (row) #11=10 ("index (row)"), index (row) #12=11 ("index (row)")) -> (element #1=→"CCD 1":T39, element #2=→"CCD 2":T39, element #3=→"CCD 3":T39, element #4=→"CCD 4":T39, element #5=→"CCD 5":T39, element #6=→"CCD 6":T39, element #7=→"CCD 7":T39, element #8=→"CCD 8":T39, element #9=→"CCD 9":T39, element #10=→"CCD 10":T39, element #11=→"CCD 11":T39, element #12=→"CCD 12":T39)  [unwired: 12 in]
          }
          frame "newtdms" {
            # "Your code here.\n(You can make a copy of, or modify, this frame)"
            n826 = Unbundle By Name(w1785) -> ("Data Value Reference out"=w1773:refnum<k34>, "active cams"=w1768:string[])
            n827 = TDMS Close(8:w1783, 11:w1773) -> (0:w1767:errorcluster)  [unwired: 1 out]
            n828 = Get Date/Time In Seconds() -> (seconds since 1Jan1904=w1761:timestamp)
            n829 = call <vilib>:"Clear Errors.vi"("error in (no error)"=w1767) -> ("error out"=w1754:errorcluster)  [unwired: 6 in]
            n830 = Format Date/Time String(time format string (%c)="%Y%m%d", seconds (now)=w1761) -> (date/time string=w1762:string)  [unwired: 1 in]
            n831 = Format Date/Time String(time format string (%c)="%Y%m%d%H%M", seconds (now)=w1761) -> (date/time string=w1759:string)  [unwired: 1 in]
            n832 = property on="new tdms" class="Bool (strict)"("Value"=FALSE ("new tdms")) -> ()  [unwired: 2 in, 2 out]
            n833 = Get Date/Time In Seconds() -> (seconds since 1Jan1904=w1782:timestamp)
            n834 = Format Date/Time String(time format string (%c)="%Y%m%d%H%M", seconds (now)=w1782) -> (date/time string=w1774:string)  [unwired: 1 in]
            n835 = Build Path(base path=w1755, name or relative path=w1762) -> (appended path=w1763:path)
            n836 = Concatenate Strings(w1774, "Beampointingbooster_PICO.tdms" ("string")) -> (w1780:string)
            n837 = String To Path(string=w1780) -> ()  [unwired: 1 out]
            n838 = Concatenate Strings(w1759, "Beampointingbooster_PICO.tdms" ("string")) -> (w1757:string)
            n839 = String To Path(string=w1757) -> (path=w1752:path)
            n840 = call <vilib>:"Check if File or Folder Exists.vi"("error in (no error)"=w1754, "path"=w1763) -> ("error out"=w1766:errorcluster, "file or folder exists?"=w1764:bool, "dup path"=w1765:path)  [unwired: 7 in]
            n841 = case shown="False" w1764 {
              tunnel: w1765 -> [w1791 w1793]
              tunnel: [w1790 w1793] -> w1751
              tunnel: w1766 -> [w1789 w1792]
              tunnel: [w1788 w1792] -> w1753
              frame False {
                n842 = Create Folder(path (use dialog)=w1791, error in=w1789) -> (created path=w1790:path, error out=w1788:errorcluster)  [unwired: 1 in, 1 out]
              }
              frame True {
              }
            }
            n843 = call <vilib>:"Add State(s) to Queue__jki_lib_state_machine.vi"("State(s) in (\"\")"=w1787) -> ("States Out"=w1786:string)  [unwired: 14 in]
            n844 = Build Path(base path=w1751, name or relative path=w1752) -> (appended path=w1775:path)
            n845 = TDMS Open(6:FALSE ("disable buffering (T)"), 7:enum16{"1.0", "2.0"}."2.0" ("file format version (2.0)"), 8:w1753, 10:T16."create or replace" ("operation"), 11:w1775) -> (0:w1771:errorcluster, 3:w1770:refnum<k34>)  [unwired: 2 in]
            n846 = call "TDMSbuffersize.vi"("error in (no error)"=w1771, "group names"=w1768, "Data Value Reference in"=w1770) -> ("error out"=w1750:errorcluster, "Data Value Reference out"=w1769:refnum<k34>)  [unwired: 7 in]
            n847 = Bundle By Name(cluster=w1785, "Data Value Reference out"=w1769) -> (w1784:T36)
            n848 = call <vilib>:"Clear Errors.vi"("error in (no error)"=w1750) -> ("error out"=w1749:errorcluster)  [unwired: 6 in]
          }
          frame "Center" {
            # "Your code here.\n(You can make a copy of, or modify, this frame)"
            n849 = control-ref of="image::1"() -> (w1808:refnum<vi>)
            n850 = control-ref of="image::2"() -> (w1807:refnum<vi>)
            n851 = control-ref of="image::3"() -> (w1806:refnum<vi>)
            n852 = control-ref of="image::4"() -> (w1805:refnum<vi>)
            n853 = control-ref of="image::5"() -> (w1804:refnum<vi>)
            n854 = control-ref of="image::6"() -> (w1803:refnum<vi>)
            n855 = control-ref of="image::7"() -> (w1802:refnum<vi>)
            n856 = control-ref of="image::8"() -> (w1801:refnum<vi>)
            n857 = control-ref of="image::9"() -> (w1800:refnum<vi>)
            n858 = control-ref of="image::10"() -> (w1799:refnum<vi>)
            n859 = control-ref of="image::11"() -> (w1798:refnum<vi>)
            n860 = control-ref of="image::12"() -> (w1797:refnum<vi>)
            n861 = for {
              tunnel: [w1817] -> w1796 mode=indexing
              tunnel: w1795 -> [w1816] mode=indexing
              n862 = Unbundle By Name(w1816) -> ("Target.X::12"=w1815:refnum<vi>, "Target.Y::12"=w1814:refnum<vi>)
              n863 = property class="DigNum (strict)"(reference=w1815) -> ("Value"=w1818:dbl)  [unwired: 1 in, 2 out]
              n864 = property class="DigNum (strict)"(reference=w1814) -> ("Value"=w1819:dbl)  [unwired: 1 in, 2 out]
              n865 = Bundle("Value"=w1818, "Value"=w1819) -> (w1817:cluster{"Value":dbl, "Value":dbl})  [unwired: 1 in]
            }
            n866 = call <vilib>:"Add State(s) to Queue__jki_lib_state_machine.vi"("State(s) in (\"\")"=w1813) -> ("States Out"=w1812:string)  [unwired: 14 in]
            n867 = Build Array(w1808, w1807, w1806, w1805, w1804, w1803, w1802, w1801, w1800, w1799, w1798, w1797) -> (w1809:refnum<vi>[])
            n868 = for {
              tunnel: w1809 -> [w1821] mode=indexing
              tunnel: w1796 -> [w1820] mode=indexing
              n869 = property class="ImageControl"(reference=w1821, "Image Center Position"=w1820) -> ()  [unwired: 1 in, 2 out]
            }
            n870 = property on="Center" class="Bool (strict)"("Value"=FALSE ("Center")) -> ()  [unwired: 2 in, 2 out]
          }
          frame "ImgToAvg" {
            n871 = Decimal String To Number(string=w1828) -> (number=w1825:i32)  [unwired: 2 in, 1 out]
            n872 = Bundle By Name(cluster=w1827, "img to avg"=w1825) -> (w1826:T36)
            n873 = call <vilib>:"Add State(s) to Queue__jki_lib_state_machine.vi"("State(s) in (\"\")"=w1824) -> ("States Out"=w1823:string)  [unwired: 14 in]
          }
          frame "history" {
            # "Your code here.\n(You can make a copy of, or modify, this frame)"
            n874 = Unbundle By Name(w1838) -> ("Offset X"=w1844:dbl[][], "Offset Y"=w1843:dbl[][], "Mean Centroid X"=w1842:dbl[][], "Mean Centroid Y"=w1841:dbl[][], "Motor X"=w1840:dbl[][], "Motor Y"=w1839:dbl[][], "Time"=w1830:timestamp[][])
            n875 = for {
              tunnel: w1844 -> [w1862] mode=indexing
              tunnel: w1843 -> [w1860] mode=indexing
              tunnel: w1842 -> [w1859] mode=indexing
              tunnel: w1841 -> [w1858] mode=indexing
              tunnel: w1840 -> [w1857] mode=indexing
              tunnel: w1839 -> [w1856] mode=indexing
              tunnel: [w1861] -> w1836 mode=indexing
              tunnel: [w1855] -> w1835 mode=indexing
              tunnel: [w1851] -> w1834 mode=indexing
              tunnel: [w1854] -> w1833 mode=indexing
              tunnel: [w1853] -> w1832 mode=indexing
              tunnel: [w1852] -> w1831 mode=indexing
              tunnel: w1830 -> [w1850] mode=indexing
              tunnel: [w1848] -> w1829 mode=indexing
              w1849 = 0
              n876 = Delete From Array(array=w1857, index=w1849) -> (array with subset deleted=w1853:dbl[])  [unwired: 1 in, 1 out]
              n877 = Delete From Array(array=w1856, index=w1849) -> (array with subset deleted=w1852:dbl[])  [unwired: 1 in, 1 out]
              n878 = Delete From Array(array=w1850, index=w1849) -> (array with subset deleted=w1848:timestamp[])  [unwired: 1 in, 1 out]
              n879 = Delete From Array(array=w1859, index=w1849) -> (array with subset deleted=w1851:dbl[])  [unwired: 1 in, 1 out]
              n880 = Delete From Array(array=w1858, index=w1849) -> (array with subset deleted=w1854:dbl[])  [unwired: 1 in, 1 out]
              n881 = Delete From Array(array=w1860, index=w1849) -> (array with subset deleted=w1855:dbl[])  [unwired: 1 in, 1 out]
              n882 = Delete From Array(array=w1862, index=w1849) -> (array with subset deleted=w1861:dbl[])  [unwired: 1 in, 1 out]
            }
            n883 = call <vilib>:"Add State(s) to Queue__jki_lib_state_machine.vi"("State(s) in (\"\")"=w1847) -> ("States Out"=w1846:string)  [unwired: 14 in]
            n884 = Bundle By Name(cluster=w1838, "Offset X"=w1836, "Offset Y"=w1835, "Mean Centroid X"=w1834, "Mean Centroid Y"=w1833, "Motor X"=w1832, "Motor Y"=w1831, "Time"=w1829) -> (w1837:T36)
          }
        }
        n885 = property on="Box" class="Arr (strict)"() -> ("Value"=w134:T6)  [unwired: 2 in, 2 out]
        n886 = for {
          tunnel: w136 -> [w157]
          tunnel: w135 -> [w158]
          tunnel: w132 -> [w150] mode=indexing
          tunnel: w134 -> [w151] mode=indexing
          n887 = call-poly <userlib>:"Filter 1D Array__ogtk.vi"("items to filter"=w150, "array"=w158) -> ("filtered item indices"=w159:i32[])  [unwired: 4 in, 1 out]
          n888 = Index Array(array=w159) -> (element=w153:i32)  [unwired: 1 in]
          n889 = Index Array(array=w157, index=w153) -> (element=w156:T30)
          n890 = Unbundle By Name(w156) -> ("Target.X::12"=w161:refnum<vi>, "Target.Y::12"=w160:refnum<vi>)
          n891 = property class="DigNum (strict)"(reference=w161) -> ("Value"=w155:dbl)  [unwired: 1 in, 2 out]
          n892 = property class="DigNum (strict)"(reference=w160) -> ("Value"=w154:dbl)  [unwired: 1 in, 2 out]
          n893 = call "draw crosshair imaq.vi"("Color"=u32 16774656, "Target.Y"=w154, "size"=cluster{"xhair size":dbl, "xhair size 2":dbl} {"xhair size"=25.0, "xhair size 2"=25.0}, "Target.X"=w155, "Bounding Rectangle"=T14 {"Left"=0, "Top"=0, "Right"=0, "Bottom"=0}, "image in"=w150) -> ("image out"=w149:T9)  [unwired: 4 in, 1 out]
          n894 = call "draw box imaq.vi"("Color"=u32 1244928, "Rectangle"=w151, "image in"=w149) -> ()  [unwired: 7 in, 2 out]
        }
      }
      n895 = control-ref of="This Application"() -> (w121:refnum<vi>)
      n896 = control-ref of="This VI"() -> (w125:refnum<vi>)
      n897 = Current VI's Menubar() -> (w124:refnum<k9>)
      n898 = call "GUI_Master_subvi_reentrant_queues.vi"("This Application"=w121, "error in (no error)"=w122, "tcp data event"=w120, "Caller menu reference"=w124, "Caller VI ref"=w125) -> ("error out"=→"error IO 2":errorcluster)  [unwired: 6 in]
      n899 = Unbundle By Name(w66) -> ("Data Value Reference out"=w65:refnum<k34>)
      n900 = for {
        tunnel: w95 -> [w129] mode=indexing
        tunnel: w94 -> [w128]
        tunnel: [w127] -> w64
        n901 = call "IMAQ Dispose"("Image"=w129, "error in (no error)"=w128) -> ("error out"=w127:errorcluster)  [unwired: 4 in]
      }
      n902 = TDMS Close(8:w64, 11:w65) -> (0:→"error out 2":errorcluster)  [unwired: 1 out]
      "Names" <- w34
    }
  }
